vi "Text control 2 v6.1_pump-specific.vi"() -> ()   [LabVIEW 2016]
panel:
  in  "Tab Control":enum32{"Main", "Other parameters"}(tab)
  out "Line running":i32
  out "Total lines":i32
  out "Path":path=path "C:/users/rlp38/09Apr2009LTtesting/test2.txt"
  out "I vs Vg":cluster{"Y data in":dbl[], "X data in":dbl[]}[](graph)
  out "Is max":dbl format="%.2e"
  out "Id max":dbl format="%.2e"
  out "Ig max":dbl format="%.2e"
  out "Imax vs time":cluster{"Y data in":dbl[], "X data in":dbl[]}[](graph)
  out "Imin vs time":cluster{"Y data in":dbl[], "X data in":dbl[]}[](graph)
  out "I vs Vd":cluster{"Y data in":dbl[], "X data in":dbl[]}[](graph)
  in  "Script":string="#-------------------------------------------------------\n# SPM pump cleaning script\n#\n# Version 0.5\n# Author: Dimitrios Simatos\n# Last updated: 2018-01-05\n#-------------------------------------------------------\n# Description\n#\n# This script is designed to run the cleaning sequence of the SPM OEM pump.\n# This script needs to be run 4 times!\n#-------------------------------------------------------\n# Changes\n#\n# Placed initialization and hard stop commands in the beginning.\n#-------------------------------------------------------\n# Important points\n#\n# Never leave any liquid in the pump to dry after the experiments. If they dry, the residue may block the valve.\n# Always run the cleaning cycle after the experiments.\n# Use clockwise rotation when going up in valve port numbers and vice versa.\n#-------------------------------------------------------\n# Things to do before running the script\n#\n# Set time units to minutes.\n# Set filenames.\n# Replace the tubing, if necessary.\n#-------------------------------------------------------\n# Port connections\n#\n# Port 1: Waste\n# Port 2: Waste\n# Port 3: Various cleaning liquids\n# Port 4: Waste\n# Port 5: Waste\n# Port 6: Waste\n#\n# Between each of the 4 runs, the settings of Port 3 will change, according to the cleaning protocol.\n# The settings for Port 3 are:\n# 1st run: 1% v/v solution of sodium hypochlorite in ultrapure water\n# 2nd run: 0.1% w/v solution of sodium dodecyl sulfate in ultrapure water\n# 3rd run: Ultrapure water\n# 4th run: Waste (in air, not immersed in liquid)\n#-------------------------------------------------------\n# Cleaning protocol for the SPM OEM pump (from the manual)\n#\n# A cleaning procedure should be performed at the end of each day or in between two different experiments.\n# An effective cleaning can be performed in the following manner:\n# • Bleach solution to kill microorganisms\n# 1. Prepare a solution of 1% chlorine bleach and deionized water\n#    NOTE: Prepare a 1% v/v solution of sodium hypochlorite in deionized water\n# 2. Prepare a reservoir and place 1 tubing in the bleach solution and 5 tubings in a waste recipient\n# 3. Pick up the bleach solution through 1 port to entirely fill the syringe\n# 4. Sequentially output the syringe content through the remaining ports and throw it to the waste\n# 5. Repeat operation at least 2 times\n# • Detergent solution to remove debris\n# 1. Prepare a solution of 0.1% detergent and deionized water\n#    NOTE: Prepare a 0.1% w/v solution of sodium dodecyl sulfate in deionized water\n# 2. Move the tubing from the bleach solution reservoir and place it into a reservoir of detergent solution\n# 3. Pick up the detergent solution through 1 port to entirely fill the syringe\n# 4. Sequentially output the detergent solution through the remaining ports into the waste recipient\n# 5. Repeat operation at least 2 times\n# • Rinsing water to prepare the pump for your next experiment\n# 1. Move the tubing from the detergent solution reservoir and place it into a reservoir of deionized water\n# 2. Pick up the rinsing solution through 1 port to entirely fill the syringe\n# 3. Sequentially output the rinse water through the remaining ports into the waste recipient\n# 4. Repeat operation at least 2 times\n# • Replace the tubing, if necessary\n#-------------------------------------------------------\n# Pumping cycles and execution time\n#\n# Execution time for a single cycle: 6 x (1 min + 10 sec) = 7 minutes\n# Total execution time: 4 x 7 = 28 minutes\n# Since the script has to run 4 times, the cleaning lasts for: 4 x 28 = 112 minutes\n# Air must be the last to be pumped through the valve, to remove all liquids.\n# There are 4 pumping cycles. Each one draws a different liquid through port 3 and pumps it sequentially through ports 1,2,4,5,6.\n# During the sequential pumping, each port receives 200 ml of liquid (20% of the total syringe volume = 600 \"plunger units\")\n# The device must be disconnected from the port during the cleaning procedure.\n# All cycles are similar, except cycle 1 has the initialization command uncommented and the first report valve command commented.\n#-------------------------------------------------------\n# Volume of liquid needed\n#\n# Volume of liquid needed per cycle: 1 ml\n# Total volume of liquid needed per script run: 4 x 1 = 4 ml\n# Since the script has to run 4 times, the first 3 with different liquids, I need:\n# 4 ml of 1% v/v solution of sodium hypochlorite in ultrapure water\n# 4 ml of 0.1% w/v solution of sodium dodecyl sulfate in ultrapure water\n# 4 ml of ultrapure water\n#-------------------------------------------------------\n# Parameters\n#\n# Syringe size: 1 ml\n# Step resolution N = 0.01 mm\n# Drawing flow V = 300 pulses/second (6000 ul/min)\n# Pumping flow V = 300 pulses/second (6000 ul/min)\n#-------------------------------------------------------\n# Pump initialization\npump /1T #hard stop pump\npump /1ZR #initialize pump\n#-------------------------------------------------------\n# Cycle 1\n# Fill the syringe\npump /1Q #query pump\npump /1? #report absolute plunger position\n#pump /1?6 #report valve position\nwait-min 1 #wait 1 minute\npump /1N0R #set step resolution: 0.01 mm\npump /1Q #query pump\npump /1? #report absolute plunger position (the plunger should be at 0)\npump /1?6 #report valve position\nwait 1000 #wait 1 second\npump /1V300R #choose speed: 300 steps/s (6000 ul/min)\npump /1Q #query pump\nwait 1000 #wait 1 second\npump /1I3R #go to port 3, clockwise rotation\npump /1Q #query pump\npump /1?6 #report valve position\nwait 1000 #wait 1 second\npump /1A3000R #go to absolute position 3000 (= draw 1 ml)\nwait 30000 #wait 30 seconds\npump /1Q #query pump\npump /1? #report absolute plunger position (the plunger should have finished moving)\n#pump /1?6 #report valve position\n# The sequential pumping begins\n# Port 1\npump /1O1R #switch to port 1, counterclockwise rotation\npump /1Q #query pump\npump /1?6 #report valve position\npump /1A2400R #go to absolute position 2400 (= pump 200 ul)\npump /1Q #query pump\npump /1? #report absolute plunger position (the plunger should be moving to 0)\nwait-min 1 #wait 1 minute\npump /1? #report absolute plunger position (the plunger should have finished moving)\n# Port 2\npump /1I2R #switch to port 2, clockwise rotation\npump /1Q #query pump\npump /1?6 #report valve position\npump /1A1800R #go to absolute position 1800 (= pump 200 ul)\npump /1Q #query pump\npump /1? #report absolute plunger position (the plunger should be moving to 0)\nwait-min 1 #wait 1 minute\npump /1? #report absolute plunger position (the plunger should have finished moving)\n# Port 4\npump /1I4R #switch to port 4, clockwise rotation\npump /1Q #query pump\npump /1?6 #report valve position\npump /1A1200R #go to absolute position 1200 (= pump 200 ul)\npump /1Q #query pump\npump /1? #report absolute plunger position (the plunger should be moving to 0)\nwait-min 1 #wait 1 minute\npump /1? #report absolute plunger position (the plunger should have finished moving)\n# Port 5\npump /1I5R #switch to port 5, clockwise rotation\npump /1Q #query pump\npump /1?6 #report valve position\npump /1A600R #go to absolute position 600 (= pump 200 ul)\npump /1Q #query pump\npump /1? #report absolute plunger position (the plunger should be moving to 0)\nwait-min 1 #wait 1 minute\npump /1? #report absolute plunger position (the plunger should have finished moving)\n# Port 6\npump /1I6R #switch to port 6, clockwise rotation\npump /1Q #query pump\npump /1?6 #report valve position\npump /1A0R #go to absolute position 0 (= pump 200 ul)\npump /1Q #query pump\npump /1? #report absolute plunger position (the plunger should be moving to 0)\nwait-min 1 #wait 1 minute\npump /1? #report absolute plunger position (the plunger should have finished moving)\n#-------------------------------------------------------\n# Cycle 2\n# Fill the syringe\n#pump /1ZR #initialize pump\npump /1Q #query pump\npump /1? #report absolute plunger position\npump /1?6 #report valve position\nwait-min 1 #wait 1 minute\npump /1N0R #set step resolution: 0.01 mm\npump /1Q #query pump\npump /1? #report absolute plunger position (the plunger should be at 0)\npump /1?6 #report valve position\nwait 1000 #wait 1 second\npump /1V300R #choose speed: 300 steps/s (6000 ul/min)\npump /1Q #query pump\nwait 1000 #wait 1 second\npump /1O3R #go to port 3, counterclockwise rotation\npump /1Q #query pump\npump /1?6 #report valve position\nwait 1000 #wait 1 second\npump /1A3000R #go to absolute position 3000 (= draw 1 ml)\nwait 30000 #wait 30 seconds\npump /1Q #query pump\npump /1? #report absolute plunger position (the plunger should have finished moving)\n#pump /1?6 #report valve position\n# The sequential pumping begins\n# Port 1\npump /1O1R #switch to port 1, counterclockwise rotation\npump /1Q #query pump\npump /1?6 #report valve position\npump /1A2400R #go to absolute position 2400 (= pump 200 ul)\npump /1Q #query pump\npump /1? #report absolute plunger position (the plunger should be moving to 0)\nwait-min 1 #wait 1 minute\npump /1? #report absolute plunger position (the plunger should have finished moving)\n# Port 2\npump /1I2R #switch to port 2, clockwise rotation\npump /1Q #query pump\npump /1?6 #report valve position\npump /1A1800R #go to absolute position 1800 (= pump 200 ul)\npump /1Q #query pump\npump /1? #report absolute plunger position (the plunger should be moving to 0)\nwait-min 1 #wait 1 minute\npump /1? #report absolute plunger position (the plunger should have finished moving)\n# Port 4\npump /1I4R #switch to port 4, clockwise rotation\npump /1Q #query pump\npump /1?6 #report valve position\npump /1A1200R #go to absolute position 1200 (= pump 200 ul)\npump /1Q #query pump\npump /1? #report absolute plunger position (the plunger should be moving to 0)\nwait-min 1 #wait 1 minute\npump /1? #report absolute plunger position (the plunger should have finished moving)\n# Port 5\npump /1I5R #switch to port 5, clockwise rotation\npump /1Q #query pump\npump /1?6 #report valve position\npump /1A600R #go to absolute position 600 (= pump 200 ul)\npump /1Q #query pump\npump /1? #report absolute plunger position (the plunger should be moving to 0)\nwait-min 1 #wait 1 minute\npump /1? #report absolute plunger position (the plunger should have finished moving)\n# Port 6\npump /1I6R #switch to port 6, clockwise rotation\npump /1Q #query pump\npump /1?6 #report valve position\npump /1A0R #go to absolute position 0 (= pump 200 ul)\npump /1Q #query pump\npump /1? #report absolute plunger position (the plunger should be moving to 0)\nwait-min 1 #wait 1 minute\npump /1? #report absolute plunger position (the plunger should have finished moving)\n#-------------------------------------------------------\n# Cycle 3\n# Fill the syringe\n#pump /1ZR #initialize pump\npump /1Q #query pump\npump /1? #report absolute plunger position\npump /1?6 #report valve position\nwait-min 1 #wait 1 minute\npump /1N0R #set step resolution: 0.01 mm\npump /1Q #query pump\npump /1? #report absolute plunger position (the plunger should be at 0)\npump /1?6 #report valve position\nwait 1000 #wait 1 second\npump /1V300R #choose speed: 300 steps/s (6000 ul/min)\npump /1Q #query pump\nwait 1000 #wait 1 second\npump /1O3R #go to port 3, counterclockwise rotation\npump /1Q #query pump\npump /1?6 #report valve position\nwait 1000 #wait 1 second\npump /1A3000R #go to absolute position 3000 (= draw 1 ml)\nwait 30000 #wait 30 seconds\npump /1Q #query pump\npump /1? #report absolute plunger position (the plunger should have finished moving)\n#pump /1?6 #report valve position\n# The sequential pumping begins\n# Port 1\npump /1O1R #switch to port 1, counterclockwise rotation\npump /1Q #query pump\npump /1?6 #report valve position\npump /1A2400R #go to absolute position 2400 (= pump 200 ul)\npump /1Q #query pump\npump /1? #report absolute plunger position (the plunger should be moving to 0)\nwait-min 1 #wait 1 minute\npump /1? #report absolute plunger position (the plunger should have finished moving)\n# Port 2\npump /1I2R #switch to port 2, clockwise rotation\npump /1Q #query pump\npump /1?6 #report valve position\npump /1A1800R #go to absolute position 1800 (= pump 200 ul)\npump /1Q #query pump\npump /1? #report absolute plunger position (the plunger should be moving to 0)\nwait-min 1 #wait 1 minute\npump /1? #report absolute plunger position (the plunger should have finished moving)\n# Port 4\npump /1I4R #switch to port 4, clockwise rotation\npump /1Q #query pump\npump /1?6 #report valve position\npump /1A1200R #go to absolute position 1200 (= pump 200 ul)\npump /1Q #query pump\npump /1? #report absolute plunger position (the plunger should be moving to 0)\nwait-min 1 #wait 1 minute\npump /1? #report absolute plunger position (the plunger should have finished moving)\n# Port 5\npump /1I5R #switch to port 5, clockwise rotation\npump /1Q #query pump\npump /1?6 #report valve position\npump /1A600R #go to absolute position 600 (= pump 200 ul)\npump /1Q #query pump\npump /1? #report absolute plunger position (the plunger should be moving to 0)\nwait-min 1 #wait 1 minute\npump /1? #report absolute plunger position (the plunger should have finished moving)\n# Port 6\npump /1I6R #switch to port 6, clockwise rotation\npump /1Q #query pump\npump /1?6 #report valve position\npump /1A0R #go to absolute position 0 (= pump 200 ul)\npump /1Q #query pump\npump /1? #report absolute plunger position (the plunger should be moving to 0)\nwait-min 1 #wait 1 minute\npump /1? #report absolute plunger position (the plunger should have finished moving)\n#-------------------------------------------------------\n# Cycle 4\n# Fill the syringe\n#pump /1ZR #initialize pump\npump /1Q #query pump\npump /1? #report absolute plunger position\npump /1?6 #report valve position\nwait-min 1 #wait 1 minute\npump /1N0R #set step resolution: 0.01 mm\npump /1Q #query pump\npump /1? #report absolute plunger position (the plunger should be at 0)\npump /1?6 #report valve position\nwait 1000 #wait 1 second\npump /1V300R #choose speed: 300 steps/s (6000 ul/min)\npump /1Q #query pump\nwait 1000 #wait 1 second\npump /1O3R #go to port 3, counterclockwise rotation\npump /1Q #query pump\npump /1?6 #report valve position\nwait 1000 #wait 1 second\npump /1A3000R #go to absolute position 3000 (= draw 1 ml)\nwait 30000 #wait 30 seconds\npump /1Q #query pump\npump /1? #report absolute plunger position (the plunger should have finished moving)\n#pump /1?6 #report valve position\n# The sequential pumping begins\n# Port 1\npump /1O1R #switch to port 1, counterclockwise rotation\npump /1Q #query pump\npump /1?6 #report valve position\npump /1A2400R #go to absolute position 2400 (= pump 200 ul)\npump /1Q #query pump\npump /1? #report absolute plunger position (the plunger should be moving to 0)\nwait-min 1 #wait 1 minute\npump /1? #report absolute plunger position (the plunger should have finished moving)\n# Port 2\npump /1I2R #switch to port 2, clockwise rotation\npump /1Q #query pump\npump /1?6 #report valve position\npump /1A1800R #go to absolute position 1800 (= pump 200 ul)\npump /1Q #query pump\npump /1? #report absolute plunger position (the plunger should be moving to 0)\nwait-min 1 #wait 1 minute\npump /1? #report absolute plunger position (the plunger should have finished moving)\n# Port 4\npump /1I4R #switch to port 4, clockwise rotation\npump /1Q #query pump\npump /1?6 #report valve position\npump /1A1200R #go to absolute position 1200 (= pump 200 ul)\npump /1Q #query pump\npump /1? #report absolute plunger position (the plunger should be moving to 0)\nwait-min 1 #wait 1 minute\npump /1? #report absolute plunger position (the plunger should have finished moving)\n# Port 5\npump /1I5R #switch to port 5, clockwise rotation\npump /1Q #query pump\npump /1?6 #report valve position\npump /1A600R #go to absolute position 600 (= pump 200 ul)\npump /1Q #query pump\npump /1? #report absolute plunger position (the plunger should be moving to 0)\nwait-min 1 #wait 1 minute\npump /1? #report absolute plunger position (the plunger should have finished moving)\n# Port 6\npump /1I6R #switch to port 6, clockwise rotation\npump /1Q #query pump\npump /1?6 #report valve position\npump /1A0R #go to absolute position 0 (= pump 200 ul)\npump /1Q #query pump\npump /1? #report absolute plunger position (the plunger should be moving to 0)\nwait-min 1 #wait 1 minute\npump /1? #report absolute plunger position (the plunger should have finished moving)\n#-------------------------------------------------------"
  out "Command running:":string
  out "Serial port data":string
  out "Elapsed Time":dbl caption="Elapsed Time (s)"
  in  "Time Units":u16(ring)=1 items=["Seconds", "Minutes", "Hours"]
  in  "Time Offset":dbl caption="Set Start Time (s)"
  in  "Reset":bool
  in  "Auto Reset":bool
  in  "integration time":u32(slide) max=2 step=1 scale=0.0..2.0
  in  "Interrupt run":bool
  out "Absolute plunger position vs time":cluster{"Y data in":dbl[], "X data in":dbl[]}[](graph)
  out "Valve position vs time":cluster{"Y data in":dbl[], "X data in":dbl[]}[](graph)
  out "Is on":dbl format="%.2e"
  out "Id on":dbl format="%.2e"
  out "Ig on":dbl format="%.2e"
  out "Ion vs time":cluster{"Y data in":dbl[], "X data in":dbl[]}[](graph)
  out "Ioff vs time":cluster{"Y data in":dbl[], "X data in":dbl[]}[](graph)
  out "Ig min":dbl format="%.2e"
  out "Id min":dbl format="%.2e"
  out "Is min":dbl format="%.2e"
  out "Is off":dbl format="%.2e"
  out "Id off":dbl format="%.2e"
  out "Ig off":dbl format="%.2e"
  in  "Integration time (long)":dbl=0.32 min=0.04 max=2.0 step=0.02 format="%.2f"
  in  "Integration time (short)":dbl=0.0019 min=8e-05 max=0.0019 step=8e-05 format="%^.0e"
  in  "Gate: Compliance":dbl=0.001 format="%.8f"
  in  "Drain: Compliance":dbl=0.001 format="%.8f"
  in  "Hard stop pump":bool
  in  "Halt pump":bool
  in  "Gate Range\nmode":u16(ring) items=["Auto", "Limited", "Fixed"]
  in  "Gate Range":u8(slide)=6 max=11 scale=0.0..11.0
  in  "Source/Drain\nRange mode":u16(ring) items=["Auto", "Limited", "Fixed"]
  in  "Source/Drain Range":u8(slide)=6 max=11 scale=0.0..11.0
  in  "Panel Controls":T1={"Emergency Stop"=refnum, "TransGraph Max"=1e-05, "Text/Graph (text=false)"=TRUE} {"TransGraph Max" format="%.2e"}
  in  "Panel Controls 2":T2={"Emergency Stop"=refnum, "TransGraph Max"=1e-05, "Text/Graph (text=false)"=TRUE, "TransGraph Min"=1e-11} {"TransGraph Min" format="%.2e"; "TransGraph Max" format="%.2e"}
  in  "SMU4":cluster{"on/off":bool, "Voltage":dbl} {"Voltage" min=-100.0 max=100.0 format="%.2f"}
  in  "Full Reset":bool
  in  "Standby":T3
  out "error out":errorcluster
  in  "Delay before read (ms)":u32=1000
  in  "byte count":u32=64
  in  "Serial End Mode for Reads":u16(ring)=2 items=["None", "LastBit", "TermChar"]
  in  "Timeout (ms)":u32=10000
  in  "Enable Termination\nChar (T)":bool=TRUE
  in  "Termination char\n(0xA = '\\n' = LF)\n(0xD = '\\r' = CR)":u8=13 format="%.0x"
  in  "flow control":u16(ring) items=["None"=0, "XON/XOFF"=1, "RTS/CTS"=2, "DTR/DSR"=4]
  in  "stop bits":u16(ring)=10 items=["1.0"=10, "1.5"=15, "2.0"=20]
  in  "parity":u16(ring) items=["None", "Odd", "Even", "Mark", "Space"]
  in  "data bits":u16=8 min=5 max=8 step=1
  in  "VISA resource name":refnum<visa-resource-name>="COM6"
  in  "baud rate":u32=9600
  in  "Filename (variable part)":string="step_1_up-H2O_initial_"
  in  "Suffix (script)":string="step_1_up-H2O_initial_script.txt"
  out "Timings Indicator":T4
  in  "Timings (overwritten by the Front Panel)":T5={"integration time"=0, "Short/Long integration time"=0.00064, "hold time (sec)"=0.0, "delay time (sec)"=0.0, "Step Time (0 disables)"=0.0, "sweep method"=0, "Pulse period"=0.005, "Base voltage"=0.0, "Pulse width"=0.0005} {"Pulse width" min=0.0005 max=0.1 step=0.0001 format="%.4f"; "Base voltage" format="%^.4e"; "Pulse period" min=0.005 max=1.0 step=0.0001 format="%.4f"; "sweep method" items=["Continuous", "Pulsed"]; "Step Time (0 disables)" format="%.2f"; "delay time (sec)" format="%.4f"; "hold time (sec)" format="%.4f"; "Short/Long integration time" format="%^.0e"; "integration time" scale=0.0..2.0}
  in  "Gate":T6={"Gate Start"=0.0, "Gate Stop"=2.0, "Gate Step (linear only)"=1.0, "Gate Compliance"=0.0001, "Gate PComp"=0.0, "Range mode"=0, "Range"=6} {"Range" max=11 scale=0.0..11.0; "Range mode" items=["Auto", "Limited", "Fixed"]; "Gate PComp" format="%^.2e"; "Gate Compliance" format="%^.2e"; "Gate Step (linear only)" format="%^.4e"; "Gate Stop" format="%^.4e"; "Gate Start" format="%^.4e"}
  in  "Drain 2":T7={"Drain Start"=0.0, "Drain Stop"=2.0, "Drain Compliance"=0.0001, "Drain Step"=1.0, "Drain PComp"=0.0, "Range mode"=0, "Range"=6} {"Range" max=11 scale=0.0..11.0; "Range mode" items=["Auto", "Limited", "Fixed"]; "Drain PComp" format="%^.2e"; "Drain Step" format="%^.4e"; "Drain Compliance" format="%^.2e"; "Drain Stop" format="%^.4e"; "Drain Start" format="%^.4e"}
  # "Syntax:\nitime [s|m|l] time(sec): [s|m|l] determines the integration time setting (small|medium|long) and time sets the value.\nNOTE: The value of the integration time has to be within the range allowed by its category (s|m|l), otherwise, the closest value will be used. (e.g. if the category is set to short but the time value is very long, the actual value used will be the maximum short integration time.\nIntegration times:\n    Short: Default: 640 us. Range: 8E-5 - 1.92E-3 seconds.\n    Medium: Fixed at 1 NPL cycle (0.02 seconds).\n    Long: Default: 16 NPL cycles (0.32 seconds). Range: 2-100 NPL cycles (0.04 seconds - 2 seconds).\ngaterangemode [a|l|f]\ndrainrangemode [a|l|f]\npulsed [on|off] PulsePeriod(sec) PulseBaseVoltage PulseONWidth(sec)\nstandby [on l off]\nwait NumMilliseconds\nwait-min NumMinutes\n# texthere = comment\ntransfer [s|d] VgStart VgStop VgStep VdStart VdStop VdStep\noutput [s|d] VgStart VgStop VgStep VdStart VdStop VdStep\nsample Vg Vd NumSamples Time(s) SampleInterval(s)\nsamplei Idg NumSamples Time(s) SampleInterval(s) VDGcompliance\n100 samples is approximately 13 seconds with medium integration\n# if in doubt use SampleInterval(s) = 0.004\nstressV VG VD IGcompliance IDcompliance Duration(sec)\nstressI IDG VDGcompliance Duration(sec)\nvsu2pulse Bias Duration(s)\npulsedstressV [s|d] VEstop VgON VgOFF Period(s) PulseONwidth(s) Vd\nsample-fpp Vg Vd NumSamples Time\nresample-fpp Vg Vd\ntransfer-fpp [s|d] VgStart VgStop VgStep VdStart VdStop VdStep\noutput-fpp [s|d] VgStart VgStop VgStep VdStart VdStop VdStep\nserial SerialPortCommand\npump SerialPortCommand for the SPM pump\n\nSPM Pump Syntax (<x>: pump number, use 1 if only one pump):\nif the command syntax contains [R], then append the letter R to the command\n/<x>Q: query (a query command should follow each command)\n/<x>Z[R] or /<x>Y[R]: initialize pump\n/<x>N<n>[R] (<n>=0,1): <0> (<1>) microstep 0.01 mm (0.00125 mm) resolution\n/<x>I<n> (<n>=0-6): turn to port number n (clockwise)\n/<x>O<n> (<n>=0-6): turn to port number n (counterclockwise)\n/<x>X: Re-execute last command string\n/<x>G<n>[R] (<n>=0-60000): repeat command sequence (default: 0, 0=loop forever)\n/<x>g: Mark the start of a repeat sequence (max = 10)\n/<x>M<n>[R] (<n>=0-86400000): delay command execution by n milliseconds\n/<x>H: Halt; Pause the sequence after finishing the current move\n/<x>T: Hardstop; Interrupt the current move and suppress it from the sequence\n/<x>A<n>[R] (<n>=0-3000 with N=0, 0-24000 with N=1): absolute position\n/<x>P<n>[R] (<n>=0-3000 with N=0, 0-24000 with N=1): relative pickup\n/<x>D<n>[R] (<n>=0-3000 with N=0, 0-24000 with N=1): relative dispense\n/<x>V<n>[R] (<n>=1-1600 default: 150): set peak speed (pulses/sec)\nNOTE: The lowest speed limit is 1 pulse/sec, not 5, as the manual states.\n/<x>S<n>[R] (<n>=10-40 default: 22): set speed (NOT in pulses/sec, look in manual)\nNOTE: When controlled with absolute position, one does not need to pay special attention to the syringe that is mounted on the pump.\nWithdraw from lower stage (ports 3, 5), dispense from higher stage (ports 2, 4, 6).\nConnect Port 1 to waste."
  # "Time"
  # "1\n2\n3\n4\n5\n6\n7\n8\n9\n10\n11\n12\n13\n14\n15\n16\n17\n18\n19\n20"
  # "Serial port settings"
  # "Filename settings"
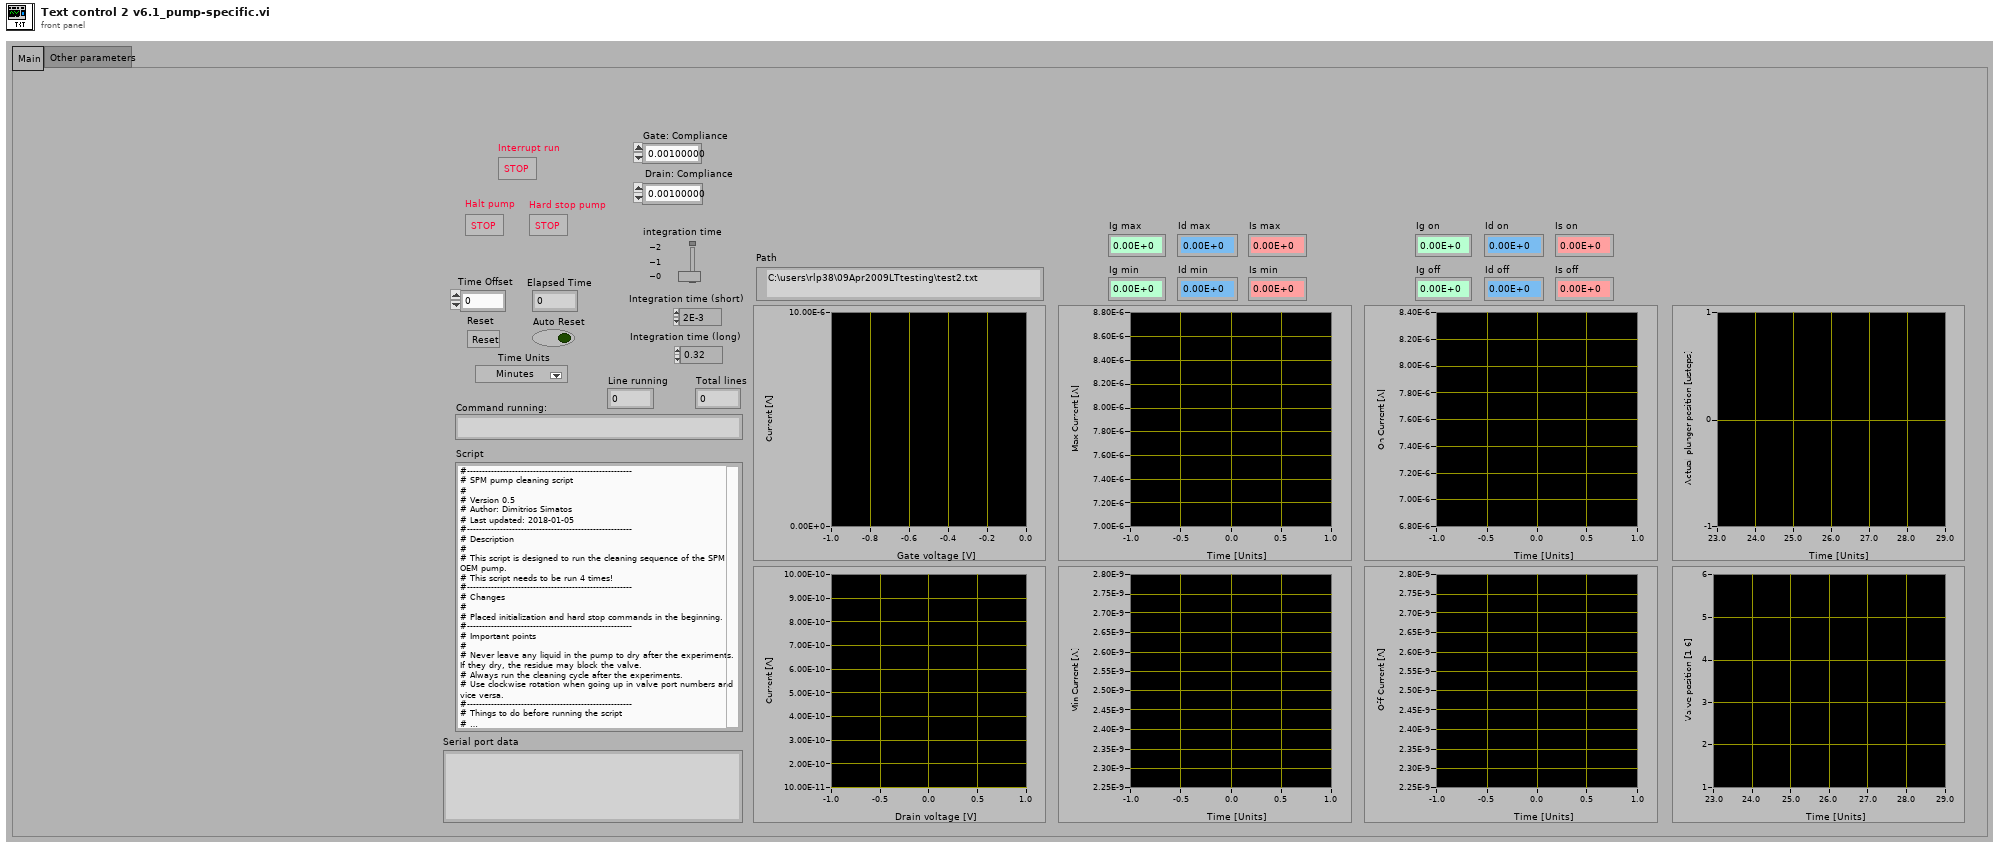
[diagram p1: front panel]
types:
  T1 = cluster{"Emergency Stop":refnum<vi>, "TransGraph Max":dbl, "Text/Graph (text=false)":bool}
  T2 = cluster{"Emergency Stop":refnum<vi>, "TransGraph Max":dbl, "Text/Graph (text=false)":bool, "TransGraph Min":dbl}
  T3 = cluster{"Gate Standby":bool, "Drain Standby":bool}
  T4 = cluster{"integration time (0:s, 1:m, 2:l)":u32, "Short/Long integration time":dbl, "hold time (sec)":dbl, "delay time (sec)":dbl, "Step Time (0 disables)":dbl, "sweep method":u16, "Pulse period":dbl, "Base voltage":dbl, "Pulse width":dbl}
  T5 = cluster{"integration time":u32, "Short/Long integration time":dbl, "hold time (sec)":dbl, "delay time (sec)":dbl, "Step Time (0 disables)":dbl, "sweep method":u16, "Pulse period":dbl, "Base voltage":dbl, "Pulse width":dbl}
  T6 = cluster{"Gate Start":dbl, "Gate Stop":dbl, "Gate Step (linear only)":dbl, "Gate Compliance":dbl, "Gate PComp":dbl, "Range mode":u16, "Range":u8}
  T7 = cluster{"Drain Start":dbl, "Drain Stop":dbl, "Drain Compliance":dbl, "Drain Step":dbl, "Drain PComp":dbl, "Range mode":u16, "Range":u8}
  T8 = enum16{"open", "replace", "create", "open or create", "replace or create", "replace or create with confirmation"}
  T9 = cluster{"V2 Start":dbl, "V2 Step":dbl, "Number of points":i32}
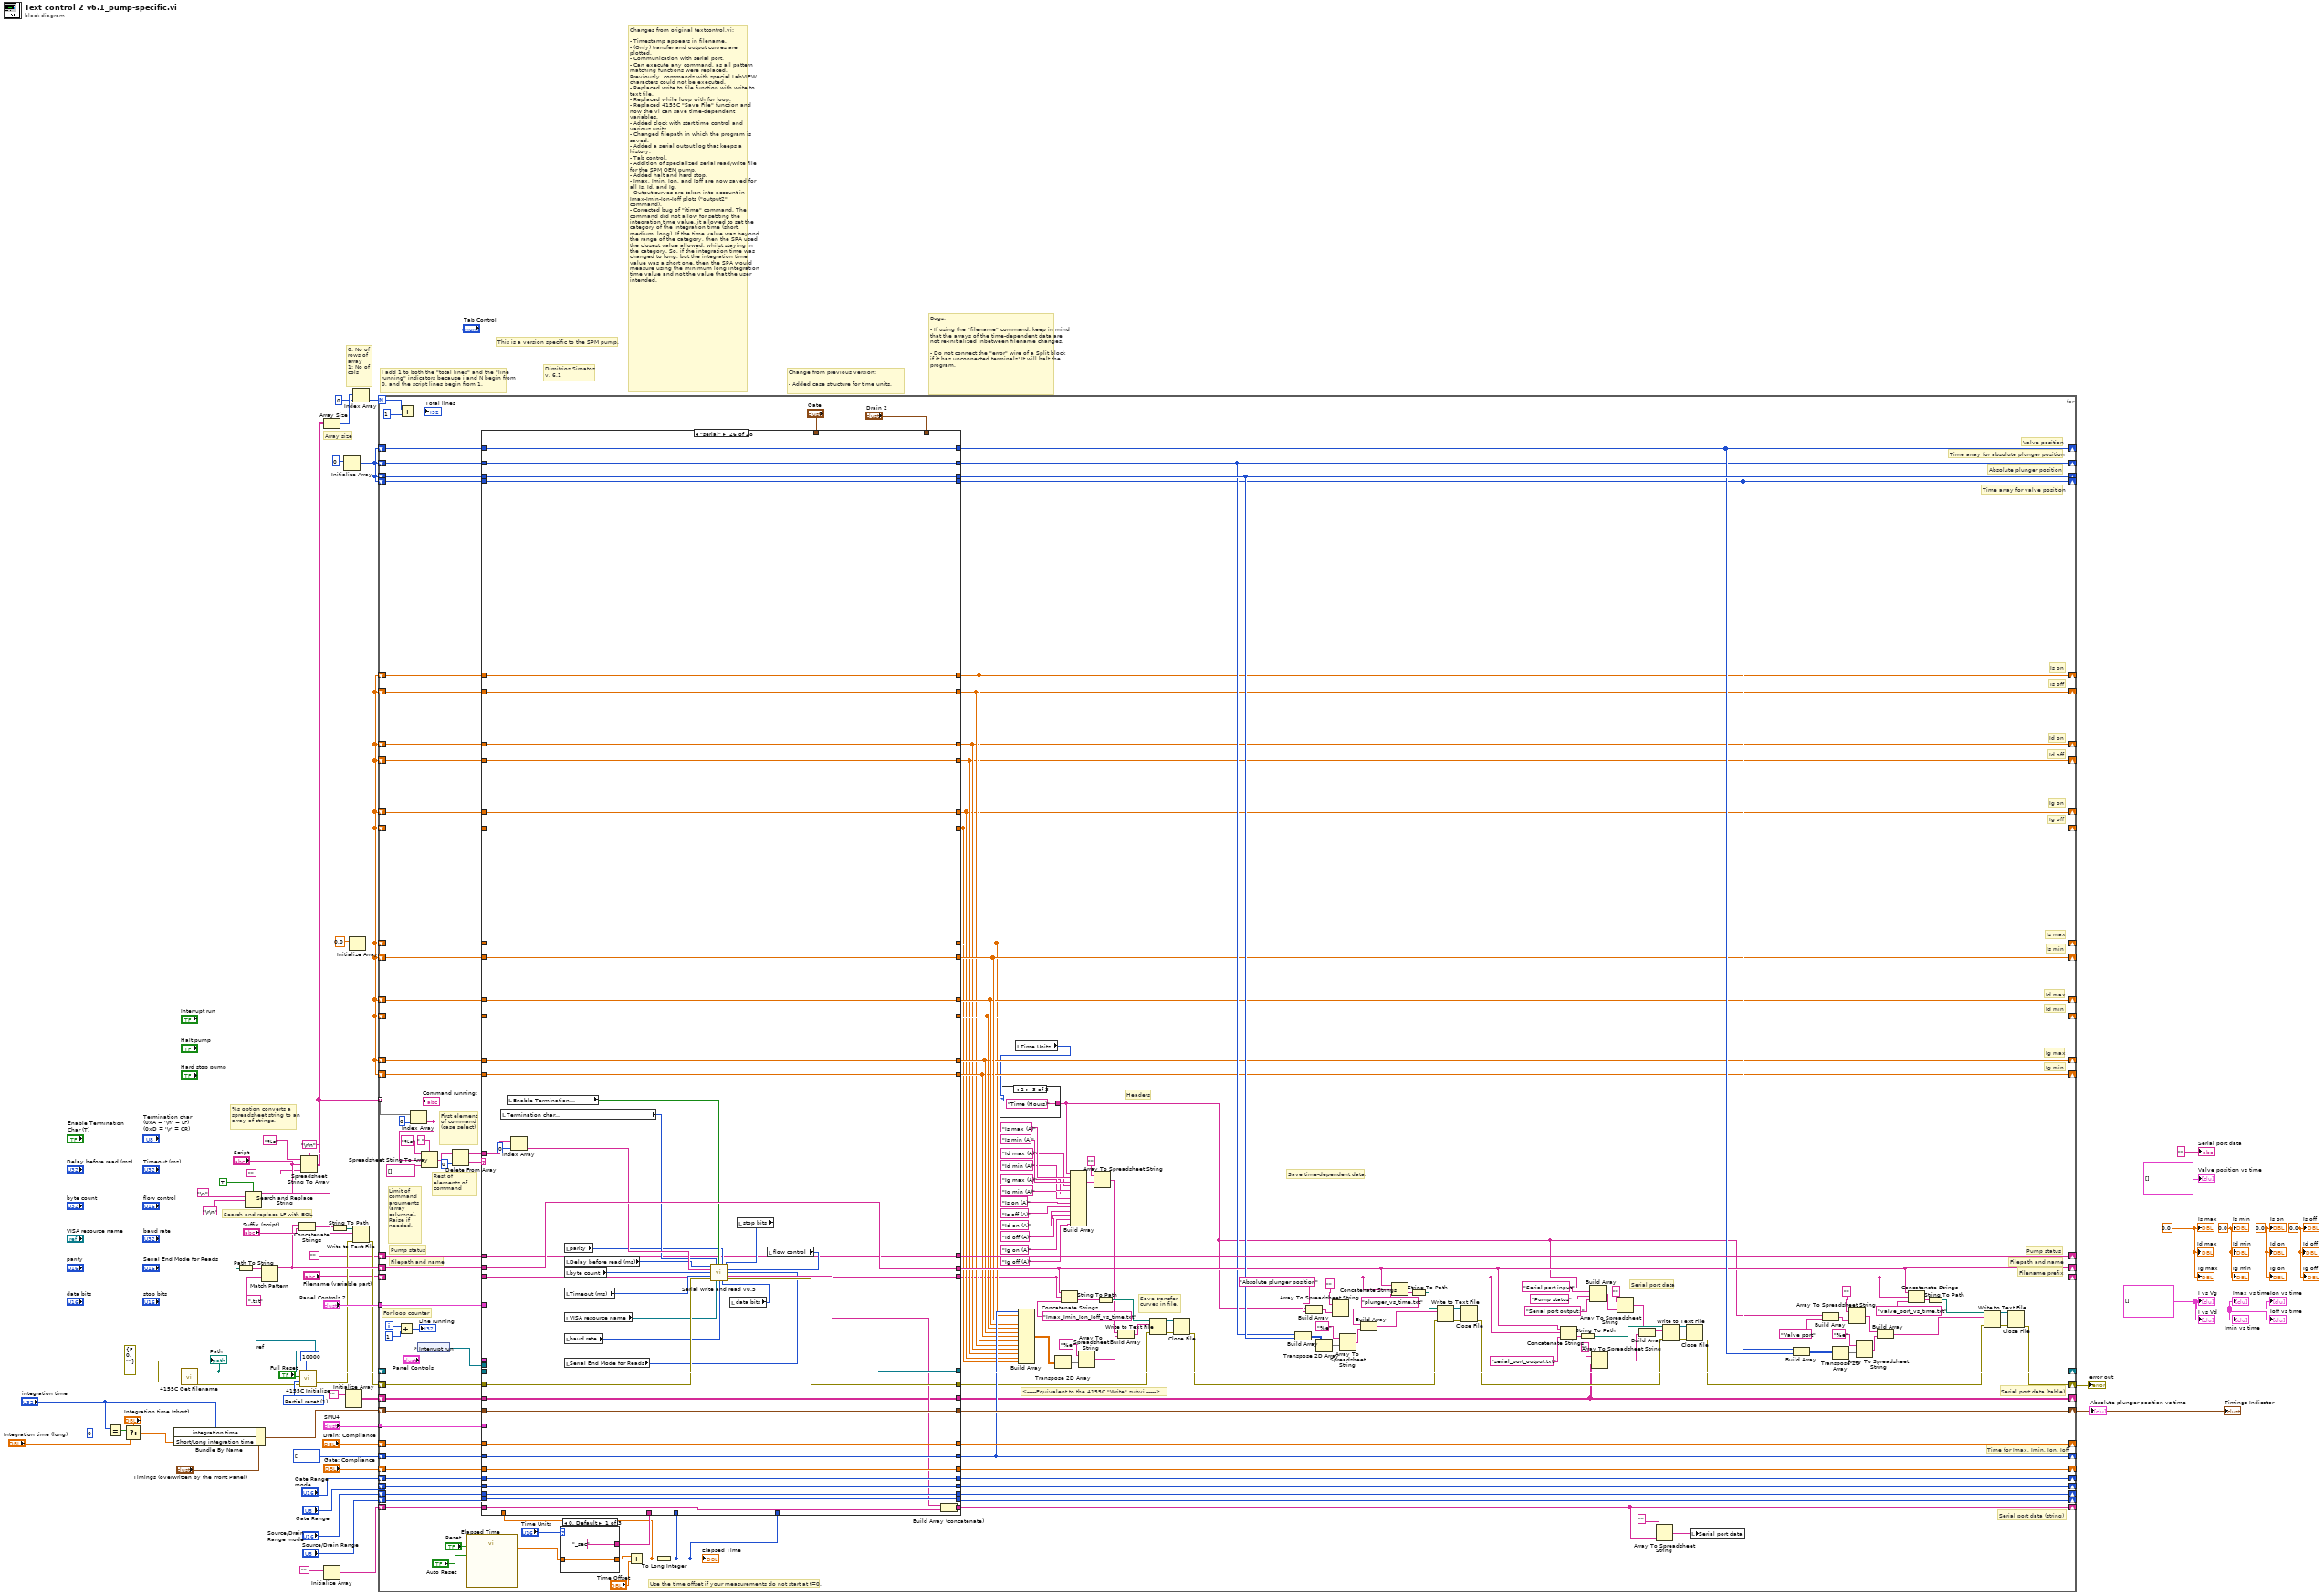
[diagram p0: block diagram]
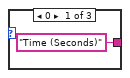
[diagram p2: hidden frame]
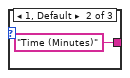
[diagram p3: hidden frame]
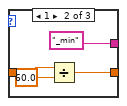
[diagram p4: hidden frame]
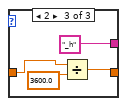
[diagram p5: hidden frame]
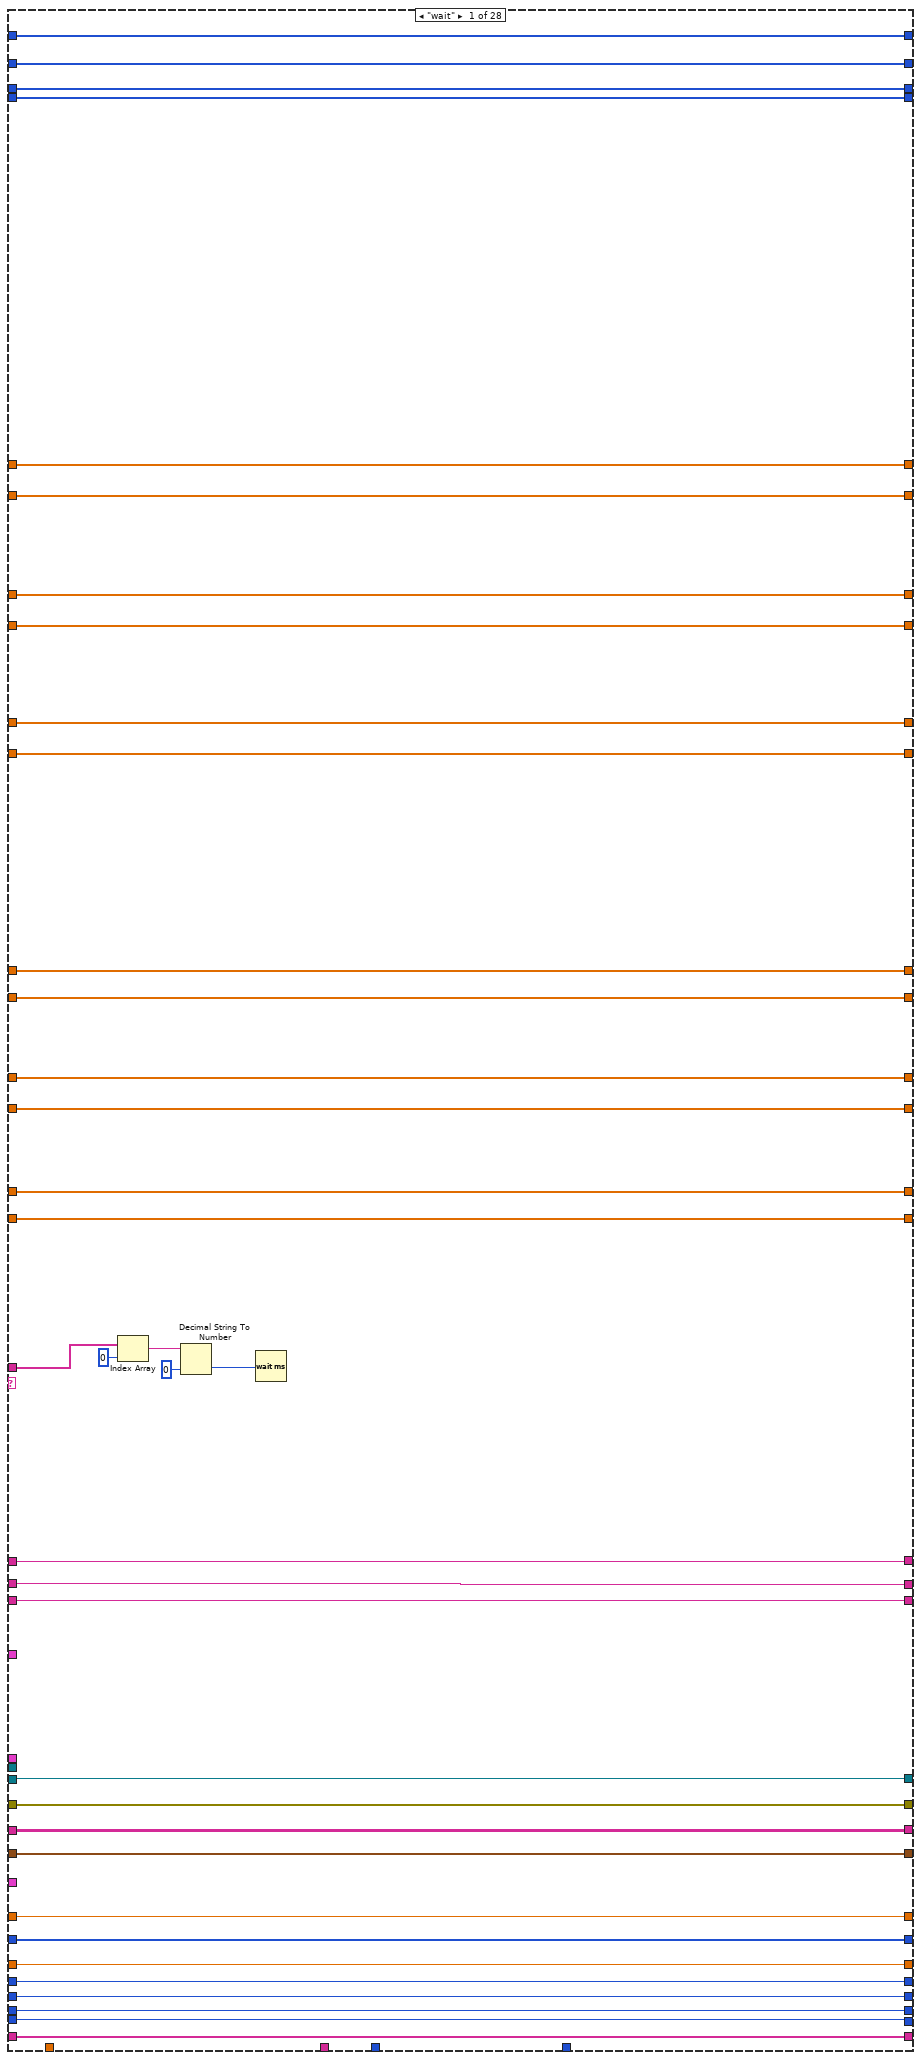
[diagram p6: hidden frame]
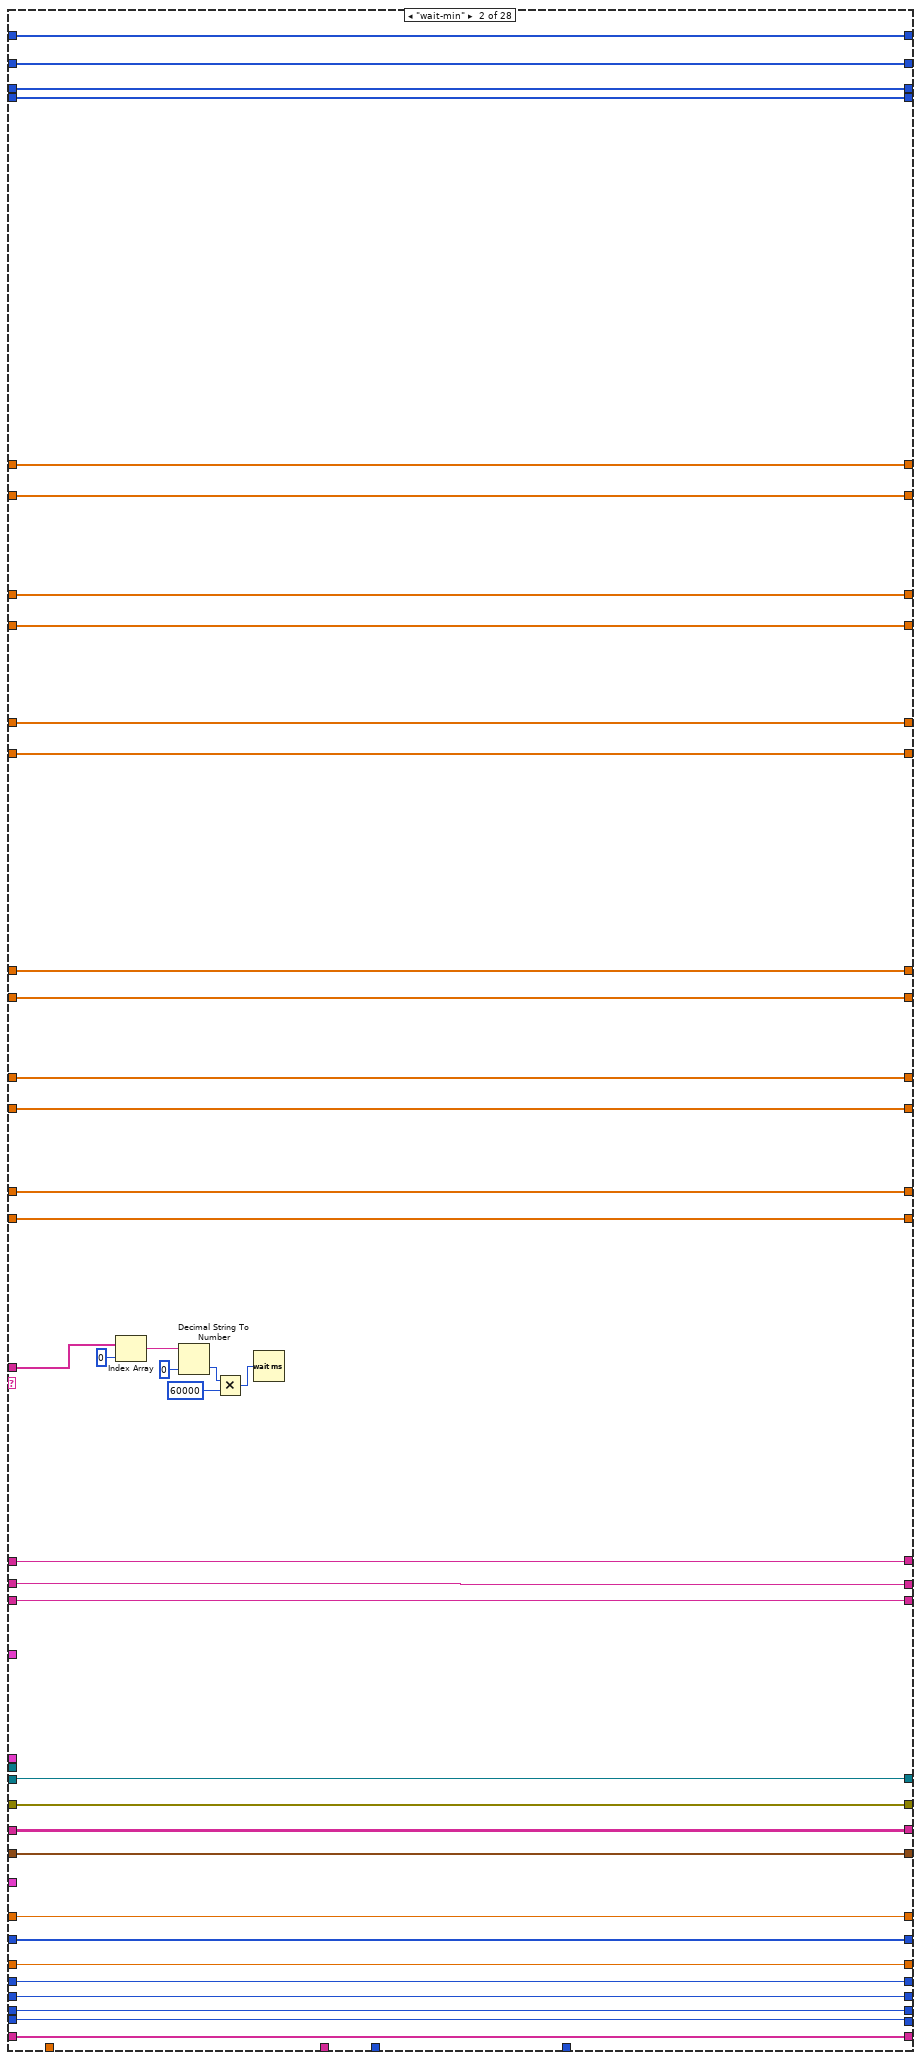
[diagram p7: hidden frame]
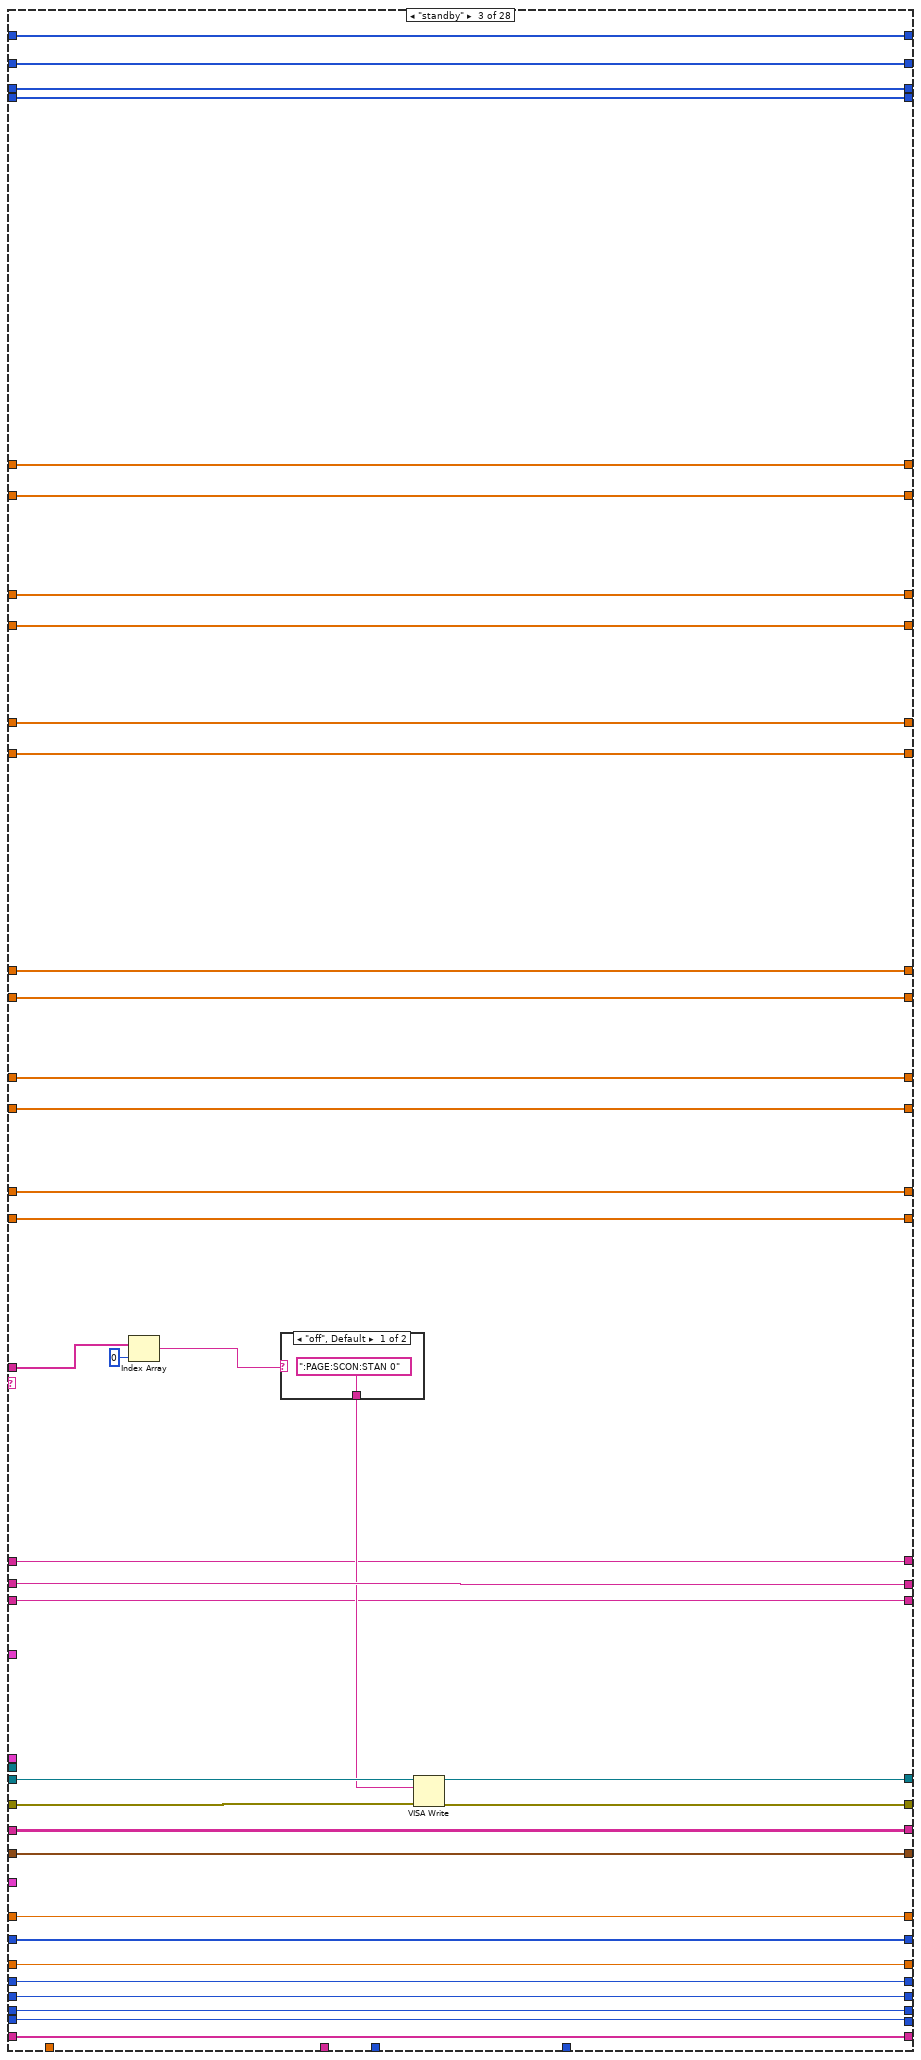
[diagram p8: hidden frame]
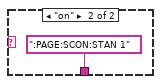
[diagram p9: hidden frame]
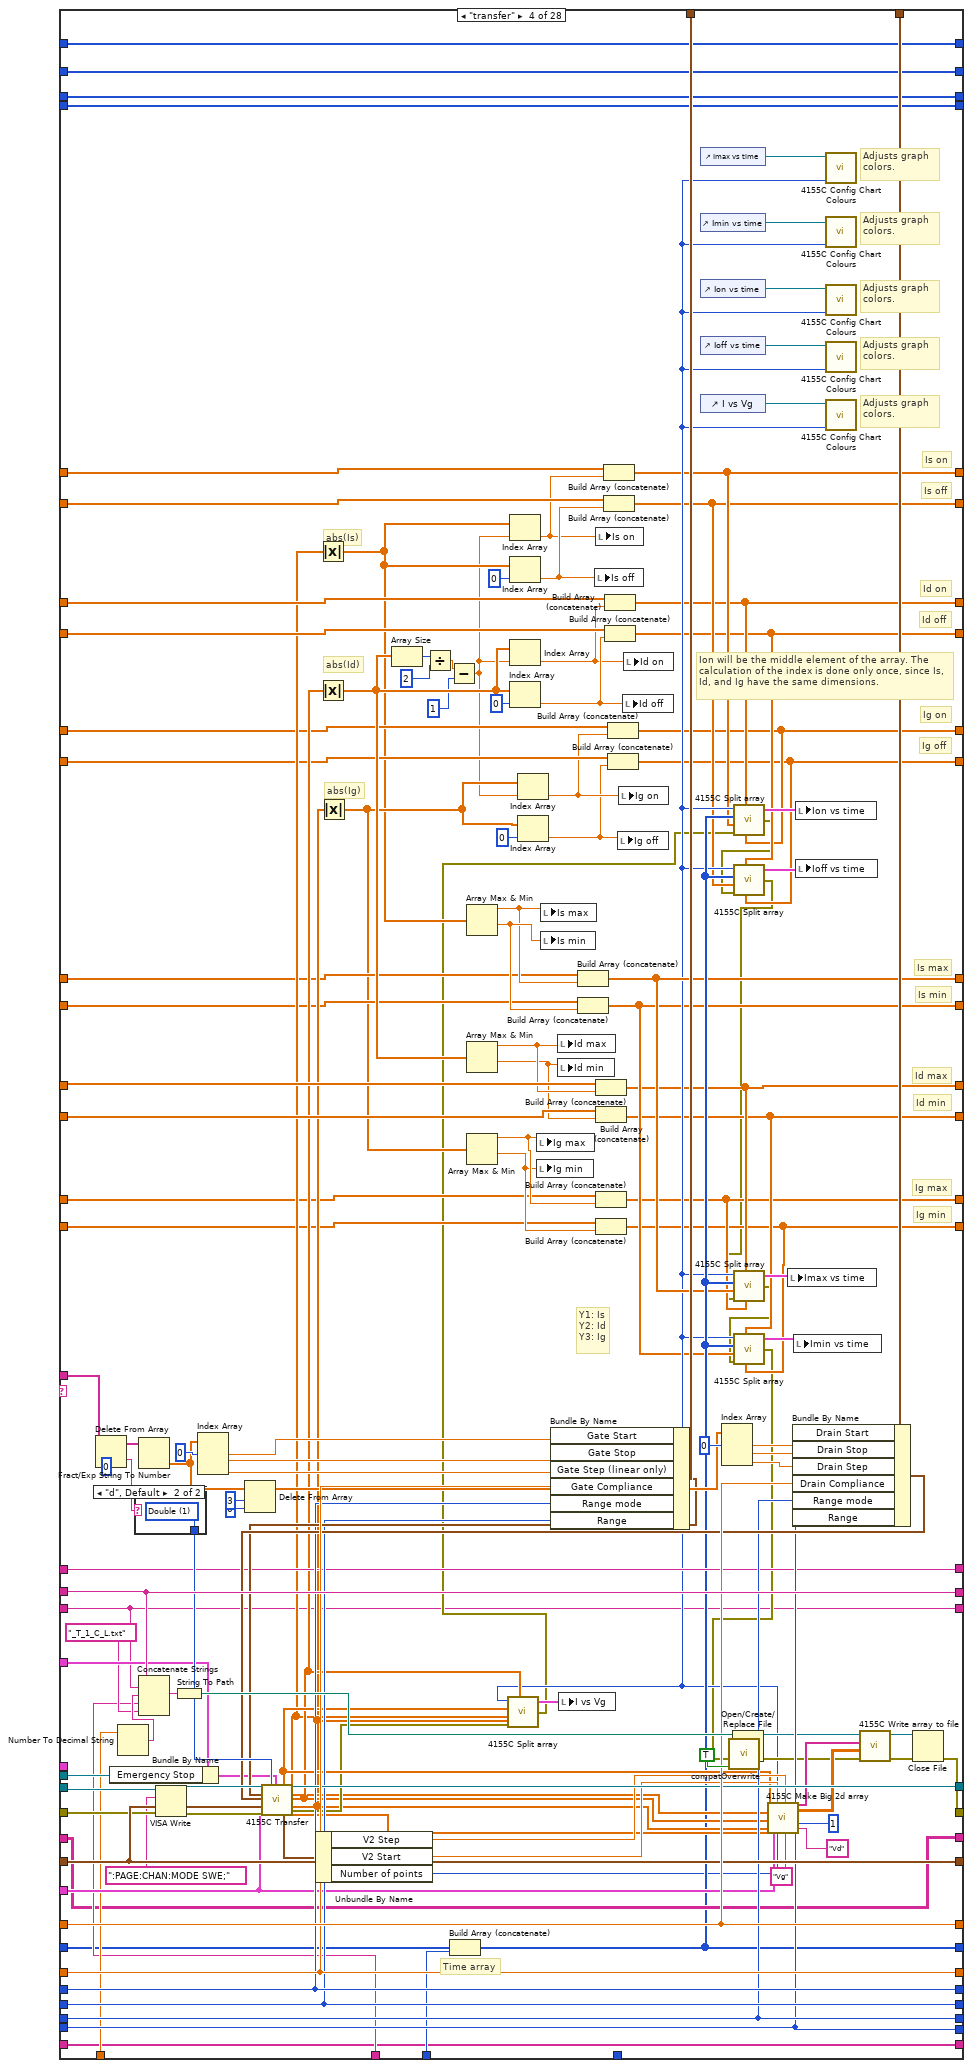
[diagram p10: hidden frame]
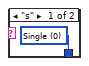
[diagram p11: hidden frame]
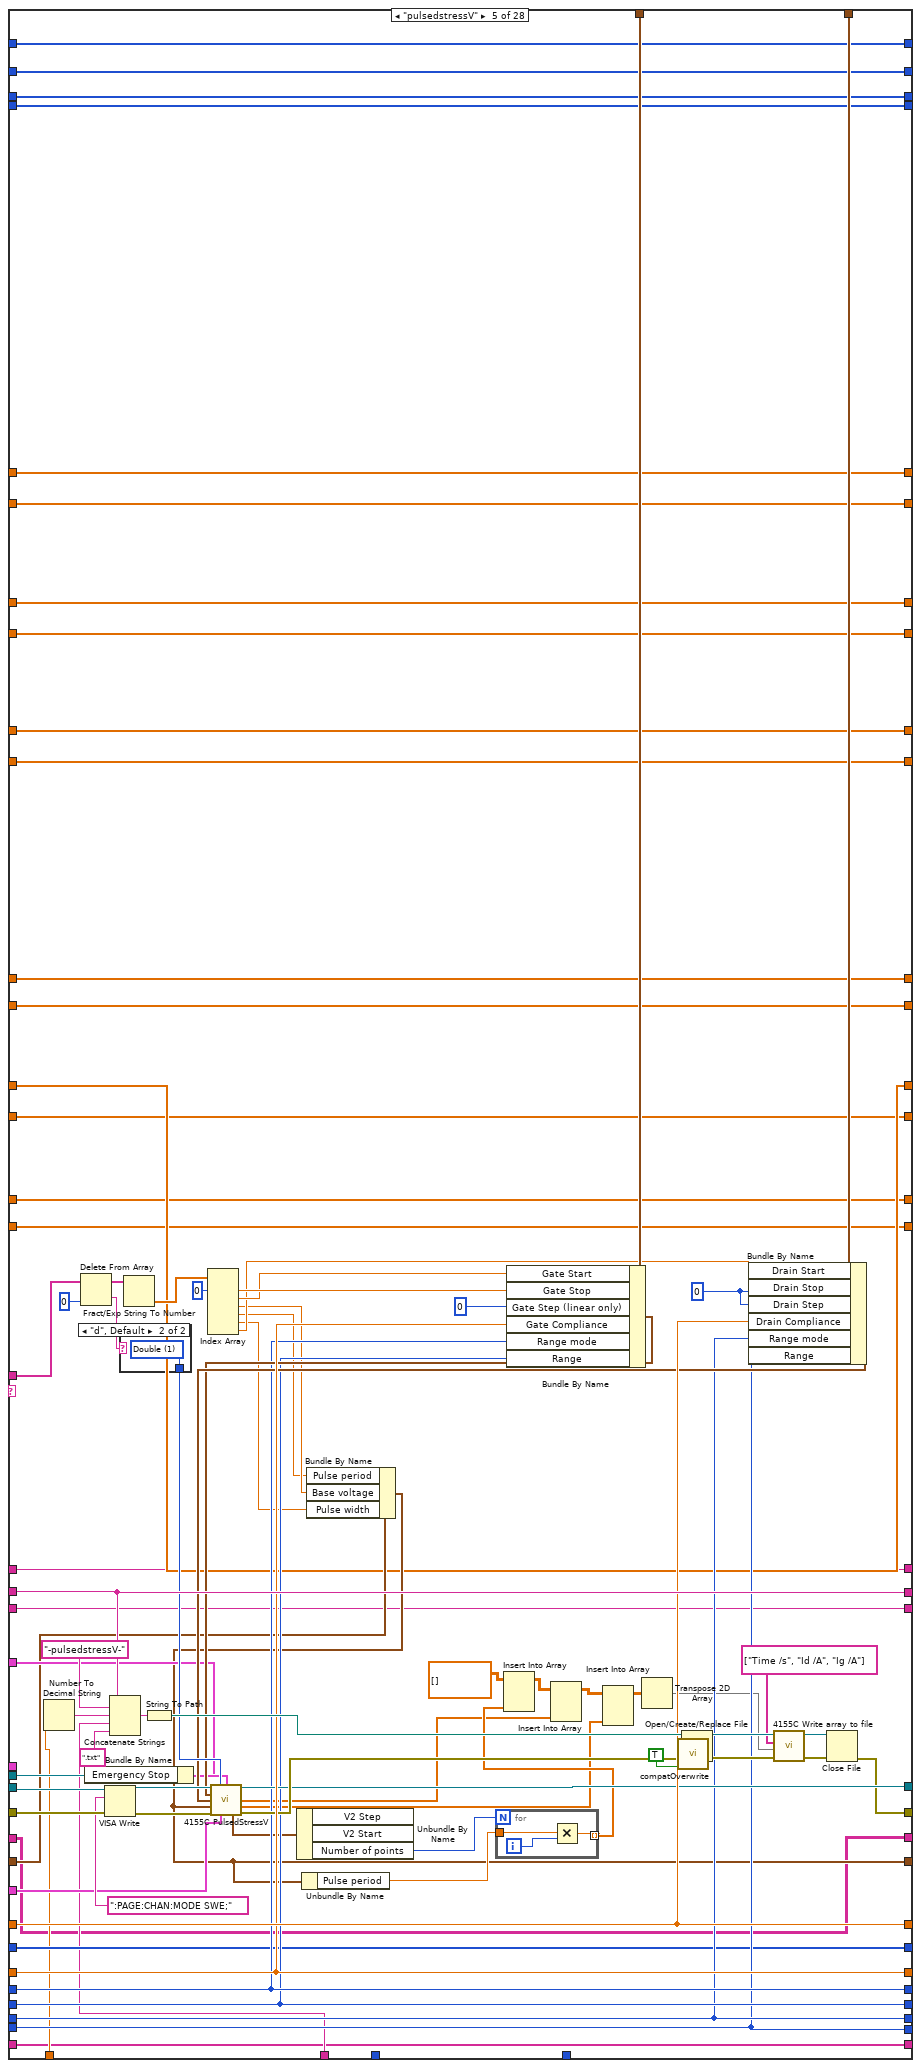
[diagram p12: hidden frame]
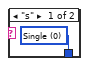
[diagram p13: hidden frame]
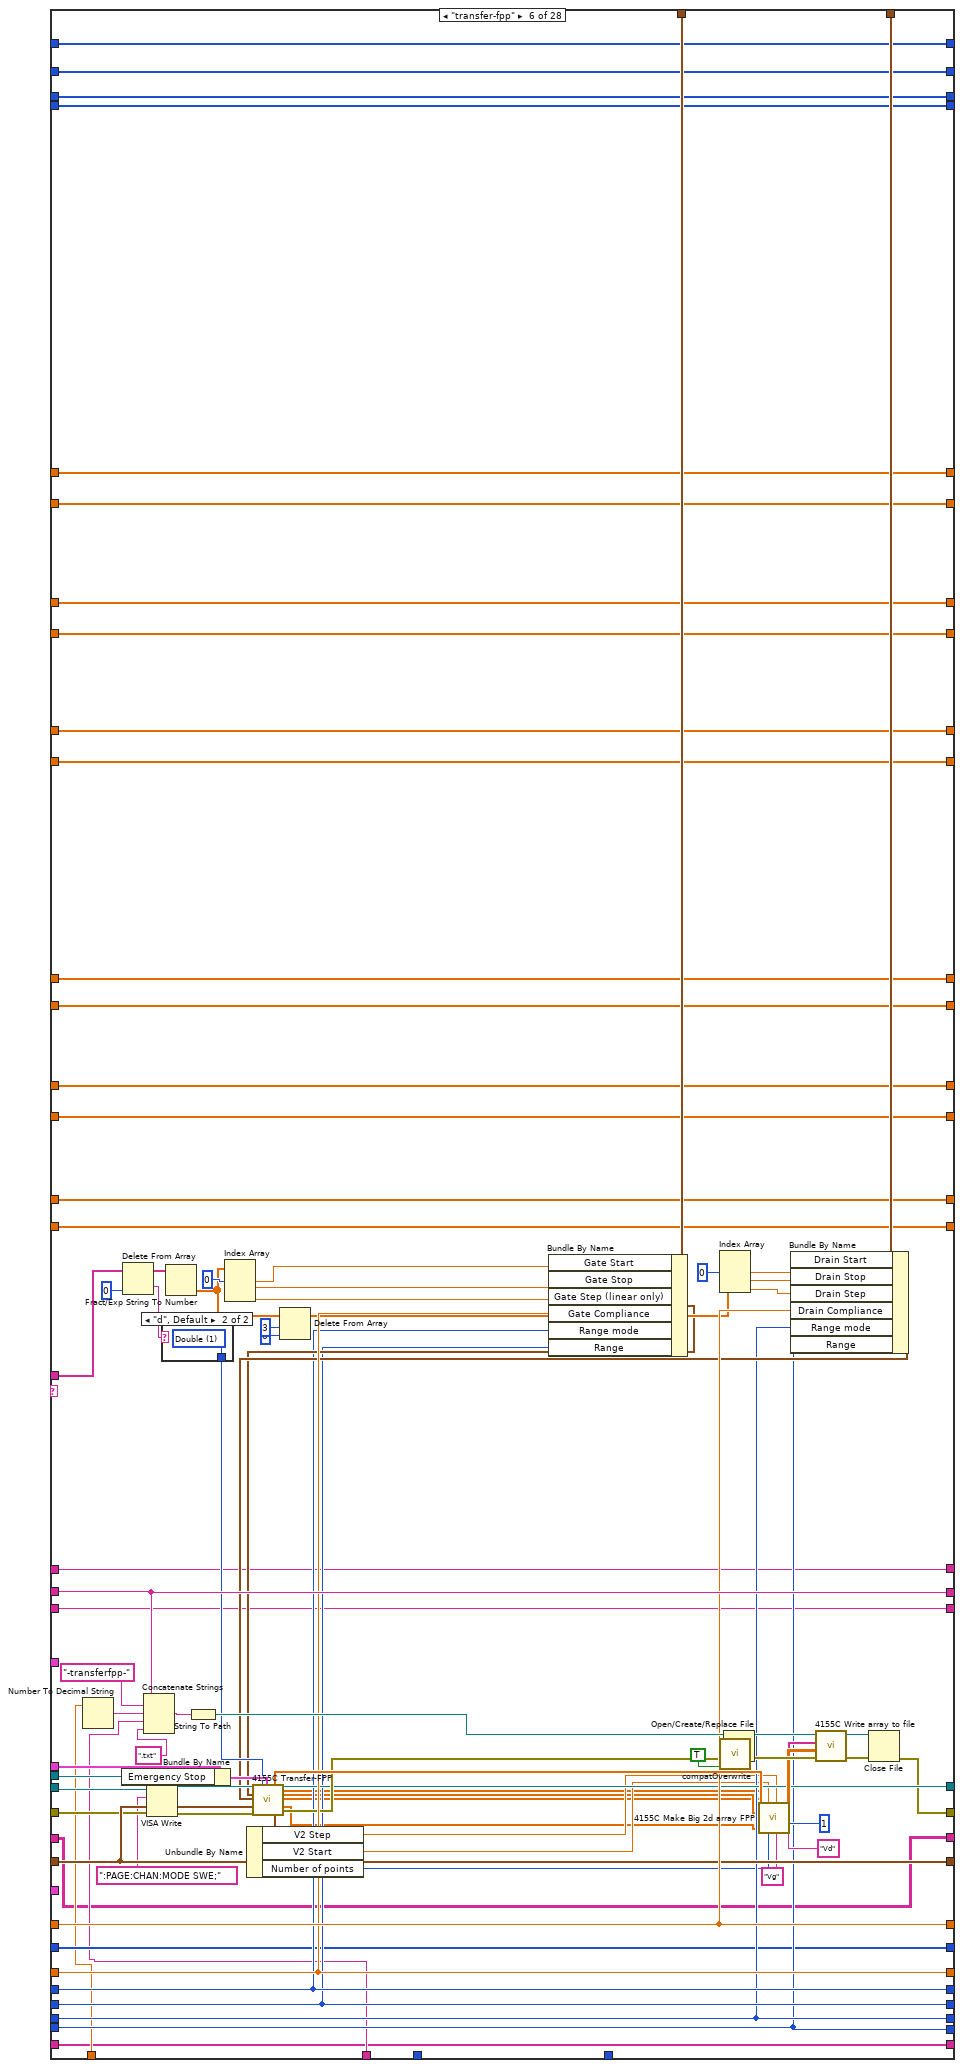
[diagram p14: hidden frame]
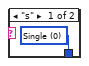
[diagram p15: hidden frame]
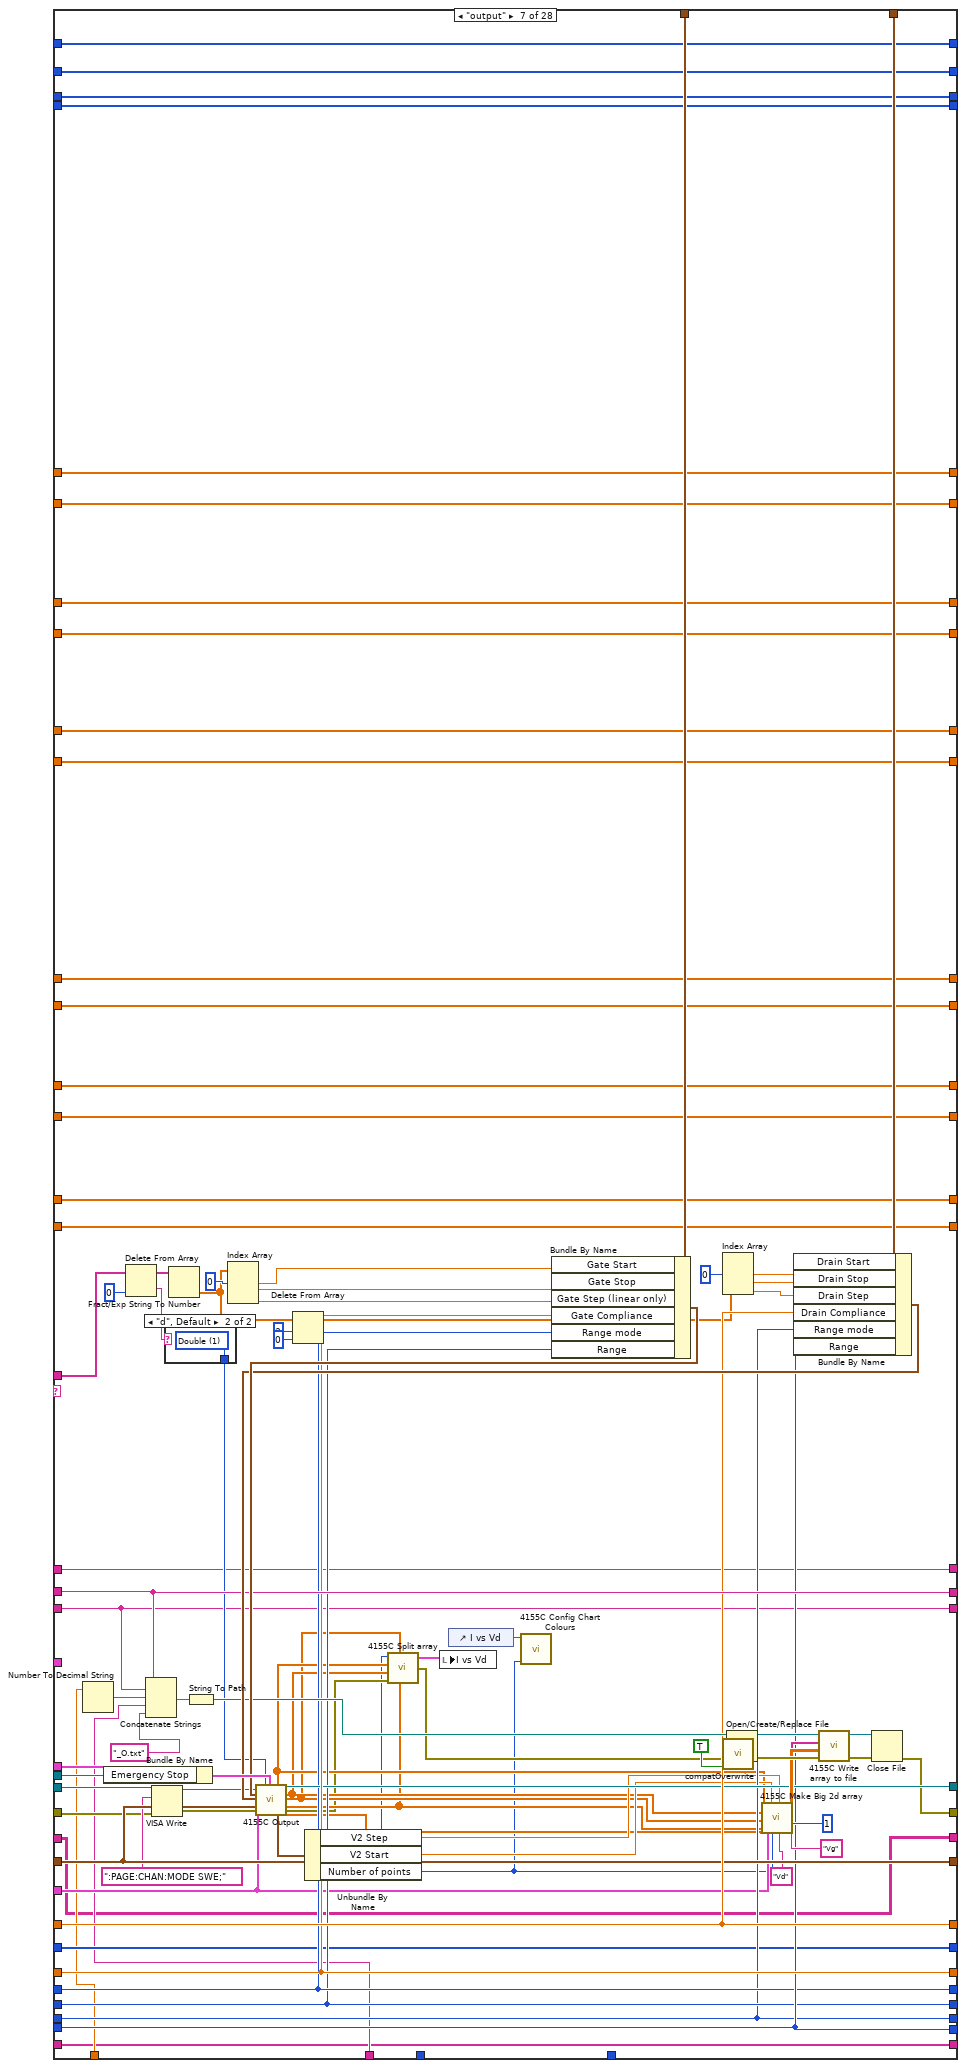
[diagram p16: hidden frame]
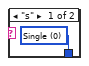
[diagram p17: hidden frame]
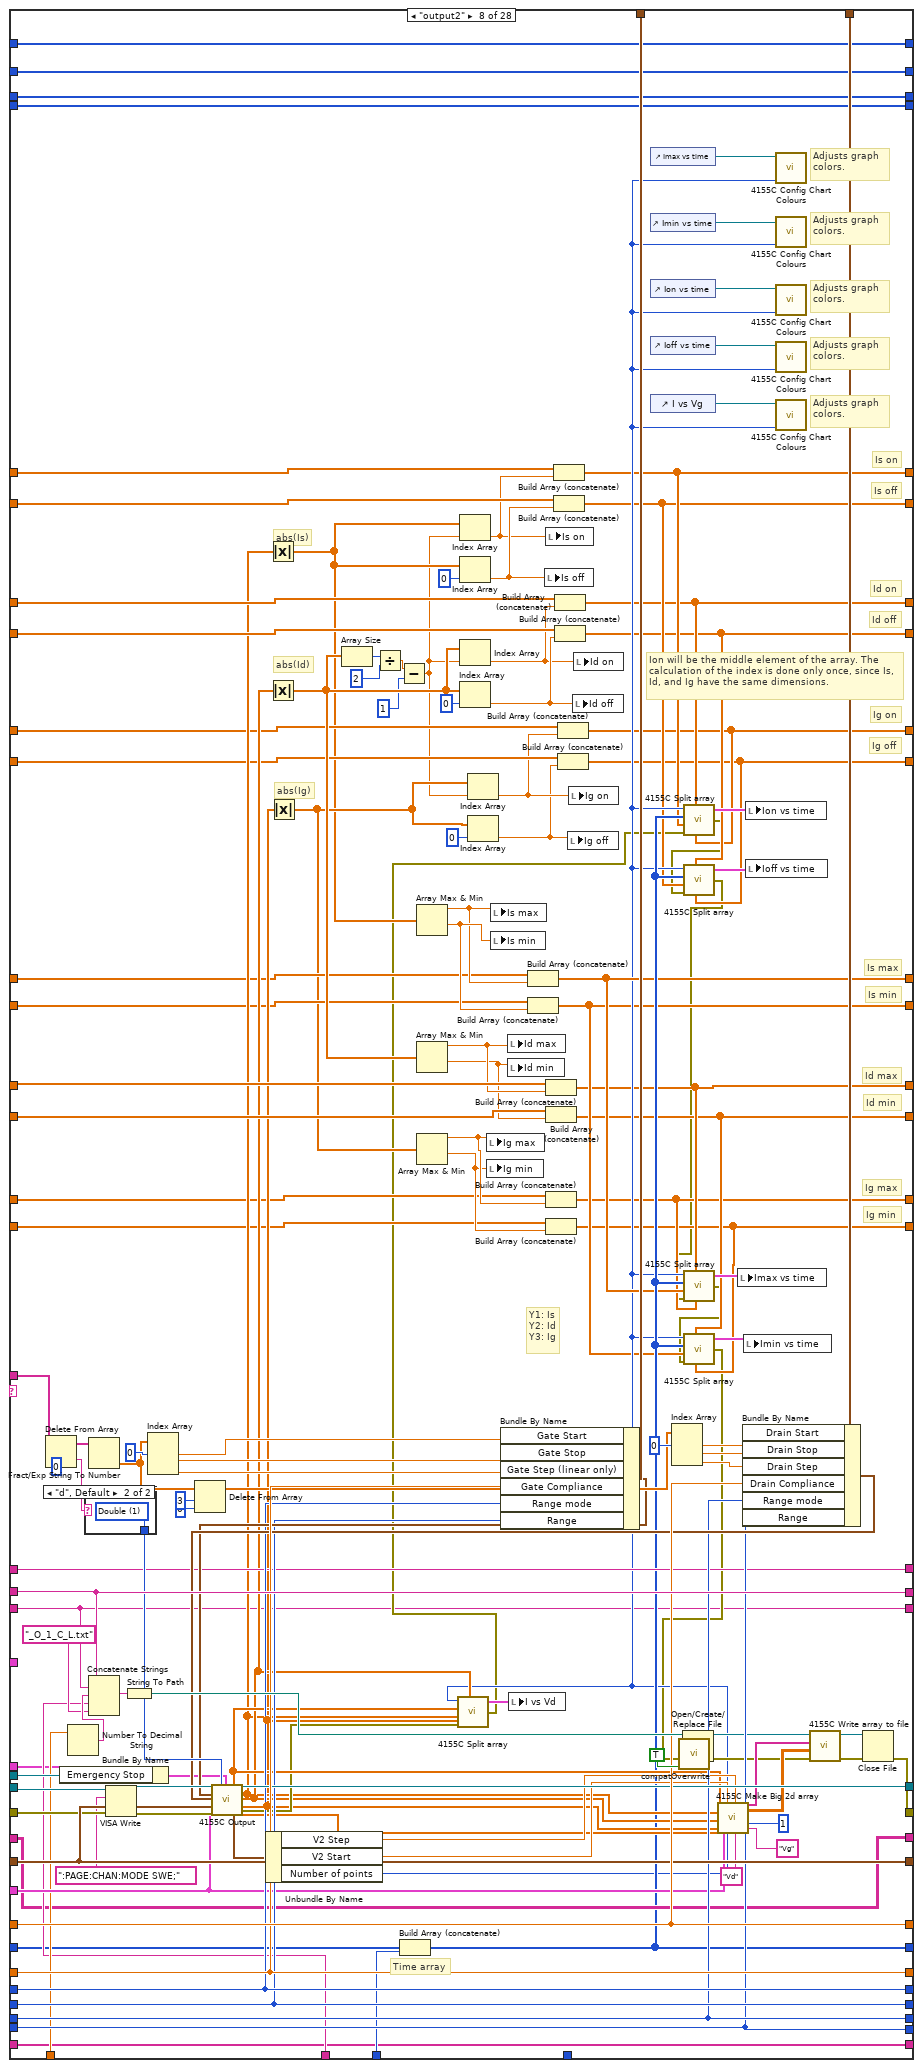
[diagram p18: hidden frame]
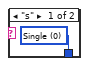
[diagram p19: hidden frame]
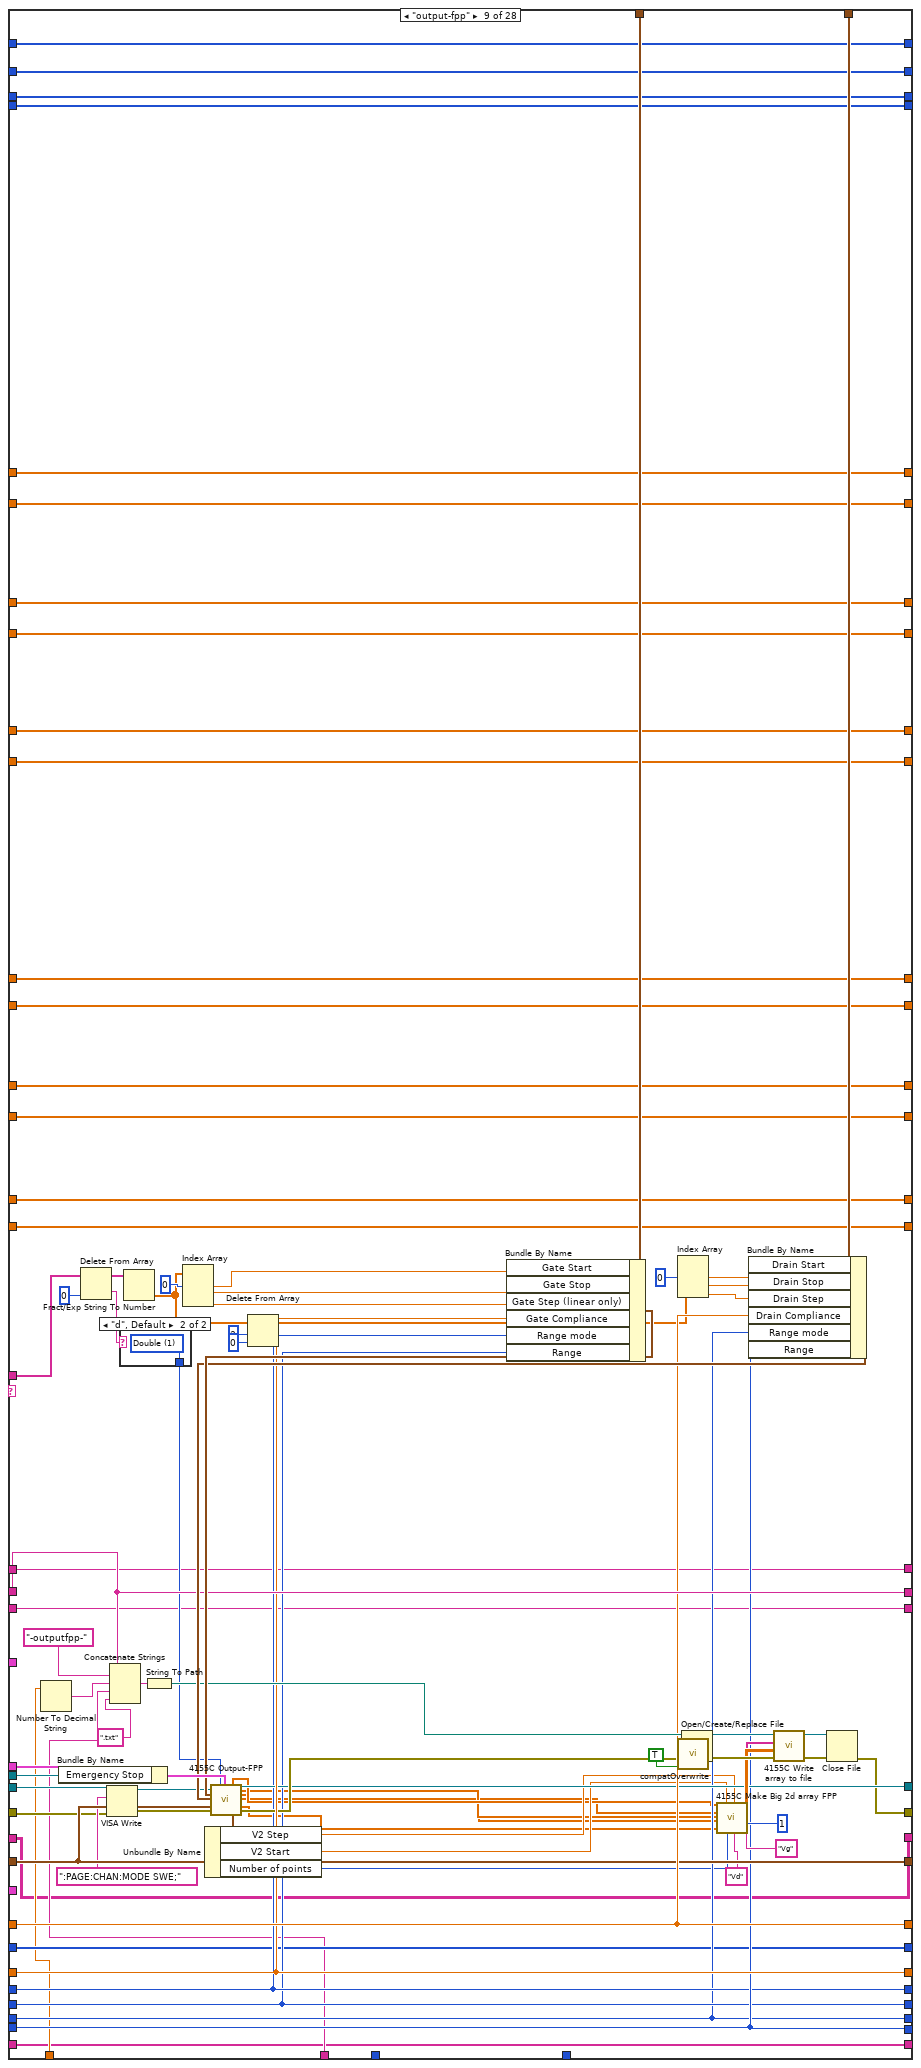
[diagram p20: hidden frame]
diagram:
  w4 = cluster{"Y data in":dbl[], "X data in":dbl[]}[] [] ("I vs Vg")
  w5 = 0.0 ("Is off")
  w6 = 0.0 ("Is on")
  w7 = 0.0 ("Is min")
  w8 = 0.0 ("Is max")
  w59 = u16 1 items=["Reset All", "Partial reset"] ("Type of reset")
  # "Change from previous version:\n\n- Added case structure for time units."
  # "This is a version specific to the SPM pump."
  # "I add 1 to both the \"total lines\" and the \"line running\" indicators because i and N begin from 0, and the script lines begin from 1."
  # "Bugs:\n\n- If using the \"filename\" command, keep in mind that the arrays of the time-dependent data are not re-initialized inbetween filename changes. \n\n- Do not connect the \"error\" wire of a Split block if it has unconnected terminals! It will halt the program."
  # "Array size"
  # "%s option converts a spreadsheet string to an array of strings."
  # "0: No of rows of array\n1: No of cols"
  # "Dimitrios Simatos\nv. 6.1"
  # "Changes from original textcontrol.vi:\n\n- Timestamp appears in filename.\n- (Only) transfer and output curves are plotted.\n- Communication with serial port.\n- Can execute any command, as all pattern matching functions were replaced. Previously, commands with special LabVIEW characters could not be executed.\n- Replaced write to file function with write to text file.\n- Replaced while loop with for loop.\n- Replaced 4155C \"Save File\" function and now the vi can save time-dependent variables.\n- Added clock with start time control and various units.\n- Changed filepath in which the program is saved.\n- Added a serial output log that keeps a history.\n- Tab control.\n- Addition of specialized serial read/write file for the SPM OEM pump.\n- Added halt and hard stop.\n- Imax, Imin, Ion, and Ioff are now saved for all Is, Id, and Ig.\n- Output curves are taken into account in Imax-Imin-Ion-Ioff plots (\"output2\" command).\n- Corrected bug of \"itime\" command. The command did not allow for settting the integration time value, it allowed to set the category of the integration time (short, medium, long). If the time value was beyond the range of the category, then the SPA used the closest value allowed, whilst staying in the category. So, if the integration time was changed to long, but the integration time value was a short one, then the SPA would measure using the minimum long integration time value and not the value that the user intended."
  # "Search and replace LF with EOL"
  n1 = Equal?(x="integration time", y=u32 0) -> (x = y?=w60:bool)
  n2 = Select(t="Integration time (short)", s=w60, f="Integration time (long)") -> (s? t:f=w9:dbl)
  n3 = Bundle By Name(cluster="Timings (overwritten by the Front Panel)", "integration time"="integration time", "Short/Long integration time"=w9) -> (w52:T5)
  n4 = call "4155C Get Filename.vi"("error in (no error)"=errorcluster {"status"=FALSE, "code"=0, "source"=""}) -> ("error out"=w54:errorcluster, "path"=w29:path)  [unwired: 2 in, 1 out]
  "Path" <- w29
  n5 = Path To String(path=w29) -> (string=w30:string)
  n6 = Search and Replace String(replace all?=TRUE ("replace all? (F)"), input string="Script", search string="\n", replace string="\r\n") -> (result string=w42:string)  [unwired: 4 in, 3 out]
  n7 = Match Pattern(string=w30, regular expression=".txt") -> (before substring=w25:string)  [unwired: 1 in, 3 out]
  n8 = Concatenate Strings(w25, "Suffix (script)") -> (w24:string)
  n9 = call "4155C Initialise.vi"("VISA resource name in"=refnum<visa-resource-name> "GPIB0::14::INSTR", "Reset"="Full Reset", "Type of reset"=w59, "error in (no error)"=w54, "VISA Timeout Value"=u32 10000) -> ("VISA Resource Name out"=w53:refnum<visa-resource-name>, "error out"=w22:errorcluster)
  n10 = Spreadsheet String To Array(delimiter (Tab)="\r\n", format string="%s", spreadsheet string="Script", array type (2D Dbl)="") -> (array=w33:string[][])
  n11 = Array Size(array=w33) -> (size(s)=w37:i32[])
  n12 = Initialize Array("") -> (w14:string[])  [unwired: 1 in]
  n13 = String To Path(string=w24) -> (path=w23:path)
  n14 = Initialize Array(0 ("element")) -> (w16:i32[])  [unwired: 1 in]
  n15 = Initialize Array("") -> (w12:string[][])  [unwired: 2 in]
  n16 = Initialize Array(0.0 ("element")) -> (w18:dbl[])  [unwired: 1 in]
  n17 = Index Array(array=w37, index=0) -> (element=w35:i32)
  n18 = Write to Text File(file (use dialog)=w23, text=w42, error in=w22) -> (error out=w21:errorcluster)  [unwired: 1 in, 2 out]
  n19 = for {
    N: w35 -> [w174]
    tunnel: "SMU4" -> [w210]
    shift-left: "Source/Drain Range" -> [w215]
    shift-right: [w211] -> _
    shift-left: "Source/Drain\nRange mode" -> [w216]
    shift-right: [w212] -> _
    shift-left: "Gate Range" -> [w217]
    shift-right: [w213] -> _
    shift-left: "Gate Range\nmode" -> [w218]
    shift-right: [w214] -> _
    shift-left: "Gate: Compliance" -> [w227]
    shift-right: [w223] -> _
    shift-left: "Drain: Compliance" -> [w228]
    shift-right: [w224] -> _
    shift-left: w52 -> [w229]
    shift-right: [w225] -> w10
    shift-left: w21 -> [w230]
    shift-right: [w120] -> w28
    shift-left: w53 -> [w231]
    shift-right: [w226] -> _
    shift-left: w25 -> [w232]
    shift-right: [w124] -> _
    tunnel: "Panel Controls 2" -> [w209]
    shift-right: [w82] -> _
    shift-left: w18 -> [w208]
    shift-right: [w144] -> _
    shift-left: i32[] [] -> [w204]
    tunnel: w33 -> [w203] mode=indexing
    shift-right: [w81] -> _
    shift-left: w18 -> [w180]
    shift-right: [w114] -> _
    shift-left: w14 -> [w166]
    shift-right: [w145] -> _
    shift-left: w16 -> [w161]
    shift-right: [w126] -> _
    shift-left: w16 -> [w160]
    shift-right: [w159] -> _
    shift-left: "" -> [w158]
    shift-right: [w119] -> _
    shift-left: w16 -> [w141]
    shift-right: [w118] -> _
    shift-left: w16 -> [w125]
    shift-right: [w115] -> _
    shift-left: w12 -> [w117]
    shift-right: [w75] -> _
    shift-left: w18 -> [w103]
    shift-right: [w76] -> _
    shift-left: w18 -> [w102]
    shift-right: [w80] -> _
    shift-left: w18 -> [w91]
    shift-right: [w79] -> _
    shift-left: w18 -> [w90]
    shift-right: [w73] -> _
    shift-left: w18 -> [w89]
    shift-right: [w83] -> _
    shift-left: w18 -> [w88]
    shift-right: [w74] -> _
    shift-left: w18 -> [w87]
    shift-right: [w72] -> _
    shift-left: w18 -> [w86]
    shift-right: [w78] -> _
    shift-left: w18 -> [w85]
    shift-right: [w77] -> _
    shift-left: w18 -> [w84]
    shift-right: [w67] -> _
    shift-left: "Filename (variable part)" -> [w66]
    i -> [w169]
    # "Filename prefix"
    # "Is off"
    # "Is on"
    # "Ig off"
    # "Ig on"
    # "Is min"
    # "Is max"
    # "Ig min"
    # "Ig max"
    # "Id min"
    # "Id max"
    # "Id off"
    # "Id on"
    # "Pump status"
    # "Filepath and name"
    # "Pump status"
    # "Limit of command arguments (array columns). Raise if needed."
    # "Serial port data (string)"
    # "Serial port data (table)"
    # "Time array for valve position"
    # "Time array for absolute plunger position"
    # "Valve position"
    # "Absolute plunger position"
    # "Serial port data"
    # "For loop counter"
    # "<-----Equivalent to the 4155C \"Write\" subvi.----->"
    # "Headers"
    # "Save transfer curves in file."
    # "Filepath and name"
    # "Save time-dependent data."
    # "Use the time offset if your measurements do not start at t=0."
    # "Time for Imax, Imin, Ion, Ioff"
    # "Rest of elements of command"
    # "First element of command\n(case select)"
    n20 = Add(x=w169, y=1) -> (x+y=→"Line running":i32)
    n21 = Add(x=w174, y=1) -> (x+y=→"Total lines":i32)
    n22 = Index Array(array=w203, index=0 ("line index")) -> (element=w198:string)
    "Command running:" <- w198
    n23 = control-ref of="Interrupt run"() -> (w222:refnum<vi>)
    n24 = Spreadsheet String To Array(delimiter (Tab)=" ", format string="%s", spreadsheet string=w198, array type (2D Dbl)=string[] []) -> (array=w196:string[])
    n25 = Delete From Array(array=w196, index=0) -> (deleted portion=w104:string, array with subset deleted=w195:string[])  [unwired: 1 in]
    n26 = call "Elapsed Time"("Reset"="Reset", "Auto Reset"="Auto Reset") -> ("Elapsed Time (s)"=w205:dbl)  [unwired: 10 in, 7 out]
    n27 = case shown="0, Default" "Time Units" {
      tunnel: ["_sec" "_min" "_h"] -> w206
      tunnel: [w236 w240 w243] -> w176
      tunnel: w205 -> [w236 w239 w244]
      frame 0, Default {
      }
      frame 1 {
        n28 = Divide(x=w239, y=60.0) -> (x/y=w240:dbl)
      }
      frame 2 {
        n29 = Divide(x=w244, y=3600.0) -> (x/y=w243:dbl)
      }
    }
    n30 = Add(x=w176, y="Time Offset") -> (x+y=w175:dbl)
    n31 = To Long Integer(number=w175) -> (32bit integer=w142:i32)
    "Elapsed Time" <- w142
    n32 = case shown="\"serial\"" w104 {
      tunnel: w195 -> [w281 w319 w356 w488 w512 w658 w752 w904 w982 w1009 w1089 w1135 w1179 w1219 w1252 _ _ w1413 w1493 _ w1596 w1659 w1720 w1809 w1890 w1929 w1999 w2053]
      tunnel: w232 -> [w276 w315 w354 w495 w577 w666 w759 w911 w990 w1032 w1078 w1127 w1172 w1213 w1245 w1283 w1344 w1391 w1475 w1525 w1583 w1646 w1708 w1803 w1886 w1931 w2001 w2055]
      tunnel: w231 -> [w275 w314 w345 w466 w562 w635 w728 w882 w958 w1033 w1079 w1128 w1173 w1214 w1246 w1288 w1346 w1419 w1499 w1529 w1602 w1665 w1726 w1815 w1844 w1935 w2005 w2057]
      tunnel: w230 -> [w274 w313 w344 w465 w561 w634 w725 w881 w955 w1034 w1080 w1129 w1174 w1215 w1247 w1287 w1317 w1418 w1498 w1528 w1601 w1664 w1725 w1814 w1843 w1934 w2004 w2058]
      tunnel: w229 -> [w273 w312 w353 w491 w537 w662 w755 w907 w986 w1042 w1088 w1126 w1171 w1212 w1244 w1286 w1341 w1382 w1467 w1534 w1576 w1639 w1701 w1802 w1885 w1936 w2006 w2060]
      tunnel: w228 -> [w272 w311 w352 w493 w575 w664 w757 w909 w988 w1041 w1087 w1134 w1178 w1218 w1251 w1285 w1326 w1417 w1497 w1537 w1600 w1663 w1724 w1813 w1894 w1937 w2007 w2061]
      tunnel: w227 -> [w271 w310 w351 w492 w574 w663 w756 w908 w987 w1040 w1086 w1133 w1177 w1217 w1250 w1284 w1327 w1392 w1476 w1536 w1584 w1647 w1709 w1804 w1887 w1939 w2008 w2063]
      tunnel: [w275 w314 w343 w490 w572 w660 w754 w906 w984 w1033 w1079 w1128 w1173 w1214 w1246 w1288 w1346 w1383 w1449 w1527 w1577 w1640 w1702 w1755 w1846 w1935 w2005 w2057] -> w226
      tunnel: [w274 w313 w342 w489 w571 w659 w753 w905 w983 w1034 w1080 w1129 w1174 w1215 w1247 w1287 w1316 w1393 w1450 w1526 w1585 w1648 w1710 w1754 w1845 w1933 w2003 w2058] -> w140
      tunnel: [w273 w312 w353 w491 w533 w662 w755 w907 w986 w1035 w1081 w1126 w1171 w1212 w1244 w1286 w1341 w1382 w1467 w1534 w1576 w1639 w1701 w1802 w1885 w1936 w2006 w2060] -> w225
      tunnel: [w272 w311 w352 w493 w575 w664 w757 w909 w988 w1041 w1087 w1134 w1178 w1218 w1251 w1285 w1326 w1417 w1497 w1537 w1600 w1663 w1724 w1813 w1894 w1937 w2007 w2061] -> w224
      tunnel: [w271 w310 w351 w492 w574 w663 w756 w908 w987 w1040 w1086 w1133 w1177 w1217 w1250 w1284 w1327 w1392 w1476 w1536 w1584 w1647 w1709 w1804 w1887 w1939 w2008 w2063] -> w223
      tunnel: [w276 w315 w354 w495 w577 w666 w759 w911 w990 w1032 w1078 w1127 w1172 w1213 w1245 w1283 w1344 w1391 w1475 w1525 w1583 w1646 w1708 w1803 w1886 w1931 w2001 w2055] -> w124
      tunnel: w222 -> [_ _ _ w497 w581 w671 w762 w913 w994 _ _ _ _ _ _ _ _ w1388 w1472 _ w1582 w1645 w1707 w1775 w1862 _ _ _]
      tunnel: "Gate" -> [_ _ _ w475 w565 w645 w739 w891 w969 _ _ _ _ _ _ _ _ _ _ _ _ _ _ _ _ _ _ _]
      tunnel: "Drain 2" -> [_ _ _ w474 w564 w644 w738 w890 w968 _ _ _ _ _ _ _ _ _ _ _ _ _ _ _ _ _ _ _]
      tunnel: "Panel Controls" -> [_ _ _ _ _ w643 w737 w775 w967 _ _ _ _ _ _ _ _ _ _ _ _ _ _ _ _ _ _ _]
      tunnel: w218 -> [w270 w309 w350 w459 w555 w628 w723 w875 w953 w1039 w1085 _ w1170 w1211 w1243 w1282 w1328 w1378 w1463 w1530 w1572 w1635 w1697 w1798 w1881 w1940 w2009 w2064]
      tunnel: w217 -> [w269 w308 w349 w458 w554 w627 w722 w874 w952 w1038 w1084 w1132 _ w1202 w1249 w1281 w1329 w1379 w1464 w1531 w1573 w1636 w1698 w1799 w1882 w1941 w2010 w2065]
      tunnel: w216 -> [w268 w307 w348 w457 w553 w626 w721 w873 w951 w1037 w1083 w1131 w1176 w1216 _ w1280 w1330 w1380 w1465 w1532 w1574 w1637 w1699 w1800 w1883 w1942 w2011 w2066]
      tunnel: w215 -> [w267 w306 w347 w456 w552 w625 w724 w872 w954 w1036 w1082 w1130 w1175 _ w1248 w1279 w1331 w1381 w1466 w1533 w1575 w1638 w1700 w1801 w1884 w1943 w2012 w2067]
      tunnel: [w270 w309 w350 w459 w555 w628 w723 w875 w953 w1039 w1085 w1125 w1170 w1211 w1243 w1282 w1328 w1378 w1463 w1530 w1572 w1635 w1697 w1798 w1881 w1940 w2009 w2064] -> w214
      tunnel: [w269 w308 w349 w458 w554 w627 w722 w874 w952 w1038 w1084 w1132 w1162 w1202 w1249 w1281 w1329 w1379 w1464 w1531 w1573 w1636 w1698 w1799 w1882 w1941 w2010 w2065] -> w213
      tunnel: [w268 w307 w348 w457 w553 w626 w721 w873 w951 w1037 w1083 w1131 w1176 w1216 w1242 w1280 w1330 w1380 w1465 w1532 w1574 w1637 w1699 w1800 w1883 w1942 w2011 w2066] -> w212
      tunnel: [w267 w306 w347 w456 w552 w625 w724 w872 w954 w1036 w1082 w1130 w1175 w1203 w1248 w1279 w1331 w1381 w1466 w1533 w1575 w1638 w1700 w1801 w1884 w1943 w2012 w2067] -> w211
      tunnel: w210 -> [_ _ _ w451 w549 _ w717 w867 _ _ _ _ _ _ _ _ _ _ _ _ _ _ _ _ _ _ _ _]
      tunnel: w209 -> [_ _ _ w449 w548 _ _ _ _ _ _ _ _ _ _ _ _ _ _ _ _ _ _ _ _ _ _ _]
      tunnel: [w266 w302 w340 w377 w525 w615 w714 w794 w940 w1031 w1076 w1124 w1161 w1201 w1241 w1278 w1312 w1370 w1428 w1524 w1561 w1628 w1691 w1752 w1839 w1932 w2002 w2072] -> w82
      tunnel: w208 -> [w266 w302 w340 w446 w525 w615 w714 w863 w940 w1031 w1076 w1124 w1161 w1201 w1241 w1278 w1312 w1370 w1428 w1524 w1561 w1628 w1691 w1752 w1839 w1932 w2002 w2072]
      tunnel: w175 -> [_ _ _ w443 w522 w613 w711 w860 w937 _ _ _ _ _ _ _ w1310 w1368 w1445 _ w1558 w1625 w1688 w1749 w1835 _ _ _]
      tunnel: w206 -> [_ _ _ w440 w521 w611 w710 w857 w936 _ _ _ _ _ _ _ w1308 w1366 w1444 _ w1557 w1624 w1687 w1748 w1836 _ w1970 _]
      tunnel: w142 -> [_ _ _ w435 _ _ _ w852 _ _ _ _ _ _ _ _ _ _ _ _ _ _ _ _ _ _ w1973 _]
      tunnel: [w265 w301 w339 w385 w524 w614 w713 w802 w939 w1030 w1075 w1123 w1160 w1200 w1240 w1277 w1311 w1369 w1447 w1523 w1560 w1627 w1690 w1751 w1838 w1938 w1982 w2062] -> w144
      tunnel: w204 -> [w265 w301 w339 w439 w524 w614 w713 w856 w939 w1030 w1075 w1123 w1160 w1200 w1240 w1277 w1311 w1369 w1447 w1523 w1560 w1627 w1690 w1751 w1838 w1938 w1982 w2062]
      tunnel: [w264 w300 w338 w376 w520 w610 w709 w793 w935 w1029 w1074 w1122 w1159 w1199 w1239 w1276 w1307 w1365 w1427 w1522 w1556 w1623 w1686 w1747 w1834 w1927 w1998 w2071] -> w81
      tunnel: w180 -> [w264 w300 w338 w433 w520 w610 w709 w850 w935 w1029 w1074 w1122 w1159 w1199 w1239 w1276 w1307 w1365 w1427 w1522 w1556 w1623 w1686 w1747 w1834 w1927 w1998 w2071]
      tunnel: [w263 w299 w337 w426 w519 w609 w699 w843 w934 w1028 w1073 w1121 w1158 w1198 w1238 w1275 w1306 w1364 w1443 w1521 w1555 w1622 w1685 w1746 w1833 w1926 w1997 w2068] -> w114
      tunnel: w166 -> [w263 w299 w337 w426 w519 w609 w699 w843 w934 w1028 w1073 w1121 w1158 w1198 w1238 w1275 w1306 w1364 w1443 w1521 w1555 w1622 w1685 w1746 w1833 w1925 w1971 w2068]
      tunnel: [w262 w298 w336 w425 w518 w608 w698 w842 w933 w1027 w1072 w1120 w1157 w1197 w1237 w1274 w1305 w1363 w1442 w1520 w1554 w1621 w1684 w1745 w1832 w1911 w1984 w2082] -> w145
      tunnel: w161 -> [w262 w298 w336 w425 w518 w608 w698 w842 w933 w1027 w1072 w1120 w1157 w1197 w1237 w1274 w1305 w1363 w1442 w1520 w1554 w1621 w1684 w1745 w1832 w1911 w1983 w2082]
      tunnel: [w261 w297 w335 w424 w517 w607 w697 w841 w932 w1026 w1071 w1119 w1156 w1196 w1236 w1273 w1304 w1362 w1441 w1519 w1553 w1620 w1683 w1744 w1831 w1910 w1966 w2084] -> w126
      tunnel: w160 -> [w261 w297 w335 w424 w517 w607 w697 w841 w932 w1026 w1071 w1119 w1156 w1196 w1236 w1273 w1304 w1362 w1441 w1519 w1553 w1620 w1683 w1744 w1831 w1910 w1964 w2084]
      tunnel: [w260 w296 w334 w423 w516 w606 w696 w840 w931 w1025 w1070 w1118 w1155 w1195 w1235 w1272 w1303 w1361 w1440 w1518 w1552 w1619 w1682 w1743 w1830 w1909 w1963 w2056] -> w159
      tunnel: w158 -> [w260 w296 w334 w423 w516 w606 w696 w840 w931 w1025 w1070 w1118 w1155 w1195 w1235 w1272 w1303 w1361 w1440 w1518 w1552 w1619 w1682 w1743 w1830 w1909 w1974 w2056]
      tunnel: w142 -> [_ _ _ _ _ _ _ _ _ _ _ _ _ _ _ _ _ _ _ _ _ _ _ _ _ _ w1962 _]
      tunnel: w141 -> [w259 w295 w333 w422 w515 w605 w695 w839 w930 w1024 w1069 w1117 w1154 w1194 w1234 w1271 w1302 w1360 w1439 w1517 w1551 w1618 w1681 w1742 w1829 w1908 w1961 w2083]
      tunnel: [w259 w295 w333 w422 w515 w605 w695 w839 w930 w1024 w1069 w1117 w1154 w1194 w1234 w1271 w1302 w1360 w1439 w1517 w1551 w1618 w1681 w1742 w1829 w1908 w1960 w2083] -> w119
      tunnel: [w258 w294 w332 w421 w514 w604 w694 w838 w929 w1023 w1068 w1116 w1153 w1193 w1233 w1270 w1301 w1359 w1438 w1516 w1550 w1617 w1680 w1741 w1828 w1907 w1959 w2081] -> w118
      tunnel: w125 -> [w258 w294 w332 w421 w514 w604 w694 w838 w929 w1023 w1068 w1116 w1153 w1193 w1233 w1270 w1301 w1359 w1438 w1516 w1550 w1617 w1680 w1741 w1828 w1907 w1958 w2081]
      tunnel: [w257 w293 w331 w420 w513 w603 w693 w837 w928 w1022 w1067 w1115 w1152 w1192 w1232 w1269 w1300 w1358 w1437 w1515 w1549 w1616 w1679 w1740 w1827 w1906 w1956 w2059] -> w115
      tunnel: w117 -> [w257 w293 w331 w420 w513 w603 w693 w837 w928 w1022 w1067 w1115 w1152 w1192 w1232 w1269 w1300 w1358 w1437 w1515 w1549 w1616 w1679 w1740 w1827 w1906 w1955 w2059]
      tunnel: [w255 w291 w329 w370 w510 w601 w691 w787 w926 w1020 w1066 w1114 w1150 w1190 w1230 w1267 w1298 w1357 w1436 w1514 w1548 w1615 w1677 w1739 w1826 w1905 w1954 w2077] -> w75
      tunnel: w103 -> [w255 w291 w329 w416 w510 w601 w691 w833 w926 w1020 w1066 w1114 w1150 w1190 w1230 w1267 w1298 w1357 w1436 w1514 w1548 w1615 w1677 w1739 w1826 w1905 w1954 w2077]
      tunnel: [w256 w292 w330 w371 w511 w602 w692 w788 w927 w1021 w1065 w1113 w1151 w1191 w1231 w1268 w1299 w1356 w1435 w1513 w1547 w1614 w1678 w1738 w1825 w1904 w1953 w2078] -> w76
      tunnel: w102 -> [w256 w292 w330 w415 w511 w602 w692 w832 w927 w1021 w1065 w1113 w1151 w1191 w1231 w1268 w1299 w1356 w1435 w1513 w1547 w1614 w1678 w1738 w1825 w1904 w1953 w2078]
      tunnel: [w248 w284 w322 w375 w507 w599 w689 w792 w924 w1013 w1063 w1111 w1148 w1188 w1228 w1265 w1291 w1349 w1426 w1512 w1540 w1607 w1670 w1731 w1820 w1897 w1952 w2070] -> w80
      tunnel: w91 -> [w248 w284 w322 w405 w507 w599 w689 w822 w924 w1013 w1063 w1111 w1148 w1188 w1228 w1265 w1291 w1349 w1426 w1512 w1540 w1607 w1670 w1731 w1820 w1897 w1952 w2070]
      tunnel: [w247 w283 w321 w374 w508 w600 w690 w791 w925 w1012 w1064 w1112 w1149 w1189 w1229 w1266 w1290 w1348 w1425 w1511 w1539 w1606 w1669 w1730 w1819 w1896 w1951 w2069] -> w79
      tunnel: w90 -> [w247 w283 w321 w404 w508 w600 w690 w821 w925 w1012 w1064 w1112 w1149 w1189 w1229 w1266 w1290 w1348 w1425 w1511 w1539 w1606 w1669 w1730 w1819 w1896 w1951 w2069]
      tunnel: [w250 w286 w324 w380 w506 w597 w687 w797 w922 w1018 w1061 w1109 w1146 w1186 w1226 w1263 w1293 w1351 w1430 w1506 w1542 w1609 w1672 w1733 w1818 w1901 w1949 w2074] -> w73
      tunnel: w89 -> [w250 w286 w324 w401 w506 w597 w687 w818 w922 w1018 w1061 w1109 w1146 w1186 w1226 w1263 w1293 w1351 w1430 w1506 w1542 w1609 w1672 w1733 w1818 w1901 w1949 w2074]
      tunnel: [w249 w285 w323 w378 w509 w598 w688 w795 w923 w1019 w1062 w1110 w1147 w1187 w1227 w1264 w1292 w1350 w1429 w1505 w1541 w1608 w1671 w1732 w1817 w1900 w1950 w2073] -> w83
      tunnel: w88 -> [w249 w285 w323 w400 w509 w598 w688 w817 w923 w1019 w1062 w1110 w1147 w1187 w1227 w1264 w1292 w1350 w1429 w1505 w1541 w1608 w1671 w1732 w1817 w1900 w1950 w2073]
      tunnel: [w252 w288 w326 w369 w505 w595 w685 w786 w920 w1016 w1059 w1107 w1144 w1184 w1224 w1261 w1295 w1353 w1432 w1508 w1544 w1611 w1674 w1735 w1822 w1903 w1947 w2076] -> w74
      tunnel: w87 -> [w252 w288 w326 w397 w505 w595 w685 w814 w920 w1016 w1059 w1107 w1144 w1184 w1224 w1261 w1295 w1353 w1432 w1508 w1544 w1611 w1674 w1735 w1822 w1903 w1947 w2076]
      tunnel: [w251 w287 w325 w368 w504 w596 w686 w785 w921 w1017 w1060 w1108 w1145 w1185 w1225 w1262 w1294 w1352 w1431 w1507 w1543 w1610 w1673 w1734 w1821 w1902 w1948 w2075] -> w72
      tunnel: w86 -> [w251 w287 w325 w396 w504 w596 w686 w813 w921 w1017 w1060 w1108 w1145 w1185 w1225 w1262 w1294 w1352 w1431 w1507 w1543 w1610 w1673 w1734 w1821 w1902 w1948 w2075]
      tunnel: [w254 w290 w328 w373 w503 w593 w683 w790 w918 w1014 w1057 w1105 w1142 w1182 w1222 w1259 w1297 w1355 w1434 w1510 w1546 w1613 w1676 w1737 w1824 w1899 w1945 w2080] -> w78
      tunnel: w85 -> [w254 w290 w328 w393 w503 w593 w683 w810 w918 w1014 w1057 w1105 w1142 w1182 w1222 w1259 w1297 w1355 w1434 w1510 w1546 w1613 w1676 w1737 w1824 w1899 w1945 w2080]
      tunnel: [w253 w289 w327 w372 w502 w594 w684 w789 w919 w1015 w1058 w1106 w1143 w1183 w1223 w1260 w1296 w1354 w1433 w1509 w1545 w1612 w1675 w1736 w1823 w1898 w1946 w2079] -> w77
      tunnel: w84 -> [w253 w289 w327 w392 w502 w594 w684 w809 w919 w1015 w1058 w1106 w1143 w1183 w1223 w1260 w1296 w1354 w1433 w1509 w1545 w1612 w1675 w1736 w1823 w1898 w1946 w2079]
      tunnel: w66 -> [w246 w282 w320 w359 w501 w592 w682 w776 w917 w1011 w1056 w1104 w1141 w1181 w1221 w1258 w1289 w1347 w1424 w1504 w1538 w1605 w1668 w1729 w1816 w1895 w1944 _]
      tunnel: [w246 w282 w320 w359 w501 w592 w682 w776 w917 w1011 w1056 w1104 w1141 w1181 w1221 w1258 w1289 w1347 w1424 w1504 w1538 w1605 w1668 w1729 w1816 w1895 w1944 w2052] -> w67
      frame "wait" {
        n33 = Index Array(array=w281, index=0 ("Index")) -> (element=w279:string)
        n34 = Decimal String To Number(string=w279, default (0L)=u32 0) -> (number=w278:u32)  [unwired: 1 in, 1 out]
        n35 = Wait (ms)(milliseconds to wait=w278) -> ()  [unwired: 1 out]
      }
      frame "wait-min" {
        n36 = Index Array(array=w319, index=0 ("Index")) -> (element=w317:string)
        n37 = Decimal String To Number(string=w317, default (0L)=u32 0) -> (number=w305:u32)  [unwired: 1 in, 1 out]
        n38 = Multiply(x=w305, y=u32 60000) -> (x*y=w304:u32)
        n39 = Wait (ms)(milliseconds to wait=w304) -> ()  [unwired: 1 out]
      }
      frame "standby" {
        n40 = Index Array(array=w356, index=0 ("Index")) -> (element=w346:string)
        n41 = case shown="\"off\", Default" w346 {
          tunnel: [":PAGE:SCON:STAN 0" ":PAGE:SCON:STAN 1"] -> w341
          frame "off", Default {
          }
          frame "on" {
          }
        }
        n42 = VISA Write(VISA resource name=w345, write buffer=w341, error in (no error)=w344) -> (VISA resource name out=w343:refnum<visa-resource-name>, error out=w342:errorcluster)  [unwired: 1 out]
      }
      frame "transfer" {
        # "Adjusts graph colors."
        # "Adjusts graph colors."
        # "Is off"
        # "Is on"
        # "Ion will be the middle element of the array. The calculation of the index is done only once, since Is, Id, and Ig have the same dimensions."
        # "Ig off"
        # "Ig on"
        # "Is min"
        # "Is max"
        # "Ig min"
        # "Ig max"
        # "abs(Ig)"
        # "abs(Is)"
        # "Id min"
        # "Id max"
        # "Y1: Is\nY2: Id\nY3: Ig"
        # "abs(Id)"
        # "Adjusts graph colors."
        # "Adjusts graph colors."
        # "Id off"
        # "Id on"
        # "Adjusts graph colors."
        # "Time array"
        n43 = Delete From Array(array=w488, index=0 ("Index")) -> (deleted portion=w486:string, array with subset deleted=w485:string[])  [unwired: 1 in]
        n44 = Bundle By Name(cluster=w449, "Emergency Stop"=w497) -> (w450:T2)
        n45 = Number To Decimal String(number=w443) -> (decimal integer string=w442:string)  [unwired: 1 in]
        n46 = case shown="\"d\", Default" w486 {
          tunnel: [w499 w500] -> w484
          frame "s" {
            w499 = u16 0 items=["Single", "Double"] ("sweep mode")
          }
          frame "d", Default {
            w500 = u16 1 items=["Single", "Double"] ("sweep mode")
          }
        }
        n47 = Fract/Exp String To Number(string=w485) -> (number=w470:dbl[])  [unwired: 3 in, 1 out]
        n48 = Concatenate Strings(w495, w359, w442, w440, "_T_1_C_L.txt" ("Suffix (transfer)")) -> (w496:string)
        n49 = VISA Write(VISA resource name=w466, write buffer=":PAGE:CHAN:MODE SWE;" ("write buffer (\"\")"), error in (no error)=w465) -> (VISA resource name out=w463:refnum<visa-resource-name>, error out=w464:errorcluster)  [unwired: 1 out]
        n50 = String To Path(string=w496) -> (path=w494:path)
        n51 = Index Array(array=w470, index #1=0 ("Index")) -> (element #1=w483:dbl, element #2=w482:dbl, element #3=w481:dbl)  [unwired: 2 in]
        n52 = Delete From Array(array=w470, length=3 ("Length"), index=0 ("Index")) -> (array with subset deleted=w468:dbl[])  [unwired: 1 out]
        n53 = Build Array (concatenate)(w439, w435) -> (w385:i32[])
        n54 = Bundle By Name(cluster=w475, "Gate Start"=w483, "Gate Stop"=w482, "Gate Step (linear only)"=w481, "Gate Compliance"=w492, "Range mode"=w459, "Range"=w458) -> (w460:T6)
        n55 = control-ref of="Imax vs time"() -> (w414:refnum<vi>)
        n56 = control-ref of="Imin vs time"() -> (w413:refnum<vi>)
        n57 = control-ref of="Ion vs time"() -> (w382:refnum<vi>)
        n58 = control-ref of="Ioff vs time"() -> (w381:refnum<vi>)
        n59 = control-ref of="I vs Vg"() -> (w444:refnum<vi>)
        n60 = Index Array(array=w468, index #1=0 ("Index")) -> (element #1=w478:dbl, element #2=w477:dbl, element #3=w476:dbl)  [unwired: 2 in]
        n61 = call <vilib>:"compatOverwrite.vi"("overwrite (F)"=TRUE) -> ("overwrite?"=w448:T8)
        n62 = Bundle By Name(cluster=w474, "Drain Start"=w478, "Drain Stop"=w477, "Drain Step"=w476, "Drain Compliance"=w493, "Range mode"=w457, "Range"=w456) -> (w461:T7)
        n63 = call "4155C Transfer.vi"("VISA resource name in"=w463, "Gate"=w460, "Drain"=w461, "Timings"=w491, "error in (no error)"=w464, "SMU4"=w451, "sweep mode"=w484, "Panel Controls"=w450) -> ("VG"=w447:dbl[], "Outparams"=w455:T9, "VISA Resource Name out"=w490:refnum<visa-resource-name>, "IS"=w410:dbl[], "ID"=w412:dbl[], "IG"=w409:dbl[], "error out"=w436:errorcluster, "SMU4"=w452:dbl[])  [unwired: 12 in]
        n64 = Unbundle By Name(w455) -> ("V2 Step"=w454:dbl, "V2 Start"=w453:dbl, "Number of points"=w379:i32)
        n65 = Absolute Value(x=w410) -> (abs(x)=w395:dbl[])
        n66 = Absolute Value(x=w412) -> (abs(x)=w411:dbl[])
        n67 = Absolute Value(x=w409) -> (abs(x)=w398:dbl[])
        n68 = Array Size(array=w411) -> (size(s)=w419:i32)
        n69 = Divide(x=w419, y=2) -> (x/y=w362:dbl)
        n70 = Subtract(x=w362, y=1) -> (x-y=w361:dbl)
        n71 = Array Max & Min(array=w395) -> (max value=w402:dbl, min value=w403:dbl)  [unwired: 2 out]
        n72 = Array Max & Min(array=w411) -> (max value=w445:dbl, min value=w408:dbl)  [unwired: 2 out]
        n73 = Array Max & Min(array=w398) -> (max value=w407:dbl, min value=w406:dbl)  [unwired: 2 out]
        n74 = call "4155C Split array.vi"("Number of VAR2 steps"=w379, "Y2 data in"=w412, "X data in"=w447, "Y1 data in"=w410, "Y3 data in"=w409, "error in (no error)"=w436) -> ("Array of clusters"=w438:cluster{"Y data in":dbl[], "X data in":dbl[]}[], "error out"=w367:errorcluster)  [unwired: 1 in]
        n75 = Index Array(array=w395, index=w361) -> (element=w386:dbl)
        n76 = Index Array(array=w395, index=0) -> (element=w387:dbl)
        n77 = Index Array(array=w411, index=w361) -> (element=w388:dbl)
        n78 = Index Array(array=w411, index=0) -> (element=w389:dbl)
        n79 = Index Array(array=w398, index=w361) -> (element=w391:dbl)
        n80 = Index Array(array=w398, index=0) -> (element=w390:dbl)
        n81 = local write "Ig max"(w407) -> ()
        n82 = local write "Ig min"(w406) -> ()
        n83 = local write "Is max"(w402) -> ()
        n84 = local write "Is min"(w403) -> ()
        n85 = local write "Id max"(w445) -> ()
        n86 = local write "Id min"(w408) -> ()
        n87 = local write "I vs Vg"(w438) -> ()
        n88 = Build Array (concatenate)(w401, w402) -> (w380:dbl[])
        n89 = Build Array (concatenate)(w400, w403) -> (w378:dbl[])
        n90 = local write "Is off"(w387) -> ()
        n91 = local write "Is on"(w386) -> ()
        n92 = Build Array (concatenate)(w446, w445) -> (w377:dbl[])
        n93 = Build Array (concatenate)(w433, w408) -> (w376:dbl[])
        n94 = Build Array (concatenate)(w405, w407) -> (w375:dbl[])
        n95 = Build Array (concatenate)(w404, w406) -> (w374:dbl[])
        n96 = Build Array (concatenate)(w393, w386) -> (w373:dbl[])
        n97 = Build Array (concatenate)(w392, w387) -> (w372:dbl[])
        n98 = Build Array (concatenate)(w415, w388) -> (w371:dbl[])
        n99 = Build Array (concatenate)(w416, w389) -> (w370:dbl[])
        n100 = Build Array (concatenate)(w397, w391) -> (w369:dbl[])
        n101 = Build Array (concatenate)(w396, w390) -> (w368:dbl[])
        n102 = local write "Ig off"(w390) -> ()
        n103 = local write "Ig on"(w391) -> ()
        n104 = local write "Id off"(w389) -> ()
        n105 = local write "Id on"(w388) -> ()
        n106 = call "4155C Split array.vi"("Number of VAR2 steps"=w379, "Y2 data in"=w371, "X data in"=w385, "Y1 data in"=w373, "Y3 data in"=w369, "error in (no error)"=w367) -> ("Array of clusters"=w383:cluster{"Y data in":dbl[], "X data in":dbl[]}[], "error out"=w366:errorcluster)  [unwired: 1 in]
        n107 = call "4155C Split array.vi"("Number of VAR2 steps"=w379, "Y2 data in"=w370, "X data in"=w385, "Y1 data in"=w372, "Y3 data in"=w368, "error in (no error)"=w366) -> ("Array of clusters"=w384:cluster{"Y data in":dbl[], "X data in":dbl[]}[], "error out"=w365:errorcluster)  [unwired: 1 in]
        n108 = call "4155C Split array.vi"("Number of VAR2 steps"=w379, "Y2 data in"=w377, "X data in"=w385, "Y1 data in"=w380, "Y3 data in"=w375, "error in (no error)"=w365) -> ("Array of clusters"=w437:cluster{"Y data in":dbl[], "X data in":dbl[]}[], "error out"=w364:errorcluster)  [unwired: 1 in]
        n109 = call "4155C Split array.vi"("Number of VAR2 steps"=w379, "Y2 data in"=w376, "X data in"=w385, "Y1 data in"=w378, "Y3 data in"=w374, "error in (no error)"=w364) -> ("Array of clusters"=w434:cluster{"Y data in":dbl[], "X data in":dbl[]}[], "error out"=w363:errorcluster)  [unwired: 1 in]
        n110 = Open/Create/Replace File(file path (use dialog)=w494, error in=w363, operation (0:open)=w448) -> (refnum out=w431:refnum<file>, error out=w429:errorcluster)  [unwired: 3 in, 1 out]
        n111 = call "4155C Make Big 2d array.vi"("1D Var1"=w447, "1d IS"=w410, "1d ID"=w412, "1d IG"=w409, "1d SMU4"=w452, "SMU4"=w451, "VAR2 START"=w453, "Number of VAR2 steps"=w379, "VAR2 STEP"=w454, "VAR1 Name"="Vg", "Decimal places in header"=i8 1, "VAR2 Name"="Vd") -> ("Header array"=w432:string[], "Data array"=w430:dbl[][])  [unwired: 14 in]
        n112 = local write "Imax vs time"(w437) -> ()
        n113 = local write "Imin vs time"(w434) -> ()
        n114 = local write "Ion vs time"(w383) -> ()
        n115 = local write "Ioff vs time"(w384) -> ()
        n116 = call "4155C Config Chart Colours.vi"("Numeric"=w379, "XY Graph 2"=w414) -> ()  [unwired: 6 in]
        n117 = call "4155C Config Chart Colours.vi"("Numeric"=w379, "XY Graph 2"=w413) -> ()  [unwired: 6 in]
        n118 = call "4155C Config Chart Colours.vi"("Numeric"=w379, "XY Graph 2"=w382) -> ()  [unwired: 6 in]
        n119 = call "4155C Config Chart Colours.vi"("Numeric"=w379, "XY Graph 2"=w381) -> ()  [unwired: 6 in]
        n120 = call "4155C Config Chart Colours.vi"("Numeric"=w379, "XY Graph 2"=w444) -> ()  [unwired: 6 in]
        n121 = call "4155C Write array to file.vi"("Byte Stream File Refnum"=w431, "Header"=w432, "Data Array"=w430, "error in (no error)"=w429) -> ("dup refnum"=w428:refnum<file>, "error out"=w427:errorcluster)  [unwired: 1 in]
        n122 = Close File(refnum=w428, error in=w427) -> (error out=w489:errorcluster)  [unwired: 1 out]
      }
      frame "pulsedstressV" {
        w531 = 0
        n123 = Number To Decimal String(number=w522) -> (decimal integer string=w578:string)  [unwired: 1 in]
        n124 = Delete From Array(array=w512, index=0 ("Index")) -> (deleted portion=w569:string, array with subset deleted=w568:string[])  [unwired: 1 in]
        n125 = Bundle By Name(cluster=w548, "Emergency Stop"=w581) -> (w550:T2)
        n126 = VISA Write(VISA resource name=w562, write buffer=":PAGE:CHAN:MODE SWE;" ("write buffer (\"\")"), error in (no error)=w561) -> (VISA resource name out=w559:refnum<visa-resource-name>, error out=w560:errorcluster)  [unwired: 1 out]
        n127 = Concatenate Strings(w577, "-pulsedstressV-" ("Substring"), w578, w521, ".txt" ("Substring")) -> (w580:string)
        n128 = case shown="\"d\", Default" w569 {
          tunnel: [w590 w591] -> w567
          frame "s" {
            w590 = u16 0 items=["Single", "Double"] ("sweep mode")
          }
          frame "d", Default {
            w591 = u16 1 items=["Single", "Double"] ("sweep mode")
          }
        }
        n129 = Fract/Exp String To Number(string=w568) -> (number=w563:dbl[])  [unwired: 3 in, 1 out]
        n130 = String To Path(string=w580) -> (path=w576:path)
        n131 = Index Array(array=w563, index #1=0 ("Index")) -> (element #1=w540:dbl, element #2=w539:dbl, element #3=w536:dbl, element #4=w535:dbl, element #5=w534:dbl, element #6=w538:dbl)  [unwired: 5 in]
        n132 = Bundle By Name(cluster=w537, "Pulse period"=w535, "Base voltage"=w536, "Pulse width"=w534) -> (w533:T5)
        n133 = Unbundle By Name(w533) -> ("Pulse period"=w541:dbl)
        n134 = Bundle By Name(cluster=w565, "Gate Start"=w539, "Gate Stop"=w540, "Gate Step (linear only)"=0, "Gate Compliance"=w574, "Range mode"=w555, "Range"=w554) -> (w556:T6)
        n135 = call <vilib>:"compatOverwrite.vi"("overwrite (F)"=TRUE) -> ("overwrite?"=w526:T8)
        n136 = Bundle By Name(cluster=w564, "Drain Start"=w538, "Drain Stop"=w531, "Drain Step"=w531, "Drain Compliance"=w575, "Range mode"=w553, "Range"=w552) -> (w557:T7)
        n137 = call "4155C PulsedStressV.vi"("VISA resource name in"=w559, "sweep mode"=w567, "Panel Controls"=w550, "Gate"=w556, "Drain"=w557, "Timings"=w533, "error in (no error)"=w560, "SMU4"=w549) -> ("VISA Resource Name out"=w572:refnum<visa-resource-name>, "ID"=w529:dbl[], "IG"=w527:dbl[], "Outparams"=w551:T9, "error out"=w573:errorcluster)  [unwired: 3 in]
        n138 = Unbundle By Name(w551) -> ("Number of points"=w528:i32)  [unwired: 2 out]
        n139 = for {
          N: w528 -> [_]
          tunnel: [w587] -> w530 mode=indexing
          tunnel: w541 -> [w589]
          i -> [w588]
          n140 = Multiply(x=w589, y=w588) -> (x*y=w587:dbl)
        }
        n141 = Insert Into Array(array=dbl[][] [] ("Input Array"), new element=w530) -> (w542:dbl[][])  [unwired: 2 in]
        n142 = Insert Into Array(array=w542, new element=w529) -> (w547:dbl[][])  [unwired: 2 in]
        n143 = Insert Into Array(array=w547, new element=w527) -> (w546:dbl[][])  [unwired: 2 in]
        n144 = Transpose 2D Array(2D array=w546) -> (transposed array=w545:dbl[][])
        n145 = Open/Create/Replace File(file path (use dialog)=w576, error in=w573, operation (0:open)=w526) -> (refnum out=w584:refnum<file>, error out=w585:errorcluster)  [unwired: 3 in, 1 out]
        n146 = call "4155C Write array to file.vi"("Byte Stream File Refnum"=w584, "Header"=string[] ["Time /s", "Id /A", "Ig /A"], "Data Array"=w545, "error in (no error)"=w585) -> ("dup refnum"=w582:refnum<file>, "error out"=w583:errorcluster)  [unwired: 1 in]
        n147 = Close File(refnum=w582, error in=w583) -> (error out=w571:errorcluster)  [unwired: 1 out]
      }
      frame "transfer-fpp" {
        n148 = Number To Decimal String(number=w613) -> (decimal integer string=w667:string)  [unwired: 1 in]
        n149 = Bundle By Name(cluster=w643, "Emergency Stop"=w671) -> (w679:T1)
        n150 = Delete From Array(array=w658, index=0 ("Index")) -> (deleted portion=w656:string, array with subset deleted=w655:string[])  [unwired: 1 in]
        n151 = Concatenate Strings(w666, "-transferfpp-" ("Substring"), w667, w611, ".txt" ("Substring")) -> (w669:string)
        n152 = VISA Write(VISA resource name=w635, write buffer=":PAGE:CHAN:MODE SWE;" ("write buffer (\"\")"), error in (no error)=w634) -> (VISA resource name out=w632:refnum<visa-resource-name>, error out=w633:errorcluster)  [unwired: 1 out]
        n153 = case shown="\"d\", Default" w656 {
          tunnel: [w680 w681] -> w654
          frame "s" {
            w680 = u16 0 items=["Single", "Double"] ("sweep mode")
          }
          frame "d", Default {
            w681 = u16 1 items=["Single", "Double"] ("sweep mode")
          }
        }
        n154 = Fract/Exp String To Number(string=w655) -> (number=w639:dbl[])  [unwired: 3 in, 1 out]
        n155 = String To Path(string=w669) -> (path=w665:path)
        n156 = Index Array(array=w639, index #1=0 ("Index")) -> (element #1=w653:dbl, element #2=w652:dbl, element #3=w651:dbl)  [unwired: 2 in]
        n157 = Delete From Array(array=w639, length=3 ("Length"), index=0 ("Index")) -> (array with subset deleted=w637:dbl[])  [unwired: 1 out]
        n158 = Bundle By Name(cluster=w645, "Gate Start"=w653, "Gate Stop"=w652, "Gate Step (linear only)"=w651, "Gate Compliance"=w663, "Range mode"=w628, "Range"=w627) -> (w629:T6)
        n159 = Index Array(array=w637, index #1=0 ("Index")) -> (element #1=w648:dbl, element #2=w647:dbl, element #3=w646:dbl)  [unwired: 2 in]
        n160 = call <vilib>:"compatOverwrite.vi"("overwrite (F)"=TRUE) -> ("overwrite?"=w616:T8)
        n161 = Bundle By Name(cluster=w644, "Drain Start"=w648, "Drain Stop"=w647, "Drain Step"=w646, "Drain Compliance"=w664, "Range mode"=w626, "Range"=w625) -> (w630:T7)
        n162 = call "4155C Transfer-FPP.vi"("VISA resource name in"=w632, "Gate"=w629, "Drain"=w630, "Timings"=w662, "error in (no error)"=w633, "sweep mode"=w654, "Panel Controls"=w679) -> ("VG"=w670:dbl[], "Outparams"=w624:T9, "VISA Resource Name out"=w660:refnum<visa-resource-name>, "Vprobe2"=w620:dbl[], "ID"=w619:dbl[], "IG"=w618:dbl[], "Vprobe1"=w617:dbl[], "error out"=w661:errorcluster)  [unwired: 13 in]
        n163 = Unbundle By Name(w624) -> ("V2 Step"=w623:dbl, "V2 Start"=w622:dbl, "Number of points"=w621:i32)
        n164 = Open/Create/Replace File(file path (use dialog)=w665, error in=w661, operation (0:open)=w616) -> (refnum out=w676:refnum<file>, error out=w677:errorcluster)  [unwired: 3 in, 1 out]
        n165 = call "4155C Make Big 2d array FPP.vi"("1D Var1"=w670, "1d ID"=w619, "1d Vp2"=w620, "1d IG"=w618, "1d Vp1"=w617, "VAR2 START"=w622, "Number of VAR2 steps"=w621, "VAR2 STEP"=w623, "VAR1 Name"="Vg", "Decimal places in header"=i8 1, "VAR2 Name"="Vd") -> ("Header array"=w672:string[], "Data array"=w673:dbl[][])  [unwired: 15 in]
        n166 = call "4155C Write array to file.vi"("Byte Stream File Refnum"=w676, "Header"=w672, "Data Array"=w673, "error in (no error)"=w677) -> ("dup refnum"=w674:refnum<file>, "error out"=w675:errorcluster)  [unwired: 1 in]
        n167 = Close File(refnum=w674, error in=w675) -> (error out=w659:errorcluster)  [unwired: 1 out]
      }
      frame "output" {
        n168 = Number To Decimal String(number=w711) -> (decimal integer string=w760:string)  [unwired: 1 in]
        n169 = Bundle By Name(cluster=w737, "Emergency Stop"=w762) -> (w772:T1)
        n170 = Delete From Array(array=w752, index=0 ("Index")) -> (deleted portion=w750:string, array with subset deleted=w749:string[])  [unwired: 1 in]
        n171 = Concatenate Strings(w759, w682, w760, w710, "_O.txt" ("Suffix (output)")) -> (w761:string)
        n172 = VISA Write(VISA resource name=w728, write buffer=":PAGE:CHAN:MODE SWE;" ("write buffer (\"\")"), error in (no error)=w725) -> (VISA resource name out=w727:refnum<visa-resource-name>, error out=w726:errorcluster)  [unwired: 1 out]
        n173 = case shown="\"d\", Default" w750 {
          tunnel: [w773 w774] -> w748
          frame "s" {
            w773 = u16 0 items=["Single", "Double"] ("sweep mode")
          }
          frame "d", Default {
            w774 = u16 1 items=["Single", "Double"] ("sweep mode")
          }
        }
        n174 = Fract/Exp String To Number(string=w749) -> (number=w731:dbl[])  [unwired: 3 in, 1 out]
        n175 = String To Path(string=w761) -> (path=w758:path)
        n176 = Index Array(array=w731, index #1=0 ("Index")) -> (element #1=w747:dbl, element #2=w746:dbl, element #3=w745:dbl)  [unwired: 2 in]
        n177 = Delete From Array(array=w731, length=3 ("Length"), index=0 ("Index")) -> (array with subset deleted=w730:dbl[])  [unwired: 1 out]
        n178 = control-ref of="I vs Vd"() -> (w701:refnum<vi>)
        n179 = Bundle By Name(cluster=w739, "Gate Start"=w747, "Gate Stop"=w746, "Gate Step (linear only)"=w745, "Gate Compliance"=w756, "Range mode"=w723, "Range"=w722) -> (w771:T6)
        n180 = Index Array(array=w730, index #1=0 ("Index")) -> (element #1=w742:dbl, element #2=w741:dbl, element #3=w740:dbl)  [unwired: 2 in]
        n181 = call <vilib>:"compatOverwrite.vi"("overwrite (F)"=TRUE) -> ("overwrite?"=w715:T8)
        n182 = Bundle By Name(cluster=w738, "Drain Start"=w742, "Drain Stop"=w741, "Drain Step"=w740, "Drain Compliance"=w757, "Range mode"=w721, "Range"=w724) -> (w770:T7)
        n183 = call "4155C Output.vi"("VISA resource name in"=w727, "Gate"=w771, "Drain"=w770, "Timings"=w755, "error in (no error)"=w726, "SMU4"=w717, "sweep mode"=w748, "Panel controls"=w772) -> ("VD"=w708:dbl[], "Outparams"=w719:T9, "VISA Resource Name out"=w754:refnum<visa-resource-name>, "IS"=w707:dbl[], "ID"=w706:dbl[], "IG"=w705:dbl[], "error out"=w703:errorcluster, "SMU4"=w716:dbl[])  [unwired: 12 in]
        n184 = Unbundle By Name(w719) -> ("V2 Step"=w720:dbl, "V2 Start"=w718:dbl, "Number of points"=w700:i32)
        n185 = call "4155C Split array.vi"("Number of VAR2 steps"=w700, "Y2 data in"=w706, "X data in"=w708, "Y1 data in"=w707, "Y3 data in"=w705, "error in (no error)"=w703) -> ("Array of clusters"=w704:cluster{"Y data in":dbl[], "X data in":dbl[]}[], "error out"=w702:errorcluster)  [unwired: 1 in]
        n186 = local write "I vs Vd"(w704) -> ()
        n187 = call "4155C Config Chart Colours.vi"("Numeric"=w700, "XY Graph 2"=w701) -> ()  [unwired: 6 in]
        n188 = Open/Create/Replace File(file path (use dialog)=w758, error in=w702, operation (0:open)=w715) -> (refnum out=w767:refnum<file>, error out=w768:errorcluster)  [unwired: 3 in, 1 out]
        n189 = call "4155C Make Big 2d array.vi"("1D Var1"=w708, "1d IS"=w707, "1d ID"=w706, "1d IG"=w705, "1d SMU4"=w716, "SMU4"=w717, "VAR2 START"=w718, "Number of VAR2 steps"=w700, "VAR2 STEP"=w720, "VAR1 Name"="Vd", "Decimal places in header"=i8 1, "VAR2 Name"="Vg") -> ("Header array"=w763:string[], "Data array"=w764:dbl[][])  [unwired: 14 in]
        n190 = call "4155C Write array to file.vi"("Byte Stream File Refnum"=w767, "Header"=w763, "Data Array"=w764, "error in (no error)"=w768) -> ("dup refnum"=w765:refnum<file>, "error out"=w766:errorcluster)  [unwired: 1 in]
        n191 = Close File(refnum=w765, error in=w766) -> (error out=w753:errorcluster)  [unwired: 1 out]
      }
      frame "output2" {
        # "Adjusts graph colors."
        # "Adjusts graph colors."
        # "Is off"
        # "Is on"
        # "Ion will be the middle element of the array. The calculation of the index is done only once, since Is, Id, and Ig have the same dimensions."
        # "Ig off"
        # "Ig on"
        # "Is min"
        # "Is max"
        # "Ig min"
        # "Ig max"
        # "abs(Ig)"
        # "abs(Is)"
        # "Id min"
        # "Id max"
        # "Y1: Is\nY2: Id\nY3: Ig"
        # "abs(Id)"
        # "Adjusts graph colors."
        # "Adjusts graph colors."
        # "Id off"
        # "Id on"
        # "Adjusts graph colors."
        # "Time array"
        n192 = Delete From Array(array=w904, index=0 ("Index")) -> (deleted portion=w902:string, array with subset deleted=w901:string[])  [unwired: 1 in]
        n193 = Bundle By Name(cluster=w775, "Emergency Stop"=w913) -> (w866:T1)
        n194 = Number To Decimal String(number=w860) -> (decimal integer string=w859:string)  [unwired: 1 in]
        n195 = case shown="\"d\", Default" w902 {
          tunnel: [w915 w916] -> w900
          frame "s" {
            w915 = u16 0 items=["Single", "Double"] ("sweep mode")
          }
          frame "d", Default {
            w916 = u16 1 items=["Single", "Double"] ("sweep mode")
          }
        }
        n196 = Fract/Exp String To Number(string=w901) -> (number=w886:dbl[])  [unwired: 3 in, 1 out]
        n197 = Concatenate Strings(w911, w776, w859, w857, "_O_1_C_L.txt" ("Suffix (transfer)")) -> (w912:string)
        n198 = VISA Write(VISA resource name=w882, write buffer=":PAGE:CHAN:MODE SWE;" ("write buffer (\"\")"), error in (no error)=w881) -> (VISA resource name out=w879:refnum<visa-resource-name>, error out=w880:errorcluster)  [unwired: 1 out]
        n199 = String To Path(string=w912) -> (path=w910:path)
        n200 = Index Array(array=w886, index #1=0 ("Index")) -> (element #1=w899:dbl, element #2=w898:dbl, element #3=w897:dbl)  [unwired: 2 in]
        n201 = Delete From Array(array=w886, length=3 ("Length"), index=0 ("Index")) -> (array with subset deleted=w884:dbl[])  [unwired: 1 out]
        n202 = Build Array (concatenate)(w856, w852) -> (w802:i32[])
        n203 = Bundle By Name(cluster=w891, "Gate Start"=w899, "Gate Stop"=w898, "Gate Step (linear only)"=w897, "Gate Compliance"=w908, "Range mode"=w875, "Range"=w874) -> (w876:T6)
        n204 = control-ref of="Imax vs time"() -> (w831:refnum<vi>)
        n205 = control-ref of="Imin vs time"() -> (w830:refnum<vi>)
        n206 = control-ref of="Ion vs time"() -> (w799:refnum<vi>)
        n207 = control-ref of="Ioff vs time"() -> (w798:refnum<vi>)
        n208 = control-ref of="I vs Vg"() -> (w861:refnum<vi>)
        n209 = Index Array(array=w884, index #1=0 ("Index")) -> (element #1=w894:dbl, element #2=w893:dbl, element #3=w892:dbl)  [unwired: 2 in]
        n210 = call <vilib>:"compatOverwrite.vi"("overwrite (F)"=TRUE) -> ("overwrite?"=w865:T8)
        n211 = Bundle By Name(cluster=w890, "Drain Start"=w894, "Drain Stop"=w893, "Drain Step"=w892, "Drain Compliance"=w909, "Range mode"=w873, "Range"=w872) -> (w877:T7)
        n212 = call "4155C Output.vi"("VISA resource name in"=w879, "Gate"=w876, "Drain"=w877, "Timings"=w907, "error in (no error)"=w880, "SMU4"=w867, "sweep mode"=w900, "Panel controls"=w866) -> ("VD"=w864:dbl[], "Outparams"=w871:T9, "VISA Resource Name out"=w906:refnum<visa-resource-name>, "IS"=w827:dbl[], "ID"=w829:dbl[], "IG"=w826:dbl[], "error out"=w853:errorcluster, "SMU4"=w868:dbl[])  [unwired: 12 in]
        n213 = Unbundle By Name(w871) -> ("V2 Step"=w870:dbl, "V2 Start"=w869:dbl, "Number of points"=w796:i32)
        n214 = Absolute Value(x=w827) -> (abs(x)=w812:dbl[])
        n215 = Absolute Value(x=w829) -> (abs(x)=w828:dbl[])
        n216 = Absolute Value(x=w826) -> (abs(x)=w815:dbl[])
        n217 = Array Size(array=w828) -> (size(s)=w836:i32)
        n218 = Divide(x=w836, y=2) -> (x/y=w779:dbl)
        n219 = Subtract(x=w779, y=1) -> (x-y=w778:dbl)
        n220 = Array Max & Min(array=w812) -> (max value=w819:dbl, min value=w820:dbl)  [unwired: 2 out]
        n221 = Array Max & Min(array=w828) -> (max value=w862:dbl, min value=w825:dbl)  [unwired: 2 out]
        n222 = Array Max & Min(array=w815) -> (max value=w824:dbl, min value=w823:dbl)  [unwired: 2 out]
        n223 = call "4155C Split array.vi"("Number of VAR2 steps"=w796, "Y2 data in"=w829, "X data in"=w864, "Y1 data in"=w827, "Y3 data in"=w826, "error in (no error)"=w853) -> ("Array of clusters"=w855:cluster{"Y data in":dbl[], "X data in":dbl[]}[], "error out"=w784:errorcluster)  [unwired: 1 in]
        n224 = Index Array(array=w812, index=w778) -> (element=w803:dbl)
        n225 = Index Array(array=w812, index=0) -> (element=w804:dbl)
        n226 = Index Array(array=w828, index=w778) -> (element=w805:dbl)
        n227 = Index Array(array=w828, index=0) -> (element=w806:dbl)
        n228 = Index Array(array=w815, index=w778) -> (element=w808:dbl)
        n229 = Index Array(array=w815, index=0) -> (element=w807:dbl)
        n230 = local write "Ig max"(w824) -> ()
        n231 = local write "Ig min"(w823) -> ()
        n232 = local write "Is max"(w819) -> ()
        n233 = local write "Is min"(w820) -> ()
        n234 = local write "Id max"(w862) -> ()
        n235 = local write "Id min"(w825) -> ()
        n236 = local write "I vs Vd"(w855) -> ()
        n237 = Build Array (concatenate)(w818, w819) -> (w797:dbl[])
        n238 = Build Array (concatenate)(w817, w820) -> (w795:dbl[])
        n239 = local write "Is off"(w804) -> ()
        n240 = local write "Is on"(w803) -> ()
        n241 = Build Array (concatenate)(w863, w862) -> (w794:dbl[])
        n242 = Build Array (concatenate)(w850, w825) -> (w793:dbl[])
        n243 = Build Array (concatenate)(w822, w824) -> (w792:dbl[])
        n244 = Build Array (concatenate)(w821, w823) -> (w791:dbl[])
        n245 = Build Array (concatenate)(w810, w803) -> (w790:dbl[])
        n246 = Build Array (concatenate)(w809, w804) -> (w789:dbl[])
        n247 = Build Array (concatenate)(w832, w805) -> (w788:dbl[])
        n248 = Build Array (concatenate)(w833, w806) -> (w787:dbl[])
        n249 = Build Array (concatenate)(w814, w808) -> (w786:dbl[])
        n250 = Build Array (concatenate)(w813, w807) -> (w785:dbl[])
        n251 = local write "Ig off"(w807) -> ()
        n252 = local write "Ig on"(w808) -> ()
        n253 = local write "Id off"(w806) -> ()
        n254 = local write "Id on"(w805) -> ()
        n255 = call "4155C Split array.vi"("Number of VAR2 steps"=w796, "Y2 data in"=w788, "X data in"=w802, "Y1 data in"=w790, "Y3 data in"=w786, "error in (no error)"=w784) -> ("Array of clusters"=w800:cluster{"Y data in":dbl[], "X data in":dbl[]}[], "error out"=w783:errorcluster)  [unwired: 1 in]
        n256 = call "4155C Split array.vi"("Number of VAR2 steps"=w796, "Y2 data in"=w787, "X data in"=w802, "Y1 data in"=w789, "Y3 data in"=w785, "error in (no error)"=w783) -> ("Array of clusters"=w801:cluster{"Y data in":dbl[], "X data in":dbl[]}[], "error out"=w782:errorcluster)  [unwired: 1 in]
        n257 = call "4155C Split array.vi"("Number of VAR2 steps"=w796, "Y2 data in"=w794, "X data in"=w802, "Y1 data in"=w797, "Y3 data in"=w792, "error in (no error)"=w782) -> ("Array of clusters"=w854:cluster{"Y data in":dbl[], "X data in":dbl[]}[], "error out"=w781:errorcluster)  [unwired: 1 in]
        n258 = call "4155C Split array.vi"("Number of VAR2 steps"=w796, "Y2 data in"=w793, "X data in"=w802, "Y1 data in"=w795, "Y3 data in"=w791, "error in (no error)"=w781) -> ("Array of clusters"=w851:cluster{"Y data in":dbl[], "X data in":dbl[]}[], "error out"=w780:errorcluster)  [unwired: 1 in]
        n259 = Open/Create/Replace File(file path (use dialog)=w910, error in=w780, operation (0:open)=w865) -> (refnum out=w848:refnum<file>, error out=w846:errorcluster)  [unwired: 3 in, 1 out]
        n260 = call "4155C Make Big 2d array.vi"("1D Var1"=w864, "1d IS"=w827, "1d ID"=w829, "1d IG"=w826, "1d SMU4"=w868, "SMU4"=w867, "VAR2 START"=w869, "Number of VAR2 steps"=w796, "VAR2 STEP"=w870, "VAR1 Name"="Vd", "Decimal places in header"=i8 1, "VAR2 Name"="Vg") -> ("Header array"=w849:string[], "Data array"=w847:dbl[][])  [unwired: 14 in]
        n261 = local write "Imax vs time"(w854) -> ()
        n262 = local write "Imin vs time"(w851) -> ()
        n263 = local write "Ion vs time"(w800) -> ()
        n264 = local write "Ioff vs time"(w801) -> ()
        n265 = call "4155C Config Chart Colours.vi"("Numeric"=w796, "XY Graph 2"=w831) -> ()  [unwired: 6 in]
        n266 = call "4155C Config Chart Colours.vi"("Numeric"=w796, "XY Graph 2"=w830) -> ()  [unwired: 6 in]
        n267 = call "4155C Config Chart Colours.vi"("Numeric"=w796, "XY Graph 2"=w799) -> ()  [unwired: 6 in]
        n268 = call "4155C Config Chart Colours.vi"("Numeric"=w796, "XY Graph 2"=w798) -> ()  [unwired: 6 in]
        n269 = call "4155C Config Chart Colours.vi"("Numeric"=w796, "XY Graph 2"=w861) -> ()  [unwired: 6 in]
        n270 = call "4155C Write array to file.vi"("Byte Stream File Refnum"=w848, "Header"=w849, "Data Array"=w847, "error in (no error)"=w846) -> ("dup refnum"=w845:refnum<file>, "error out"=w844:errorcluster)  [unwired: 1 in]
        n271 = Close File(refnum=w845, error in=w844) -> (error out=w905:errorcluster)  [unwired: 1 out]
      }
      frame "output-fpp" {
        n272 = Number To Decimal String(number=w937) -> (decimal integer string=w991:string)  [unwired: 1 in]
        n273 = Bundle By Name(cluster=w967, "Emergency Stop"=w994) -> (w1004:T1)
        n274 = Delete From Array(array=w982, index=0 ("Index")) -> (deleted portion=w980:string, array with subset deleted=w979:string[])  [unwired: 1 in]
        n275 = VISA Write(VISA resource name=w958, write buffer=":PAGE:CHAN:MODE SWE;" ("write buffer (\"\")"), error in (no error)=w955) -> (VISA resource name out=w957:refnum<visa-resource-name>, error out=w956:errorcluster)  [unwired: 1 out]
        n276 = Concatenate Strings(w990, "-outputfpp-" ("Substring"), w991, w936, ".txt" ("Substring")) -> (w993:string)
        n277 = case shown="\"d\", Default" w980 {
          tunnel: [w1005 w1006] -> w978
          frame "s" {
            w1005 = u16 0 items=["Single", "Double"] ("sweep mode")
          }
          frame "d", Default {
            w1006 = u16 1 items=["Single", "Double"] ("sweep mode")
          }
        }
        n278 = Fract/Exp String To Number(string=w979) -> (number=w961:dbl[])  [unwired: 3 in, 1 out]
        n279 = String To Path(string=w993) -> (path=w989:path)
        n280 = Index Array(array=w961, index #1=0 ("Index")) -> (element #1=w977:dbl, element #2=w976:dbl, element #3=w975:dbl)  [unwired: 2 in]
        n281 = Delete From Array(array=w961, length=3 ("Length"), index=0 ("Index")) -> (array with subset deleted=w960:dbl[])  [unwired: 1 out]
        n282 = Bundle By Name(cluster=w969, "Gate Start"=w977, "Gate Stop"=w976, "Gate Step (linear only)"=w975, "Gate Compliance"=w987, "Range mode"=w953, "Range"=w952) -> (w1003:T6)
        n283 = Index Array(array=w960, index #1=0 ("Index")) -> (element #1=w972:dbl, element #2=w971:dbl, element #3=w970:dbl)  [unwired: 2 in]
        n284 = call <vilib>:"compatOverwrite.vi"("overwrite (F)"=TRUE) -> ("overwrite?"=w941:T8)
        n285 = Bundle By Name(cluster=w968, "Drain Start"=w972, "Drain Stop"=w971, "Drain Step"=w970, "Drain Compliance"=w988, "Range mode"=w951, "Range"=w954) -> (w1002:T7)
        n286 = call "4155C Output-FPP.vi"("VISA resource name in"=w957, "Gate"=w1003, "Drain"=w1002, "Timings"=w986, "error in (no error)"=w956, "sweep mode"=w978, "Panel controls"=w1004) -> ("VD"=w946:dbl[], "Outparams"=w949:T9, "VISA Resource Name out"=w984:refnum<visa-resource-name>, "Vprobe2"=w945:dbl[], "ID"=w944:dbl[], "IG"=w943:dbl[], "Vprobe1"=w942:dbl[], "error out"=w985:errorcluster)  [unwired: 13 in]
        n287 = Unbundle By Name(w949) -> ("V2 Step"=w950:dbl, "V2 Start"=w948:dbl, "Number of points"=w947:i32)
        n288 = Open/Create/Replace File(file path (use dialog)=w989, error in=w985, operation (0:open)=w941) -> (refnum out=w999:refnum<file>, error out=w1000:errorcluster)  [unwired: 3 in, 1 out]
        n289 = call "4155C Make Big 2d array FPP.vi"("1D Var1"=w946, "1d ID"=w944, "1d Vp2"=w945, "1d IG"=w943, "1d Vp1"=w942, "VAR2 START"=w948, "Number of VAR2 steps"=w947, "VAR2 STEP"=w950, "VAR1 Name"="Vd", "Decimal places in header"=i8 1, "VAR2 Name"="Vg") -> ("Header array"=w995:string[], "Data array"=w996:dbl[][])  [unwired: 15 in]
        n290 = call "4155C Write array to file.vi"("Byte Stream File Refnum"=w999, "Header"=w995, "Data Array"=w996, "error in (no error)"=w1000) -> ("dup refnum"=w997:refnum<file>, "error out"=w998:errorcluster)  [unwired: 1 in]
        n291 = Close File(refnum=w997, error in=w998) -> (error out=w983:errorcluster)  [unwired: 1 out]
      }
      frame "itime" {
        n292 = Delete From Array(array=w1009, index=1) -> (deleted portion=w1008:string)  [unwired: 1 in, 1 out]
        n293 = Delete From Array(array=w1009, index=0 ("Index")) -> (deleted portion=w1043:string)  [unwired: 1 in, 1 out]
        n294 = Fract/Exp String To Number(string=w1008) -> (number=w1007:dbl)  [unwired: 3 in, 1 out]
        n295 = case shown="\"l\"" w1043 {
          tunnel: w1042 -> [w1048 w1050 w1054]
          tunnel: [w1047 w1049 w1053] -> w1035
          tunnel: w1007 -> [w1045 _ w1052]
          frame "s" {
            w1046 = u32 0 items=["short  ", "medium  ", "long  "] ("integration time 2")
            n296 = Bundle By Name(cluster=w1048, "integration time"=w1046, "Short/Long integration time"=w1045) -> (w1047:T5)
          }
          frame "m", Default {
            w1051 = u32 1 items=["short  ", "medium  ", "long  "] ("integration time 2")
            n297 = Bundle By Name(cluster=w1050, "integration time"=w1051) -> (w1049:T5)
          }
          frame "l" {
            w1055 = u32 2 items=["short  ", "medium  ", "long  "] ("integration time 2")
            n298 = Bundle By Name(cluster=w1054, "integration time"=w1055, "Short/Long integration time"=w1052) -> (w1053:T5)
          }
        }
      }
      frame "pulsed" {
        n299 = Delete From Array(array=w1089, index=0 ("Index")) -> (deleted portion=w1090:string, array with subset deleted=w1077:string[])  [unwired: 1 in]
        n300 = case shown="\"on\", Default" w1090 {
          tunnel: w1088 -> [w1100 w1103]
          tunnel: [w1099 w1102] -> w1081
          tunnel: w1077 -> [w1097 _]
          frame "on", Default {
            w1098 = u16 1 items=["Continuous", "Pulsed"] ("sweep method")
            n301 = Fract/Exp String To Number(string=w1097) -> (number=w1095:dbl[])  [unwired: 3 in, 1 out]
            n302 = Index Array(array=w1095, index #1=0 ("Index")) -> (element #1=w1094:dbl, element #2=w1093:dbl, element #3=w1092:dbl)  [unwired: 2 in]
            n303 = Bundle By Name(cluster=w1100, "sweep method"=w1098, "Pulse period"=w1094, "Base voltage"=w1093, "Pulse width"=w1092) -> (w1099:T5)
          }
          frame "off" {
            w1101 = u16 0 items=["Continuous", "Pulsed"] ("sweep method")
            n304 = Bundle By Name(cluster=w1103, "sweep method"=w1101) -> (w1102:T5)
          }
        }
      }
      frame "gaterangemode" {
        n305 = Delete From Array(array=w1135, index=0 ("Index")) -> (deleted portion=w1136:string)  [unwired: 1 in, 1 out]
        n306 = case shown="\"f\"" w1136 {
          tunnel: [w1138 w1139 w1140] -> w1125
          frame "a", Default {
            w1138 = u16 0 items=["Auto", "Limited", "Fixed"] ("Gate Range\nmode 2")
          }
          frame "f" {
            w1139 = u16 2 items=["Auto", "Limited", "Fixed"] ("Gate Range\nmode 2")
          }
          frame "l" {
            w1140 = u16 1 items=["Auto", "Limited", "Fixed"] ("Gate Range\nmode 2")
          }
        }
      }
      frame "gaterange" {
        (unwired) u8 11 items=["10fA  ", "100fA  ", "1nA  ", "10nA", "100nA", "1uA", "10uA", "100uA", "1mA", "10mA", "100mA", "1A"] ("Gate Range 2")
        n307 = Delete From Array(array=w1179, index=0 ("Index")) -> (deleted portion=w1169:string)  [unwired: 1 in, 1 out]
        n308 = Scan Value(string=w1169, format string="") -> (value=w1167:dbl)  [unwired: 1 in, 1 out]
        n309 = Logarithm Base 10(1:w1167) -> (0:w1166:dbl)
        n310 = Round To Nearest(number=w1166) -> (nearest integer value=w1165:dbl)
        n311 = Add(x=w1165, y=11.0) -> (x+y=w1163:dbl)
        n312 = To Unsigned Byte Integer(number=w1163) -> (unsigned 8bit integer=w1162:u8)
      }
      frame "drainrange" {
        (unwired) u8 11 items=["10fA  ", "100fA  ", "1nA  ", "10nA", "100nA", "1uA", "10uA", "100uA", "1mA", "10mA", "100mA", "1A"] ("Gate Range 2")
        n313 = Delete From Array(array=w1219, index=0 ("Index")) -> (deleted portion=w1210:string)  [unwired: 1 in, 1 out]
        n314 = Scan Value(string=w1210, format string="") -> (value=w1208:dbl)  [unwired: 1 in, 1 out]
        n315 = Logarithm Base 10(1:w1208) -> (0:w1207:dbl)
        n316 = Round To Nearest(number=w1207) -> (nearest integer value=w1206:dbl)
        n317 = Add(x=w1206, y=11.0) -> (x+y=w1204:dbl)
        n318 = To Unsigned Byte Integer(number=w1204) -> (unsigned 8bit integer=w1203:u8)
      }
      frame "drainrangemode" {
        n319 = Delete From Array(array=w1252, index=0 ("Index")) -> (deleted portion=w1253:string)  [unwired: 1 in, 1 out]
        n320 = case shown="\"f\"" w1253 {
          tunnel: [w1255 w1256 w1257] -> w1242
          frame "a", Default {
            w1255 = u16 0 items=["Auto", "Limited", "Fixed"] ("Gate Range\nmode 2")
          }
          frame "f" {
            w1256 = u16 2 items=["Auto", "Limited", "Fixed"] ("Gate Range\nmode 2")
          }
          frame "l" {
            w1257 = u16 1 items=["Auto", "Limited", "Fixed"] ("Gate Range\nmode 2")
          }
        }
      }
      frame "Error", Default {
      }
      frame "logfile" {
        n321 = Number To Decimal String(number=w1310) -> (decimal integer string=w1345:string)  [unwired: 1 in]
        n322 = Concatenate Strings(w1344, "logfile" ("Substring"), w1345, w1308, ".txt" ("Substring")) -> (w1342:string)
        n323 = String To Path(string=w1342) -> (path=w1315:path)
        n324 = Unbundle(w1341) -> ("integration time"=w1340:u32, "Short/Long integration time"=w1339:dbl, "hold time (sec)"=w1338:dbl, "delay time (sec)"=w1337:dbl, "Step Time (0 disables)"=w1336:dbl, "sweep method"=w1335:u16, "Pulse period"=w1334:dbl, "Base voltage"=w1333:dbl, "Pulse width"=w1332:dbl)
        n325 = Build Array(w1340, w1339, w1338, w1337, w1336, w1335, w1334, w1333, w1332, w1326, w1327, w1328, w1329, w1330, w1331) -> (w1319:dbl[])
        n326 = Insert Into Array(array=dbl[][] [] ("Input Array"), new element=w1319) -> (w1318:dbl[][])  [unwired: 2 in]
        n327 = call <vilib>:"compatOverwrite.vi"("overwrite (F)"=TRUE) -> ("overwrite?"=w1313:T8)
        n328 = Open/Create/Replace File(file path (use dialog)=w1315, error in=w1317, operation (0:open)=w1313) -> (refnum out=w1323:refnum<file>, error out=w1322:errorcluster)  [unwired: 3 in, 1 out]
        n329 = call "4155C Write array to file.vi"("Byte Stream File Refnum"=w1323, "Header"=string[] ["Int Time", "Short/Long Itime", "Hold time", "Delay time", "Step time", "Sweep method", "Pulse period", "Base Voltage", "Pulse width", "Drain compliance", "Gate compliance", "Gate range mode", "Gate range", "S/D range mode", "S/D range"], "Data Array"=w1318, "error in (no error)"=w1322) -> ("dup refnum"=w1325:refnum<file>, "error out"=w1324:errorcluster)  [unwired: 1 in]
        n330 = Close File(refnum=w1325, error in=w1324) -> (error out=w1316:errorcluster)  [unwired: 1 out]
      }
      frame "sample" {
        n331 = Number To Decimal String(number=w1368) -> (decimal integer string=w1416:string)  [unwired: 1 in]
        n332 = Fract/Exp String To Number(string=w1413) -> (number=w1374:dbl[])  [unwired: 3 in, 1 out]
        n333 = Concatenate Strings(w1391, "-sample-" ("Substring"), w1416, w1366, ".txt" ("Substring")) -> (w1414:string)
        n334 = Index Array(array=w1374, index=0 ("Index")) -> (element=w1411:dbl)
        n335 = String To Path(string=w1414) -> (path=w1395:path)
        n336 = Index Array(array=w1374, index=2 ("Index")) -> (element=w1407:dbl)
        n337 = Index Array(array=w1374, index=3 ("Index")) -> (element=w1376:dbl)
        n338 = Index Array(array=w1374, index=4 ("Index")) -> (element=w1373:dbl)
        n339 = call "4155C Config Sampling Measurements.vi"("Sampling interval"=w1373, "Sample time"=w1376, "Display on/off"=TRUE, "Timings"=w1382, "Num Points"=w1407, "error in (no error)"=w1418, "Drain Compliance"=w1417, "Gate Compliance"=w1392, "VISA session"=w1419) -> ("error out"=w1420:errorcluster, "dup VISA resource name"=w1421:refnum<visa-resource-name>)  [unwired: 1 in]
        n340 = Index Array(array=w1374, index=1 ("Index")) -> (element=w1408:dbl)
        n341 = call "4155C Take Sample.vi"("Emergency Stop"=w1388, "error in (no error)"=w1420, "Vd"=w1408, "Vg"=w1411, "VISA resource name in"=w1421) -> ("error out"=w1386:errorcluster, "Id"=w1423:dbl[], "Ig"=w1397:dbl[], "VISA Resource Name out"=w1384:refnum<visa-resource-name>, "Is"=w1422:dbl[], "Time"=w1401:dbl[])  [unwired: 1 in]
        n342 = Insert Into Array(array=dbl[][] [] ("Input Array"), new element=w1401) -> (w1400:dbl[][])  [unwired: 2 in]
        n343 = Insert Into Array(array=w1400, new element=w1397) -> (w1399:dbl[][])  [unwired: 2 in]
        n344 = Insert Into Array(array=w1399, new element=w1423) -> (w1398:dbl[][])  [unwired: 2 in]
        n345 = VISA Write(VISA resource name=w1384, write buffer=":DISP ON" ("write buffer (\"\")"), error in (no error)=w1386) -> (VISA resource name out=w1383:refnum<visa-resource-name>, error out=w1385:errorcluster)  [unwired: 1 out]
        n346 = Insert Into Array(array=w1398, new element=w1422) -> (w1390:dbl[][])  [unwired: 2 in]
        n347 = Transpose 2D Array(2D array=w1390) -> (transposed array=w1389:dbl[][])
        n348 = call <vilib>:"compatOverwrite.vi"("overwrite (F)"=TRUE) -> ("overwrite?"=w1371:T8)
        n349 = Open/Create/Replace File(file path (use dialog)=w1395, error in=w1385, operation (0:open)=w1371) -> (refnum out=w1404:refnum<file>, error out=w1403:errorcluster)  [unwired: 3 in, 1 out]
        n350 = call "4155C Write array to file.vi"("Byte Stream File Refnum"=w1404, "Header"=string[] ["Time /s", "Ig /A", "Id /A", "Is /A"], "Data Array"=w1389, "error in (no error)"=w1403) -> ("dup refnum"=w1406:refnum<file>, "error out"=w1405:errorcluster)  [unwired: 1 in]
        n351 = Close File(refnum=w1406, error in=w1405) -> (error out=w1393:errorcluster)  [unwired: 1 out]
      }
      frame "samplei" {
        n352 = Number To Decimal String(number=w1445) -> (decimal integer string=w1496:string)  [unwired: 1 in]
        n353 = Concatenate Strings(w1475, "-samplei-" ("Substring"), w1496, w1444, ".txt" ("Substring")) -> (w1494:string)
        n354 = Fract/Exp String To Number(string=w1493) -> (number=w1460:dbl[])  [unwired: 3 in, 1 out]
        n355 = String To Path(string=w1494) -> (path=w1478:path)
        n356 = Index Array(array=w1460, index=4 ("Index")) -> (element=w1454:dbl)
        n357 = Index Array(array=w1460, index=3 ("Index")) -> (element=w1455:dbl)
        n358 = Index Array(array=w1460, index=1 ("Index")) -> (element=w1457:dbl)
        n359 = Index Array(array=w1460, index=0 ("Index")) -> (element=w1458:dbl)
        n360 = Index Array(array=w1460, index=2 ("Index")) -> (element=w1456:dbl)
        n361 = call "4155C Config SamplingI Measurements.vi"("Sample time"=w1456, "Display on/off"=TRUE, "Timings"=w1467, "Num Points"=w1457, "error in (no error)"=w1498, "Sampling interval"=w1455, "VISA session"=w1499) -> ("error out"=w1500:errorcluster, "dup VISA resource name"=w1501:refnum<visa-resource-name>)  [unwired: 3 in]
        n362 = call "4155C Take SampleI.vi"("Emergency Stop"=w1472, "error in (no error)"=w1500, "Idg 2"=w1458, "Vdg compliance 2"=w1454, "VISA resource name in"=w1501) -> ("error out"=w1470:errorcluster, "Idg"=w1503:dbl[], "Vdg"=w1480:dbl[], "VISA Resource Name out"=w1468:refnum<visa-resource-name>, "Is"=w1502:dbl[], "Time"=w1484:dbl[])  [unwired: 1 in]
        n363 = Insert Into Array(array=dbl[][] [] ("Input Array"), new element=w1484) -> (w1483:dbl[][])  [unwired: 2 in]
        n364 = Insert Into Array(array=w1483, new element=w1480) -> (w1482:dbl[][])  [unwired: 2 in]
        n365 = Insert Into Array(array=w1482, new element=w1503) -> (w1481:dbl[][])  [unwired: 2 in]
        n366 = VISA Write(VISA resource name=w1468, write buffer=":DISP ON" ("write buffer (\"\")"), error in (no error)=w1470) -> (VISA resource name out=w1453:refnum<visa-resource-name>, error out=w1469:errorcluster)  [unwired: 1 out]
        n367 = Insert Into Array(array=w1481, new element=w1502) -> (w1474:dbl[][])  [unwired: 2 in]
        n368 = call <vilib>:"compatOverwrite.vi"("overwrite (F)"=TRUE) -> ("overwrite?"=w1448:T8)
        n369 = Open/Create/Replace File(file path (use dialog)=w1478, error in=w1469, operation (0:open)=w1448) -> (refnum out=w1487:refnum<file>, error out=w1486:errorcluster)  [unwired: 3 in, 1 out]
        n370 = Transpose 2D Array(2D array=w1474) -> (transposed array=w1473:dbl[][])
        n371 = call "4155C Write array to file.vi"("Byte Stream File Refnum"=w1487, "Header"=string[] ["Time /s", "Vdg /V", "Idg /A", "Is /A"], "Data Array"=w1473, "error in (no error)"=w1486) -> ("dup refnum"=w1489:refnum<file>, "error out"=w1488:errorcluster)  [unwired: 1 in]
        n372 = Close File(refnum=w1489, error in=w1488) -> (error out=w1451:errorcluster)  [unwired: 1 out]
        n373 = VISA Write(VISA resource name=w1453, write buffer=";:PAGE:SCON:STAN OFF;:PAGE:CHAN:VSU2:DIS;" ("write buffer (\"\")"), error in (no error)=w1451) -> (VISA resource name out=w1449:refnum<visa-resource-name>, error out=w1450:errorcluster)  [unwired: 1 out]
      }
      frame "#" {
        n374 = VISA Write(VISA resource name=w1529, write buffer=":DISP ON" ("write buffer (\"\")"), error in (no error)=w1528) -> (VISA resource name out=w1527:refnum<visa-resource-name>, error out=w1526:errorcluster)  [unwired: 1 out]
      }
      frame "stressV" {
        n375 = Number To Decimal String(number=w1558) -> (decimal integer string=w1599:string)  [unwired: 1 in]
        n376 = Concatenate Strings(w1583, "-stressV-" ("Substring"), w1599, w1557, ".txt" ("Substring")) -> (w1597:string)
        n377 = Fract/Exp String To Number(string=w1596) -> (number=w1569:dbl[])  [unwired: 3 in, 1 out]
        n378 = String To Path(string=w1597) -> (path=w1587:path)
        n379 = Index Array(array=w1569, index=3 ("Index")) -> (element=w1566:dbl)
        n380 = Index Array(array=w1569, index=1 ("Index")) -> (element=w1564:dbl)
        n381 = Index Array(array=w1569, index=0 ("Index")) -> (element=w1563:dbl)
        n382 = Index Array(array=w1569, index=4 ("Index")) -> (element=w1568:dbl)
        n383 = Index Array(array=w1569, index=2 ("Index")) -> (element=w1565:dbl)
        n384 = call "4155C Config V Stress.vi"("VISA session"=w1602, "ID compliance"=w1566, "VD"=w1564, "VG"=w1563, "IG compliance"=w1565, "error in (no error)"=w1601, "Display on/off"=TRUE) -> ("dup VISA resource name"=w1604:refnum<visa-resource-name>, "error out"=w1603:errorcluster)
        n385 = call "4155C Apply Stress.vi"("error in (no error)"=w1603, "Duration"=w1568, "Emergency Stop"=w1582, "VISA resource name in"=w1604) -> ("error out"=w1580:errorcluster, "VISA Resource Name out"=w1578:refnum<visa-resource-name>)
        n386 = VISA Write(VISA resource name=w1578, write buffer=":DISP ON" ("write buffer (\"\")"), error in (no error)=w1580) -> (VISA resource name out=w1577:refnum<visa-resource-name>, error out=w1579:errorcluster)  [unwired: 1 out]
        n387 = call <vilib>:"compatOverwrite.vi"("overwrite (F)"=TRUE) -> ("overwrite?"=w1562:T8)
        n388 = Open/Create/Replace File(file path (use dialog)=w1587, error in=w1579, operation (0:open)=w1562) -> (refnum out=w1590:refnum<file>, error out=w1589:errorcluster)  [unwired: 3 in, 1 out]
        n389 = call "4155C Write array to file.vi"("Byte Stream File Refnum"=w1590, "Header"=string[] ["V stress completed successfully", ""], "error in (no error)"=w1589) -> ("dup refnum"=w1592:refnum<file>, "error out"=w1591:errorcluster)  [unwired: 2 in]
        n390 = Close File(refnum=w1592, error in=w1591) -> (error out=w1585:errorcluster)  [unwired: 1 out]
      }
      frame "stressI" {
        n391 = Number To Decimal String(number=w1625) -> (decimal integer string=w1662:string)  [unwired: 1 in]
        n392 = Concatenate Strings(w1646, "-stressI-" ("Substring"), w1662, w1624, ".txt" ("Substring")) -> (w1660:string)
        n393 = Fract/Exp String To Number(string=w1659) -> (number=w1634:dbl[])  [unwired: 3 in, 1 out]
        n394 = Index Array(array=w1634, index=1 ("Index")) -> (element=w1630:dbl)
        n395 = Index Array(array=w1634, index=0 ("Index")) -> (element=w1631:dbl)
        n396 = call "4155C Config I Stress.vi"("VISA session"=w1665, "IDG"=w1631, "VDG compliance"=w1630, "error in (no error)"=w1664, "Display on/off"=TRUE) -> ("dup VISA resource name"=w1667:refnum<visa-resource-name>, "error out"=w1666:errorcluster)
        n397 = Index Array(array=w1634, index=2 ("Index")) -> (element=w1632:dbl)
        n398 = String To Path(string=w1660) -> (path=w1650:path)
        n399 = call "4155C Apply Stress.vi"("error in (no error)"=w1666, "Duration"=w1632, "Emergency Stop"=w1645, "VISA resource name in"=w1667) -> ("error out"=w1643:errorcluster, "VISA Resource Name out"=w1641:refnum<visa-resource-name>)
        n400 = VISA Write(VISA resource name=w1641, write buffer=":DISP ON" ("write buffer (\"\")"), error in (no error)=w1643) -> (VISA resource name out=w1640:refnum<visa-resource-name>, error out=w1642:errorcluster)  [unwired: 1 out]
        n401 = call <vilib>:"compatOverwrite.vi"("overwrite (F)"=TRUE) -> ("overwrite?"=w1629:T8)
        n402 = Open/Create/Replace File(file path (use dialog)=w1650, error in=w1642, operation (0:open)=w1629) -> (refnum out=w1653:refnum<file>, error out=w1652:errorcluster)  [unwired: 3 in, 1 out]
        n403 = call "4155C Write array to file.vi"("Byte Stream File Refnum"=w1653, "Header"=string[] ["I stress completed successfully", ""], "error in (no error)"=w1652) -> ("dup refnum"=w1655:refnum<file>, "error out"=w1654:errorcluster)  [unwired: 2 in]
        n404 = Close File(refnum=w1655, error in=w1654) -> (error out=w1648:errorcluster)  [unwired: 1 out]
      }
      frame "vsu2pulse" {
        n405 = Number To Decimal String(number=w1688) -> (decimal integer string=w1723:string)  [unwired: 1 in]
        n406 = Concatenate Strings(w1708, "-vsu2-" ("Substring"), w1723, w1687, ".txt" ("Substring")) -> (w1721:string)
        n407 = Fract/Exp String To Number(string=w1720) -> (number=w1696:dbl[])  [unwired: 3 in, 1 out]
        n408 = String To Path(string=w1721) -> (path=w1712:path)
        n409 = Index Array(array=w1696, index=1 ("Index")) -> (element=w1695:dbl)
        n410 = Index Array(array=w1696, index=0 ("Index")) -> (element=w1693:dbl)
        n411 = call "4155C Config VSU2 Stress.vi"("error in (no error)"=w1725, "VSU2"=w1693, "Display on/off"=TRUE, "VISA session"=w1726) -> ("error out"=w1727:errorcluster, "dup VISA resource name"=w1728:refnum<visa-resource-name>)
        n412 = call "4155C Apply Stress.vi"("error in (no error)"=w1727, "Duration"=w1695, "Emergency Stop"=w1707, "VISA resource name in"=w1728) -> ("error out"=w1705:errorcluster, "VISA Resource Name out"=w1703:refnum<visa-resource-name>)
        n413 = VISA Write(VISA resource name=w1703, write buffer=":DISP ON" ("write buffer (\"\")"), error in (no error)=w1705) -> (VISA resource name out=w1702:refnum<visa-resource-name>, error out=w1704:errorcluster)  [unwired: 1 out]
        n414 = call <vilib>:"compatOverwrite.vi"("overwrite (F)"=TRUE) -> ("overwrite?"=w1692:T8)
        n415 = Open/Create/Replace File(file path (use dialog)=w1712, error in=w1704, operation (0:open)=w1692) -> (refnum out=w1715:refnum<file>, error out=w1714:errorcluster)  [unwired: 3 in, 1 out]
        n416 = call "4155C Write array to file.vi"("Byte Stream File Refnum"=w1715, "Header"=string[] ["VSU2 pulse completed successfully", ""], "error in (no error)"=w1714) -> ("dup refnum"=w1717:refnum<file>, "error out"=w1716:errorcluster)  [unwired: 2 in]
        n417 = Close File(refnum=w1717, error in=w1716) -> (error out=w1710:errorcluster)  [unwired: 1 out]
      }
      frame "sample-fpp" {
        w1760 = string[] ["Time /s", "Id VgVd /A", "Ig VgVd /A", "Vp1 VgVd /V", "Vp2 VgVd /V"] ("Header")
        w1764 = "%d" ("format string")
        n418 = Number To Decimal String(number=w1749) -> (decimal integer string=w1812:string)  [unwired: 1 in]
        n419 = Fract/Exp String To Number(string=w1809) -> (number=w1797:dbl[])  [unwired: 3 in, 1 out]
        n420 = Concatenate Strings(w1803, "-samplefpp-" ("Substring"), w1812, w1748, ".txt" ("Substring")) -> (w1810:string)
        n421 = String To Path(string=w1810) -> (path=w1772:path)
        n422 = Index Array(array=w1797, index=0 ("Index")) -> (element=w1758:dbl)
        n423 = Index Array(array=w1797, index=1 ("Index")) -> (element=w1757:dbl)
        n424 = Index Array(array=w1797, index=2 ("Index")) -> (element=w1805:dbl)
        n425 = Index Array(array=w1797, index=3 ("Index")) -> (element=w1795:dbl)
        n426 = call "4155C Config Sampling Measurements FPP.vi"("VISA session"=w1815, "Num Points"=w1805, "Vg"=w1758, "Display on/off"=TRUE, "Gate Compliance"=w1804, "Drain Compliance"=w1813, "Standby"="Standby", "error in (no error)"=w1814, "Timings"=w1802, "Vd"=w1757, "Sample time"=w1795) -> ("dup VISA resource name"=w1774:refnum<visa-resource-name>, "error out"=w1773:errorcluster)  [unwired: 3 in]
        n427 = Number To Decimal String(number=w1758) -> (decimal integer string=w1784:string)  [unwired: 1 in]
        n428 = call "4155C Take Sample FPP.vi"("VISA resource name in"=w1774, "error in (no error)"=w1773, "Emergency Stop"=w1775) -> ("Time"=w1779:dbl[], "Vp1"=w1789:dbl[], "VISA Resource Name out"=w1755:refnum<visa-resource-name>, "Ig"=w1777:dbl[], "Id"=w1778:dbl[], "Vp2"=w1787:dbl[], "error out"=w1776:errorcluster)  [unwired: 10 in]
        n429 = Insert Into Array(array=dbl[][] [] ("Input Array"), new element=w1779) -> (w1793:dbl[][])  [unwired: 2 in]
        n430 = Number To Decimal String(number=w1757) -> (decimal integer string=w1782:string)  [unwired: 1 in]
        n431 = Insert Into Array(array=w1793, new element=w1778) -> (w1792:dbl[][])  [unwired: 2 in]
        n432 = Concatenate Strings("(Vg = " ("Substring"), w1784, "V, Vd = " ("Substring"), w1782, "V)" ("Substring")) -> (w1780:string)
        n433 = Insert Into Array(array=w1792, new element=w1777) -> (w1791:dbl[][])  [unwired: 2 in]
        n434 = Insert Into Array(array=w1791, new element=w1789) -> (w1788:dbl[][])  [unwired: 2 in]
        n435 = Insert Into Array(array=w1788, new element=w1787) -> (w1756:dbl[][])  [unwired: 2 in]
        n436 = Transpose 2D Array(2D array=w1756) -> (transposed array=w1786:dbl[][])
        n437 = call <vilib>:"compatOverwrite.vi"("overwrite (F)"=TRUE) -> ("overwrite?"=w1753:T8)
        n438 = Open/Create/Replace File(file path (use dialog)=w1772, error in=w1776, operation (0:open)=w1753) -> (refnum out=w1769:refnum<file>, error out=w1770:errorcluster)  [unwired: 3 in, 1 out]
        n439 = Array To Spreadsheet String(array=w1760, 3:w1764) -> (spreadsheet string=w1766:string)  [unwired: 1 in]
        n440 = Search and Replace String(replace all?=TRUE ("replace all? (F)"), input string=w1766, search string="VgVd", replace string=w1780) -> (result string=w1762:string)  [unwired: 4 in, 3 out]
        n441 = Spreadsheet String To Array(format string=w1764, spreadsheet string=w1762, array type (2D Dbl)=w1760) -> (array=w1761:string[])  [unwired: 1 in]
        n442 = call "4155C Write array to file.vi"("Byte Stream File Refnum"=w1769, "Header"=w1761, "Data Array"=w1786, "error in (no error)"=w1770) -> ("dup refnum"=w1767:refnum<file>, "error out"=w1768:errorcluster)  [unwired: 1 in]
        n443 = Close File(refnum=w1767, error in=w1768) -> (error out=w1754:errorcluster)  [unwired: 1 out]
      }
      frame "resample-fpp" {
        w1849 = string[] ["Time /s", "Id VgVd /A", "Ig VgVd /A", "Vp1 VgVd /V", "Vp2 VgVd /V"] ("Header")
        w1853 = "%d" ("format string")
        n444 = Number To Decimal String(number=w1835) -> (decimal integer string=w1893:string)  [unwired: 1 in]
        n445 = Fract/Exp String To Number(string=w1890) -> (number=w1842:dbl[])  [unwired: 3 in, 1 out]
        n446 = Concatenate Strings(w1886, "-resamplefpp-" ("Substring"), w1893, w1836, ".txt" ("Substring")) -> (w1891:string)
        n447 = String To Path(string=w1891) -> (path=w1861:path)
        n448 = Index Array(array=w1842, index=0 ("Index")) -> (element=w1848:dbl)
        n449 = Index Array(array=w1842, index=1 ("Index")) -> (element=w1847:dbl)
        n450 = Number To Decimal String(number=w1848) -> (decimal integer string=w1871:string)  [unwired: 1 in]
        n451 = call "4155C Take Sample FPP.vi"("VISA resource name in"=w1844, "error in (no error)"=w1843, "Emergency Stop"=w1862) -> ("Time"=w1866:dbl[], "Vp1"=w1876:dbl[], "VISA Resource Name out"=w1846:refnum<visa-resource-name>, "Ig"=w1864:dbl[], "Id"=w1865:dbl[], "Vp2"=w1874:dbl[], "error out"=w1863:errorcluster)  [unwired: 10 in]
        n452 = Insert Into Array(array=dbl[][] [] ("Input Array"), new element=w1866) -> (w1880:dbl[][])  [unwired: 2 in]
        n453 = Number To Decimal String(number=w1847) -> (decimal integer string=w1869:string)  [unwired: 1 in]
        n454 = Insert Into Array(array=w1880, new element=w1865) -> (w1879:dbl[][])  [unwired: 2 in]
        n455 = Concatenate Strings("(Vg = " ("Substring"), w1871, "V, Vd = " ("Substring"), w1869, "V)" ("Substring")) -> (w1867:string)
        n456 = Insert Into Array(array=w1879, new element=w1864) -> (w1878:dbl[][])  [unwired: 2 in]
        n457 = Insert Into Array(array=w1878, new element=w1876) -> (w1875:dbl[][])  [unwired: 2 in]
        n458 = Insert Into Array(array=w1875, new element=w1874) -> (w1841:dbl[][])  [unwired: 2 in]
        n459 = call <vilib>:"compatOverwrite.vi"("overwrite (F)"=TRUE) -> ("overwrite?"=w1840:T8)
        n460 = Open/Create/Replace File(file path (use dialog)=w1861, error in=w1863, operation (0:open)=w1840) -> (refnum out=w1858:refnum<file>, error out=w1859:errorcluster)  [unwired: 3 in, 1 out]
        n461 = Array To Spreadsheet String(array=w1849, 3:w1853) -> (spreadsheet string=w1855:string)  [unwired: 1 in]
        n462 = Transpose 2D Array(2D array=w1841) -> (transposed array=w1873:dbl[][])
        n463 = Search and Replace String(replace all?=TRUE ("replace all? (F)"), input string=w1855, search string="VgVd", replace string=w1867) -> (result string=w1851:string)  [unwired: 4 in, 3 out]
        n464 = Spreadsheet String To Array(format string=w1853, spreadsheet string=w1851, array type (2D Dbl)=w1849) -> (array=w1850:string[])  [unwired: 1 in]
        n465 = call "4155C Write array to file.vi"("Byte Stream File Refnum"=w1858, "Header"=w1850, "Data Array"=w1873, "error in (no error)"=w1859) -> ("dup refnum"=w1856:refnum<file>, "error out"=w1857:errorcluster)  [unwired: 1 in]
        n466 = Close File(refnum=w1856, error in=w1857) -> (error out=w1845:errorcluster)  [unwired: 1 out]
      }
      frame "serial" {
        n467 = local read "Termination char\n(0xA = '\\n' = LF)\n(0xD = '\\r' = CR)"() -> (w1921:u8)
        n468 = local read "Enable Termination\nChar (T)"() -> (w1922:bool)
        n469 = Index Array(array=w1929, index=0 ("Index")) -> (element=w1928:string)
        n470 = local read "parity"() -> (w1912:u16)
        n471 = local read "Delay before read (ms)"() -> (w1923:u32)
        n472 = local read "byte count"() -> (w1920:u32)
        n473 = local read "Timeout (ms)"() -> (w1919:u32)
        n474 = local read "VISA resource name"() -> (w1916:refnum<visa-resource-name>)
        n475 = local read "baud rate"() -> (w1915:u32)
        n476 = local read "Serial End Mode for Reads"() -> (w1914:u16)
        n477 = local read "data bits"() -> (w1913:u16)
        n478 = local read "stop bits"() -> (w1918:u16)
        n479 = local read "flow control"() -> (w1917:u16)
        n480 = call "Serial write and read v0.5.vi"("Delay before read (ms)"=w1923, "Termination char\n(0xA = '\\n' = LF)\n(0xD = '\\r' = CR)"=w1921, "Enable Termination\nChar (T)"=w1922, "parity"=w1912, "stop bits"=w1918, "string to write"=w1928, "flow control"=w1917, "byte count"=w1920, "Serial Settings:Serial End Mode for Reads"=w1914, "Timeout (ms)"=w1919, "error in (no error)"=w1934, "VISA resource name"=w1916, "baud rate"=w1915, "data bits"=w1913) -> ("Serial port output"=w1924:string, "error out"=w1933:errorcluster)
        n481 = Build Array (concatenate)(w1924, w1925) -> (w1926:string[])
      }
      frame "pump" {
        # "Time array for valve position"
        # "Time array for absolute plunger position"
        # "Valve position"
        # "Absolute plunger position"
        # "Remove \"_\""
        # "Check if hard stop is pressed."
        # "Check if halt is pressed."
        # "Check if pump is idle. Else halt."
        n482 = Index Array(array=w1999, index=0 ("Index")) -> (element=w1976:string)
        n483 = case shown="\"No error\", Default" w1974 {
          tunnel: w1976 -> [w2035 _ w2037 w2038 w2039 w2040 _ _ w2043 w2044 _]
          tunnel: [w2035 "/1H" w2037 w2038 w2039 w2040 "/1H" "/1H" w2043 w2044 "/1H"] -> w1975
          frame "No error", Default {
          }
          frame "Initialization" {
          }
          frame "Invalid command" {
          }
          frame "Invalid operand" {
          }
          frame "Device not initialized" {
          }
          frame "Internal failure" {
          }
          frame "Plunger overload" {
          }
          frame "Valve overload" {
          }
          frame "Plunger move not allowed" {
          }
          frame "A/D converter failure" {
          }
          frame "Command overflow" {
          }
        }
        n484 = local read "Hard stop pump"() -> (w1978:bool)
        n485 = local read "Halt pump"() -> (w1981:bool)
        n486 = local read "Serial End Mode for Reads"() -> (w1987:u16)
        n487 = local read "flow control"() -> (w1990:u16)
        n488 = local read "stop bits"() -> (w1991:u16)
        n489 = local read "parity"() -> (w1985:u16)
        n490 = local read "Delay before read (ms)"() -> (w1996:u32)
        n491 = local read "byte count"() -> (w1993:u32)
        n492 = local read "Timeout (ms)"() -> (w1992:u32)
        n493 = local read "VISA resource name"() -> (w1989:refnum<visa-resource-name>)
        n494 = local read "baud rate"() -> (w1988:u32)
        n495 = local read "Enable Termination\nChar (T)"() -> (w1995:bool)
        n496 = local read "Termination char\n(0xA = '\\n' = LF)\n(0xD = '\\r' = CR)"() -> (w1994:u8)
        n497 = case shown="True" w1981 {
          tunnel: [w2049 "/1H"] -> w1980
          tunnel: w1975 -> [w2049 _]
          frame False {
          }
          frame True {
            n498 = local write "Halt pump"(FALSE) -> ()
          }
        }
        n499 = case shown="True" w1978 {
          tunnel: [w2046 "/1T"] -> w1979
          tunnel: w1980 -> [w2046 _]
          frame False {
          }
          frame True {
            n500 = local write "Hard stop pump"(FALSE) -> ()
          }
        }
        n501 = local read "data bits"() -> (w1986:u16)
        n502 = String Subset(string=w1970, offset (0)=1) -> (substring=w1968:string)  [unwired: 1 in]
        n503 = call "SPM Pump v0.6.vi"("Termination char\n(0xA = '\\n' = LF)\n(0xD = '\\r' = CR)"=w1994, "Enable Termination\nChar (T)"=w1995, "Timeout (ms)"=w1992, "Serial Settings:Serial End Mode for Reads"=w1987, "byte count"=w1993, "Delay before read (ms)"=w1996, "Time <input>"=w1973, "error in (no error)"=w2004, "Serial port input"=w1979, "VISA resource name"=w1989, "parity"=w1985, "baud rate"=w1988, "stop bits"=w1991, "data bits"=w1986, "flow control"=w1990, "Time units <input>"=w1968) -> ("Input command"=w1967:string, "Serial port data"=w1957:string[], "Pump status"=w1963:string, "Valve position"=w1965:i32, "Absolute plunger position"=w1977:i32, "Serial port"=w1972:string, "error out"=w2003:errorcluster)  [unwired: 1 in, 4 out]
        n504 = case shown="\"?6\"" w1967 {
          tunnel: [w2016 w2024 w2030] -> w1984
          tunnel: w1983 -> [w2016 w2023 w2030]
          tunnel: w1977 -> [_ w2022 _]
          tunnel: w1964 -> [w2015 w2021 w2031]
          tunnel: [w2015 w2021 w2033] -> w1966
          tunnel: w1965 -> [_ _ w2032]
          tunnel: w1962 -> [_ w2020 w2028]
          tunnel: w1961 -> [w2014 w2019 w2029]
          tunnel: [w2014 w2018 w2029] -> w1960
          tunnel: [w2013 w2017 w2027] -> w1959
          tunnel: w1958 -> [w2013 w2017 w2026]
          frame "Q", Default {
          }
          frame "?" {
            n505 = Build Array (concatenate)(w2023, w2022) -> (w2024:i32[])
            n506 = Build Array (concatenate)(w2019, w2020) -> (w2018:i32[])
            n507 = call "4155C Split array.vi"("X data in"=w2018, "Y1 data in"=w2024) -> ("Array of clusters"=w2025:cluster{"Y data in":dbl[], "X data in":dbl[]}[])  [unwired: 5 in, 1 out]
            n508 = local write "Absolute plunger position vs time"(w2025) -> ()
          }
          frame "?6" {
            n509 = Build Array (concatenate)(w2031, w2032) -> (w2033:i32[])
            n510 = Build Array (concatenate)(w2026, w2028) -> (w2027:i32[])
            n511 = call "4155C Split array.vi"("X data in"=w2027, "Y1 data in"=w2033) -> ("Array of clusters"=w2034:cluster{"Y data in":dbl[], "X data in":dbl[]}[])  [unwired: 5 in, 1 out]
            n512 = local write "Valve position vs time"(w2034) -> ()
          }
        }
        n513 = Build Array (concatenate)(w1955, w1957) -> (w1956:string[][])
        n514 = Build Array (concatenate)(w1971, w1972) -> (w1997:string[])
      }
      frame "filename" {
        n515 = Index Array(array=w2053, index=0 ("Index")) -> (element=w2052:string)
      }
    }
    n516 = local read "Time Units"() -> (w65:u16)
    n517 = case shown="2" w65 {
      tunnel: ["Time (Seconds)" ("element") "Time (Minutes)" ("element") "Time (Hours)" ("element")] -> w105
      frame 0 {
      }
      frame 1, Default {
      }
      frame 2 {
      }
    }
    n518 = Build Array(w144, w73, w83, w82, w81, w80, w79, w78, w77, w76, w75, w74, w72) -> (w183:dbl[][])
    n519 = Transpose 2D Array(2D array=w183) -> (transposed array=w182:dbl[][])
    n520 = Concatenate Strings(w124, w67, "Imax_Imin_Ion_Ioff_vs_time.txt" ("Suffix (Imax,Imin,Ion,Ioff)")) -> (w193:string)
    n521 = Build Array(w105, "Is max (A)" ("VAR2 Name"), "Is min (A)" ("VAR2 Name"), "Id max (A)" ("VAR2 Name"), "Id min (A)" ("VAR2 Name"), "Ig max (A)" ("VAR2 Name"), "Ig min (A)" ("VAR2 Name"), "Is on (A)" ("VAR2 Name"), "Is off (A)" ("VAR2 Name"), "Id on (A)" ("VAR2 Name"), "Id off (A)" ("VAR2 Name"), "Ig on (A)" ("VAR2 Name"), "Ig off (A)" ("VAR2 Name")) -> (w188:string[])
    n522 = Array To Spreadsheet String(array=w182, 3:"%e" ("format string")) -> (spreadsheet string=w186:string)  [unwired: 1 in]
    n523 = Array To Spreadsheet String(array=w188, 3:"" ("format string")) -> (spreadsheet string=w187:string)  [unwired: 1 in]
    n524 = String To Path(string=w193) -> (path=w192:path)
    n525 = Build Array(w187, w186) -> (w185:string[])
    n526 = Write to Text File(file (use dialog)=w192, text=w185, error in=w140) -> (refnum out=w194:refnum<file>, error out=w184:errorcluster)  [unwired: 1 in, 1 out]
    n527 = Close File(refnum=w194, error in=w184) -> (error out=w123:errorcluster)  [unwired: 1 out]
    n528 = Build Array(w119, w145) -> (w150:i32[][])
    n529 = Build Array(w105, "Absolute plunger position" ("VAR2 Name")) -> (w153:string[])
    n530 = Transpose 2D Array(2D array=w150) -> (transposed array=w143:i32[][])
    n531 = Array To Spreadsheet String(array=w153, 3:"" ("format string")) -> (spreadsheet string=w152:string)  [unwired: 1 in]
    n532 = Array To Spreadsheet String(array=w143, 3:"%e" ("format string")) -> (spreadsheet string=w149:string)  [unwired: 1 in]
    n533 = Build Array(w152, w149) -> (w155:string[])
    n534 = Concatenate Strings(w124, w67, "plunger_vs_time.txt" ("Suffix (plunger)")) -> (w147:string)
    n535 = String To Path(string=w147) -> (path=w146:path)
    n536 = Write to Text File(file (use dialog)=w146, text=w155, error in=w123) -> (refnum out=w148:refnum<file>, error out=w157:errorcluster)  [unwired: 1 in, 1 out]
    n537 = Close File(refnum=w148, error in=w157) -> (error out=w122:errorcluster)  [unwired: 1 out]
    n538 = Concatenate Strings(w124, w67, "serial_port_output.txt" ("Suffix (serial port log)")) -> (w163:string)
    n539 = String To Path(string=w163) -> (path=w162:path)
    n540 = Build Array(w105, "Serial port input" ("VAR2 Name"), "Pump status" ("VAR2 Name"), "Serial port output: ") -> (w109:string[])
    n541 = Array To Spreadsheet String(array=w115, 3:"" ("format string")) -> (spreadsheet string=w106:string)  [unwired: 1 in]
    n542 = Array To Spreadsheet String(array=w109, 3:"" ("format string")) -> (spreadsheet string=w107:string)  [unwired: 1 in]
    n543 = Build Array(w107, w106) -> (w108:string[])
    n544 = Array To Spreadsheet String(array=w114, 3:"" ("format string")) -> (spreadsheet string=w168:string)  [unwired: 1 in]
    n545 = Write to Text File(file (use dialog)=w162, text=w108, error in=w122) -> (refnum out=w164:refnum<file>, error out=w165:errorcluster)  [unwired: 1 in, 1 out]
    n546 = Close File(refnum=w164, error in=w165) -> (error out=w121:errorcluster)  [unwired: 1 out]
    n547 = local write "Serial port data"(w168) -> ()
    n548 = Build Array(w118, w126) -> (w132:i32[][])
    n549 = Build Array(w105, "Valve port" ("VAR2 Name")) -> (w135:string[])
    n550 = Transpose 2D Array(2D array=w132) -> (transposed array=w127:i32[][])
    n551 = Array To Spreadsheet String(array=w135, 3:"" ("format string")) -> (spreadsheet string=w134:string)  [unwired: 1 in]
    n552 = Array To Spreadsheet String(array=w127, 3:"%e" ("format string")) -> (spreadsheet string=w131:string)  [unwired: 1 in]
    n553 = Build Array(w134, w131) -> (w137:string[])
    n554 = Concatenate Strings(w124, w67, "valve_port_vs_time.txt" ("Suffix (valve)")) -> (w129:string)
    n555 = String To Path(string=w129) -> (path=w128:path)
    n556 = Write to Text File(file (use dialog)=w128, text=w137, error in=w121) -> (refnum out=w130:refnum<file>, error out=w139:errorcluster)  [unwired: 1 in, 1 out]
    n557 = Close File(refnum=w130, error in=w139) -> (error out=w120:errorcluster)  [unwired: 1 out]
  }
  "error out" <- w28
  "Timings Indicator" <- w10
  "Is max" <- w8
  "Id max" <- w8
  "Ig max" <- w8
  "Imax vs time" <- w4
  "I vs Vg" <- w4
  "Imin vs time" <- w4
  "I vs Vd" <- w4
  "Serial port data" <- "" ("Serial port data")
  "Valve position vs time" <- cluster{"Y data in":dbl[], "X data in":dbl[]}[] [] ("Valve position vs time")
  "Is min" <- w7
  "Id min" <- w7
  "Ig min" <- w7
  "Ion vs time" <- w4
  "Ioff vs time" <- w4
  "Is on" <- w6
  "Id on" <- w6
  "Ig on" <- w6
  "Is off" <- w5
  "Id off" <- w5
  "Ig off" <- w5
